vi "MIX11.1Eng.vi"() -> ()   [LabVIEW 2017]
uses:
  <vilib>/Utility/NIReport.llb/NI_report.lvclass
  <vilib>/Utility/NIReport.llb/Excel/NI_Excel.lvclass
  Instance           1 13Saved   MIX10 .vi
  Instance           5 13Saved   MIX10 .vi
  <vilib>/Utility/file.llb/Write To Spreadsheet File (string).vi
  <vilib>/Utility/file.llb/Read From Spreadsheet File (string).vi
  Instance           6 13Saved   MIX10 .vi
  <vilib>/Utility/NIReport.llb/Append Report Text (str wrap).vi
  <vilib>/Utility/NIReport.llb/Append Text Table to Report (wrap).vi
  Instance           4 13Saved   MIX10 .vi
  Instance           2 13Saved   MIX10 .vi
panel:
  in  "SP_Spurious":cluster{"Rx_output_data":path, "SAVE":bool}={"Rx_output_data"=path "L:/cartridge/assembly/SN03/03-23/111227_DSB/SP_810.00_120_111227_CCA03-23_DSBFB.csv", "SAVE"=TRUE}
  in  "report":refnum<class "NI_report.lvclass">=refnum
  in  "Offset":dbl
  in  "WCA Pol":u16(ring) items=["------------"=444, "WCA P0 S1"=0, "WCA P0 S2"=2, "WCA P1 S1"=1, "WCA P1 S2"=3]
  in  "VMax":dbl=5.0
  in  "Vmin":dbl
  out "VP Class":cluster{"”z—ñ":dbl[], "”z—ñ 2":dbl[]}={"”z—ñ"=[-1.0620880126953125, -1.0097503662109375, -0.9580230712890625, -0.9108734130859375, -0.8547210693359375, -0.803070068359375, -0.7555389404296875, -0.71075439453125, -0.659027099609375, -0.6090545654296875, -0.5593109130859375, -0.5091094970703125, -0.4544830322265625, -0.405120849609375, -0.3562164306640625, -0.3061676025390625, -0.25177001953125, -0.2005767822265625, -0.1529693603515625, -0.0995635986328125, -0.0360870361328125, 0.0032806396484375, 0.0568389892578125, 0.1003265380859375, 0.1499176025390625, 0.201416015625, 0.2490234375, 0.2971649169921875, 0.3517913818359375, 0.3971099853515625, 0.447845458984375, 0.4936981201171875, 0.5454254150390625, 0.59356689453125, 0.643768310546875, 0.6946563720703125, 0.7459259033203125, 0.7933807373046875, 0.8406829833984375, 0.8930206298828125, 0.94207763671875], "”z—ñ 2"=[0.0, 0.0, 0.0, 0.0, 0.0, 0.0, 0.0, 0.0, 0.0, 0.0, 0.0, 0.0, 0.0, 0.0, 0.0, 0.0, 0.0, 0.0, 0.0, 0.0, 0.0, 0.0, 0.0, 0.0, 0.0, 0.0, 0.0, 0.0, 0.0, 0.0, 0.0, 0.0, 0.0, 0.0, 0.0, 0.0, 0.0, 0.0, 0.0, 0.0, 0.0]}
  out "VI Class":cluster{"”z—ñ":dbl[], "”z—ñ 2":dbl[]}={"”z—ñ"=[-1.0620880126953125, -1.0097503662109375, -0.9580230712890625, -0.9108734130859375, -0.8547210693359375, -0.803070068359375, -0.7555389404296875, -0.71075439453125, -0.659027099609375, -0.6090545654296875, -0.5593109130859375, -0.5091094970703125, -0.4544830322265625, -0.405120849609375, -0.3562164306640625, -0.3061676025390625, -0.25177001953125, -0.2005767822265625, -0.1529693603515625, -0.0995635986328125, -0.0360870361328125, 0.0032806396484375, 0.0568389892578125, 0.1003265380859375, 0.1499176025390625, 0.201416015625, 0.2490234375, 0.2971649169921875, 0.3517913818359375, 0.3971099853515625, 0.447845458984375, 0.4936981201171875, 0.5454254150390625, 0.59356689453125, 0.643768310546875, 0.6946563720703125, 0.7459259033203125, 0.7933807373046875, 0.8406829833984375, 0.8930206298828125, 0.94207763671875], "”z—ñ 2"=[-8.428955078125, -7.815551757812501, -7.476806640625, -7.16552734375, -6.5887451171875, -6.0546875, -5.7098388671875, -5.682373046875, -5.18798828125, -4.4708251953125, -4.45556640625, -4.150390625, -3.375244140625, -3.167724609375, -2.40478515625, -2.4810791015625, -1.9561767578124998, -1.5899658203125, -1.0498046875, -0.4425048828125, -0.3448486328125, -0.0732421875, 0.1373291015625, 0.5889892578125, 1.1199951171875, 1.2298583984375, 1.715087890625, 1.9439697265625, 2.5054931640625, 2.9205322265625, 3.4698486328125, 3.50341796875, 3.96728515625, 4.2327880859375, 4.656982421875, 4.7698974609375, 5.230712890625, 5.7342529296875, 5.9234619140625, 6.439208984375, 6.9610595703125]}
  out "XY graph":cluster{dbl[], dbl[]}[](graph)=[{[0.9882354736328125], [1.4178466983139515]}, {[0.9882354736328125], [0.0]}, {[-1.0620880126953125, -1.0097503662109375, -0.9580230712890625, -0.9108734130859375, -0.8547210693359375, -0.803070068359375, -0.7555389404296875, -0.71075439453125, -0.659027099609375, -0.6090545654296875, -0.5593109130859375, -0.5091094970703125, -0.4544830322265625, -0.405120849609375, -0.3562164306640625, -0.3061676025390625, -0.25177001953125, -0.2005767822265625, -0.1529693603515625, -0.0995635986328125, -0.0360870361328125, 0.0032806396484375, 0.0568389892578125, 0.1003265380859375, 0.1499176025390625, 0.201416015625, 0.2490234375, 0.2971649169921875, 0.3517913818359375, 0.3971099853515625, 0.447845458984375, 0.4936981201171875, 0.5454254150390625, 0.59356689453125, 0.643768310546875, 0.6946563720703125, 0.7459259033203125, 0.7933807373046875, 0.8406829833984375, 0.8930206298828125, 0.94207763671875], [-8.428955078125, -7.815551757812501, -7.476806640625, -7.16552734375, -6.5887451171875, -6.0546875, -5.7098388671875, -5.682373046875, -5.18798828125, -4.4708251953125, -4.45556640625, -4.150390625, -3.375244140625, -3.167724609375, -2.40478515625, -2.4810791015625, -1.9561767578124998, -1.5899658203125, -1.0498046875, -0.4425048828125, -0.3448486328125, -0.0732421875, 0.1373291015625, 0.5889892578125, 1.1199951171875, 1.2298583984375, 1.715087890625, 1.9439697265625, 2.5054931640625, 2.9205322265625, 3.4698486328125, 3.50341796875, 3.96728515625, 4.2327880859375, 4.656982421875, 4.7698974609375, 5.230712890625, 5.7342529296875, 5.9234619140625, 6.439208984375, 6.9610595703125]}, {[-1.0620880126953125, -1.0097503662109375, -0.9580230712890625, -0.9108734130859375, -0.8547210693359375, -0.803070068359375, -0.7555389404296875, -0.71075439453125, -0.659027099609375, -0.6090545654296875, -0.5593109130859375, -0.5091094970703125, -0.4544830322265625, -0.405120849609375, -0.3562164306640625, -0.3061676025390625, -0.25177001953125, -0.2005767822265625, -0.1529693603515625, -0.0995635986328125, -0.0360870361328125, 0.0032806396484375, 0.0568389892578125, 0.1003265380859375, 0.1499176025390625, 0.201416015625, 0.2490234375, 0.2971649169921875, 0.3517913818359375, 0.3971099853515625, 0.447845458984375, 0.4936981201171875, 0.5454254150390625, 0.59356689453125, 0.643768310546875, 0.6946563720703125, 0.7459259033203125, 0.7933807373046875, 0.8406829833984375, 0.8930206298828125, 0.94207763671875], [0.0, 0.0, 0.0, 0.0, 0.0, 0.0, 0.0, 0.0, 0.0, 0.0, 0.0, 0.0, 0.0, 0.0, 0.0, 0.0, 0.0, 0.0, 0.0, 0.0, 0.0, 0.0, 0.0, 0.0, 0.0, 0.0, 0.0, 0.0, 0.0, 0.0, 0.0, 0.0, 0.0, 0.0, 0.0, 0.0, 0.0, 0.0, 0.0, 0.0, 0.0]}]
  in  "Controller":T1(tab)=enum."revision"
  in  "CAN reset":bool
  out "Connected":bool
  in  "DISConnect":bool
  in  "Connect":bool
  in  "Bias_LO_equip":T2={"Node address"=19, "CAN Interface"="CAN0", "Cartridge band"=8, "Slave Node in"={"Address"=19, "Serial Number"=[16, 121, 69, 76, 1, 8, 0, -31]}, "ObjHandle out"=26, "POL"=0, "sb"=1, "GPIB_SM (SIS S,V)"="24", "GPIB_DMM (SIS I)"="22", "GPIB_SM (MAG I) "="25", "GPIB_SG(LO)"="19", "GPIB_PW (PAMP) "="6", "GPIB_TMP1(8ch)"="12", "GPIB_TMP2(2ch)"="13", "WCA_avg"=10, "Rsen"=10.0, "BiasModule"=1, "LOModule "=2, "WCA_LO_FREQ_SET"={"YTO Low freq. [GHz]"=14.65, "YTO High freq. [GHz]"=17.5, "Kvco"=1, "Lock Pol."=0, "SET LO FREQ"=88.77778, "Multiplier"=6.0, "YTO (HEX)"=210, "YTO ( FREQ)"=14.796153, "NULL PLL INTEGRATOR"=TRUE}, "Res for"=0} {"Res for" items=["none", "series res", "parallel res"]; "WCA_LO_FREQ_SET"."YTO ( FREQ)" min=25 max=150 step=0.0001 format="%.3f"; "WCA_LO_FREQ_SET"."Multiplier" min=3 max=6 step=3; "WCA_LO_FREQ_SET"."SET LO FREQ" min=25 max=150 step=0.0001 format="%.3f"; "WCA_LO_FREQ_SET"."Lock Pol." items=["Lower", "Upper"]; "WCA_LO_FREQ_SET"."Kvco" items=["7.5MHz/V", "15MHz/V"]; "WCA_LO_FREQ_SET"."YTO High freq. [GHz]" format="%.3f"; "WCA_LO_FREQ_SET"."YTO Low freq. [GHz]" format="%.3f"; "BiasModule" items=["B10Lab Bias"=0, "WCA BiasModule"=1, "none"=99, "SM-4W"=2]; "Slave Node in"."Serial Number" format="%.0x"; "Slave Node in"."Address" format="%.0x"; "Cartridge band" max=10 step=1; "Node address" format="%.0x"}
  in  "Control":T3={"GPIB_ATT"="28", "6501Dev#"=1, "GPIB_SpecA"="18", "GPIB_PM"="13", "GPIB_DSA"="11", "GPIB_DMM (TPD)"="23", "MPI COM"="COM5", "motor setting"=[{"Axis"=0, "ID"=0, "HIspeed"=200.0, "LOspeed"=100.0, "ACCEL(ms)"=100.0, "Sratio"=50.0, "free run\n"=FALSE, "motor"="DSB HOT/COLD"}, {"Axis"=1, "ID"=0, "HIspeed"=4.0, "LOspeed"=4.0, "ACCEL(ms)"=100.0, "Sratio"=50.0, "free run\n"=TRUE, "motor"="SubMM Att"}, {"Axis"=0, "ID"=0, "HIspeed"=200.0, "LOspeed"=100.0, "ACCEL(ms)"=100.0, "Sratio"=50.0, "free run\n"=FALSE, "motor"="MPI Port1"}, {"Axis"=1, "ID"=0, "HIspeed"=200.0, "LOspeed"=100.0, "ACCEL(ms)"=100.0, "Sratio"=50.0, "free run\n"=FALSE, "motor"="MPI Port2"}, {"Axis"=1, "ID"=0, "HIspeed"=200.0, "LOspeed"=100.0, "ACCEL(ms)"=100.0, "Sratio"=50.0, "free run\n"=TRUE, "motor"="gainComp"}], "DATA path"=path "C:/", "mixer param file "=path "C:/", "comment"="150115_balanced_WCA_2", "Carteidge SN"="balanced150115", "Th"=297.0, "Tc"=77.0, "Set_SIS_volt"=1.0483870967741935, "Offset"=0.0, "control"=0, "FreqLO"=799.0, "Set_Mag_Cur"=0.0, "MPI offset(mm)"=23.203, "HOT/COLD"=0} {"HOT/COLD" items=["DSB", "SBR (Cart.)"]; "control" items=["CLOSE LOOP", "OPEN LOOP", "Not Control"]}
  in  "Additional Cartridge band":u32=10 max=10 step=1
  in  "add":bool
  in  "CLNA_SET":T4 {"SET POL0 LNA1 STAGE3 DRAIN C" min=0 max=20 step=0.01 format="%.2f"; "SET POL0 LNA1 STAGE3 DRAIN V" min=0 max=3 step=0.01 format="%.2f"; "SET POL0 LNA1 STAGE2 DRAIN C" min=0 max=20 step=0.01 format="%.2f"; "SET POL0 LNA1 STAGE2 DRAIN V" min=0 max=3 step=0.01 format="%.2f"; "SET POL0 LNA1 STAGE1 DRAIN C" min=0 max=20 step=0.01 format="%.2f"; "SET POL0 LNA1 STAGE1 DRAIN V" min=0 max=3 step=0.01 format="%.2f"; "CLNA State" items=["Disabled", "Enabled"]}
  out "CLNA_monitor":T5={"Pol0 LNA1 S1 Drain V [V]"=0.0017700195, "Pol0 LNA1 S1 Drain C [mA]"=0.0033569336, "Pol0 LNA1 S1 Gate V [V]"=-0.3663025, "Pol0 LNA1 S2 Drain V [V]"=0.0020446777, "Pol0 LNA1 S2 Drain C [mA]"=0.0010681152, "Pol0 LNA1 S2 Gate V [V]"=4.9404297, "Pol0 LNA1 S3 Drain V [V]"=0.0019989014, "Pol0 LNA1 S3 Drain C [mA]"=0.024871826, "Pol0 LNA1 S3 Gate V [V]"=4.940445, "Pol0 LNA1 State"=enum."Disabled"} {"Pol0 LNA1 S3 Gate V [V]" format="%.2f"; "Pol0 LNA1 S3 Drain C [mA]" format="%.2f"; "Pol0 LNA1 S3 Drain V [V]" format="%.2f"; "Pol0 LNA1 S2 Gate V [V]" format="%.2f"; "Pol0 LNA1 S2 Drain C [mA]" format="%.2f"; "Pol0 LNA1 S2 Drain V [V]" format="%.2f"; "Pol0 LNA1 S1 Gate V [V]" format="%.2f"; "Pol0 LNA1 S1 Drain C [mA]" format="%.2f"; "Pol0 LNA1 S1 Drain V [V]" format="%.2f"}
  in  "CLNA Monitor":bool=TRUE
  in  "Set CLNA":bool
  in  "Temp Monitor":bool=TRUE
  out "T3":dbl=-1.0
  out "T2":dbl=296.31982421875
  out "T1":dbl=-1.0
  in  "CLNAsweep":T6={"VDmin"=1.0, "VDmax"=2.0, "VDstep"=0.1, "IDmin"=8.0, "IDmax"=20.0, "IDstep"=1.0, "wait (mS)"=500.0, "P.M.aveg"=10, "HOT/COLD "=0, "SIS hotV "=8.0, "SIS coldV"=5.0, "file_name"="", "frq(GHz)"=8.0} {"HOT/COLD" items=["Liq Ni Motor", "SISBias"]}
  in  "CLNA Sweep":bool
  in  "Do shapiro":bool
  in  "Heater@ON@":bool
  in  "Do Demag":bool
  in  "Ic measurement":bool
  in  "demag":T7={"Start(mA)"=100.0, "Time(ms)"=200.0, "step"=1.0}
  in  "Joseph_curr":T8={"start(mA)"=8.5, "stop(mA)"=10.0, "step(mA)"=0.1, "file_name"="", "file path"=path "", "save?"=FALSE, "SIS Bias range Vsis"={"start"=-0.1, "stop"=0.1, "step"=0.02}}
  in  "Magnet Current Set":dbl(slide) scale=10.0..30.0
  in  "Mag Monitor":bool=TRUE
  out "Mag V":dbl=0.8539886474609375
  out "Mag C":dbl=26.22833251953125
  in  "shapiro":T9={"start(mA)"=8.5, "stop(mA)"=10.0, "step(mA)"=0.05, "start(mV)"=1.2, "stop(mV)"=2.4, "step(mV)"=0.05, "file_name"="", "path"=path "", "save?"=FALSE}
  in  "SIS_Deflux_heater":T10={"ON start time (ms)"=3000.0, "ON duration time (ms)"=10000.0, "Measurement end time"=60000.0, "SIS Volt (mV)"=0.5, "GPIB_PW (SISHeater) "="3", "SAVE"=TRUE, "file_name"="", "path"=path "Z:/band10/Labview_ALMA/MIX95/test"}
  in  "SISparam":bool
  in  "Zero Int":bool
  in  "Set LO PAMP":bool
  in  "WCA_LO monitor":bool=TRUE
  in  "LO_misc":T11={"LO FRQ(GHz)"=799.0, "LO multi "=9.0, "LocK?"=FALSE, "LO REF multi"=3.0, "wait (ms)"=100.0, "SG Pow Min (dBm)"=0.0, "SG Pow Max (dBm)"=20.0, "SG Pow Step (dBm)"=0.2, "SGPow OPT? "=TRUE, "SG set frq"=0.0, "SG set pow"=0.0}
  in  "Set LO freq":bool
  out "GET_PA":T12={"PA_A_DRAIN_V"=0.009918213, "PA_A_DRAIN_C"=2.4871826, "PA_A_GATE_V"=0.0016784668, "PA_B_DRAIN_V"=0.0077819824, "PA_B_DRAIN_C"=2.8533936, "PA_B_GATE_V"=0.004272461, "PA_3V_SUPPLY_V"=2.992859, "PA_5V_MON"=5.2355957}
  out "GET_PLL":T13={"PLL_ASSY_T"=29.312134, "PLL_REF_TOT_P"=-0.02670288, "PLL_IF_TOT_P"=-0.036315918, "PLL_CORR_V"=-3.8926976, "PLL_LOCK_V"=0.05389127, "PLL_5V_SUPPLY_V"=25.061035, "Temp_TF"=TRUE, "PLL Ref Pwr_TF"=FALSE, "IF Pwr_TF"=FALSE, "PLL Corr_TF"=FALSE, "PLL Lock V_TF"=FALSE, "PLL Nominal_TF"=FALSE}
  in  "PA V":cluster{"VD":dbl, "VG ":dbl, "String":string}[](array[cluster])=[{"VD"=0.0, "VG "=-0.4, "String"="WCA P0"}, {"VD"=0.0, "VG "=0.0, "String"="WCA P1"}, {"VD"=0.0, "VG "=0.0, "String"="B10 PAMP"}] {"VG" min=-1.0 max=4.0; "VD" min=0.0 max=2.5}
  in  "_LO_P_OPT":T14={"Range Array"=[{"Start"=0.0, "Stop"=3.5, "Step"=0.1, "By"="NEL VG"}, {"Start"=30.0, "Stop"=75.0, "Step"=1.0, "By"="Motor"}, {"Start"=0.5, "Stop"=2.0, "Step"=0.05, "By"="WCA VD"}], "Optimize"=0, "file_name"="LP_914.0_Tmin_100519.csv", "Save?"=FALSE, "measure"=2, "current(uA)"=40.0, "wait(ms)"=0, "IFfrq(GHz)"=8.0, "aveg"=10, "SISparam option"=0} {"SISparam option" items=["Volt and Current", "Volt only"]; "measure" items=["Pmax (only HOT)", "Tmin (HOT/COLD)", "C current"]; "Optimize" items=["Sweep", "‰©‹à•ªŠ„"]; "Range Array"."Step" format="%.2f"; "Range Array"."Stop" format="%.2f"; "Range Array"."Start" format="%.2f"}
  in  "LOP optimize":bool
  in  "_LO_sweep":T15={"scales"=200.0, "start (GHz)"=780.0, "stop (GHz)"=960.0, "step (GHz) "=0.1, "Wait(ms)"=10.0, "file_name"="", "path"=path "", "measure"=0, "WCA Pol"=0} {"WCA Pol" items=["------------"=444, "WCA P0 S1"=0, "WCA P0 S2"=2, "WCA P1 S1"=1, "WCA P1 S2"=3]; "measure" items=["SIS Current", "DMM34401A"]}
  in  "LO_SWEEP":bool
  in  "IFBOX":T16={" Output"=2, "YIG Fc(GHz)"=8.0, " Filter"=3, "Input"=2} {"Input" items=["1:Pol 0"=1, "2:Pol 1"=2, "3:dummy"=3, "4:NoiseSource"=4]; "Filter" items=["1:YIG"=1, "2:direct"=2, "3:4-12BPF"=3, "4:direct 4-12BPF"=4]; "Output" items=["1:Speana"=1, "2:PowerMeter"=2, "3:dummy"=3, "4:TPD"=4]}
  in  "I-V sweep":bool
  in  "i-v parameter":T17={"start(mV)"=0.0, "stop(mV)"=3.0, "step(mV)"=0.05, "file_name"="", "IF OFF/ON"=FALSE, "SAVE OFF/ON"=FALSE, "frq(GHz)"=8.0, "avg"=1, "number of Sweep  "=0, "VminfromSS"=0.15, "mode "=0, "V@opt"=2} {"mode" items=["voltage sweep", "every time HOT/COLD"]; "number of Sweep" items=["only once", "Hot/Cold_auto", "Hot/Cold manual"]}
  out "HOT":bool
  in  "HOT/COLD":bool=TRUE
  in  "IFBOXSet":bool
  in  "CrossTalk_mkpk":T18={"save"=TRUE, "file_name"="", "IF start"=4.0, "IF stop"=12.0, "IF step"=1.0}
  in  "CrossTalk":bool
  in  "GainComp":bool
  in  "GC_LockinAmp":T19={"GPIB"="28", "wait(s)"=10.0, "measure(s) "=30.0, "save"=FALSE, "time constant"=6, "file_name"=""} {"time constant" items=["100mS"=5, "300mS"=6, "1S"=7, "3S"=8, "10S"=9]}
  in  "allan":T20={"DMM Setting A"={"interval"=1.0, "sample number"=5000, "Voltage Range"=enum."1 V", "Factor"=1.0, "unit"=0, "Power supply freq. (Hz)"=50.0}, "Path"=path "c:/Data", "File name"="", "DMM"=0, "DSA_mes"={"GPIB_DSA"="11", "Startfrq(Hz)"=0.0, "Stopfrq(Hz)"=800.0, "Range(Vpk)"=1.0, "average"=4}, " temperature?"=TRUE, "time interval"=10.0} {"DMM" items=["DMM34410A", "34401A", "3458", "DSA35670A"]; "DMM Setting A"."unit" items=["Sec", "PLC"]; "DMM Setting A"."sample number" min=1 max=1000000 step=1}
  in  "Start allan":bool
  in  "LO harmonic":T21={"save"=TRUE, "file_name"="", "LO start"=890.0, "LO stop"=938.0, "LO step"=8.0, "IF"=5.0, "8th 10th"=TRUE}
  in  "LO Harmonic":bool
  in  "spectrum_data":T22={"total data num(1-3)"=2, "file_name"="", "SAVE OFF/ON"=FALSE, "ATT1"=0.0, "ATT2"=2.0, "SNAdatafile ATT1"=path "C:/Documents and Settings/band10/デスクトップ/Labview_ALMA/MIX99/101210_ATT/ATT0db.prn", "SNAdatafile ATT2"=path "C:/Documents and Settings/band10/デスクトップ/Labview_ALMA/MIX99/101210_ATT/ATT2db.prn", "ATTcal"=FALSE, "SP_set"={"start(GHz)"=3.5, "stop(GHz) "=12.5, "BW(MHz)"=8.0, "VBW(Hz)"=30.0, "ref(dBm)"=-50.0, "log(dB)"=1.0, "AVEG"=1, "AVEG ON/OFF"=FALSE, "Auto Align ON/OFF"=FALSE, "GPIB"="18", "point"=1126}, "HOT/COLD"=1} {"HOT/COLD" items=["Manual", "Motor auto", "SIS V", "P0/P1", "single data"]}
  in  "SPmeasuremnt":bool
  in  "Noise_YIG_tune_filter_control":T23={"Start(GHz)"=4.0, "Stop(GHz)"=12.0, "Step(GHz) "=0.1, "wait (S)"=0.0, "Hot/Cold Switch"=1, "file_name"="", "P.M.aveg"=10, "save"=TRUE} {"Hot/Cold Switch" items=["Liq Ni Motor", "NoiseSource Pow", "NoiseSource SP4T SW"]}
  in  "YIG measurement":bool
  in  "RF":bool
  in  "Move MPI toSSB":bool
  in  "IF frequency to SSB":dbl=4.0 format="%#.5g"
  in  "SBR":bool
  out "MPI present location":string="22.99999\r\n"
  in  "MPI pos":dbl=23.0 format="%#.5g"
  in  "MPI-I":bool
  in  "MPI_I":T24={"wait(ms)"=300, "Start"=22.5, "Stop"=23.5, "Step"=0.005, "save"=TRUE, "file_name"=""} {"Step" format="%#.6f"; "Stop" format="%.2f"; "Start" format="%.2f"}
  in  "Move MPI":bool
  in  "SBR_Set":T25={"file_name"="", "HOT/COLD AUTO"=TRUE, "MPI SSB Set"=TRUE, "Waiting time at AUTO(S)"=0.1, "P/V         V/P"=TRUE, "save"=TRUE, "start(GHz)"=4.0, "stop(GHz) "=12.0, "Step(GHz) "=0.5, "P.M.aveg"=10, "PM        SP"=FALSE, "SP_set"={"start(GHz)"=3.5, "stop(GHz) "=12.5, "BW(MHz)"=8.0, "VBW(Hz)"=30.0, "ref(dBm)"=-45.0, "log(dB)"=1.0, "AVEG"=1, "AVEG ON/OFF"=FALSE, "Auto Align ON/OFF"=FALSE, "GPIB"="18", "point"=801}}
  in  "RF":T26={"RF(GHz)"=900.0, "mm_multi(4or6)"=6.0, "SGPOUT(dBm)"=16.0, "SGGPIB"="29", "PAMP GPIB"="6", "VD (V)"=1.0, "VG (V)"=0.0, "multi (V)"=8.0} {"multi (V)" min=0.0 max=15.0 step=0.5; "VG (V)" min=0.0 max=4.0 step=0.1; "VD (V)" min=0.0 max=1.85 step=0.01}
  out "file name":string="mix11_baranced_setmix.txt"
  in  "MOSL":i32
  out "log_refnum":refnum<file>
  in  "Script path":path=path "C:/Labview_ALMA/MIX11/Mixスクリプト"
  in  "?":enum32{"run", "save"}(tab)
  in  "load script":bool
  in  "run script":bool
  in  "save":bool
  in  "program":cluster{"Cord":u16, "Option":string}[](array[cluster])=[{"Cord"=1, "Option"="auto measurement By WCA LO 2Pol"}, {"Cord"=16, "Option"=""}, {"Cord"=130, "Option"="0"}, {"Cord"=15, "Option"="モータ位置確認"}, {"Cord"=1, "Option"="LOあり"}, {"Cord"=17, "Option"="ファイル名に付加するコメント入力,%COM%"}, {"Cord"=13, "Option"="-9999"}, {"Cord"=21, "Option"=""}, {"Cord"=284, "Option"=""}, {"Cord"=25, "Option"=""}, {"Cord"=302, "Option"=""}, {"Cord"=25, "Option"=""}, {"Cord"=302, "Option"=""}, {"Cord"=25, "Option"=""}, {"Cord"=1, "Option"=""}, {"Cord"=2, "Option"="794,938,8"}, {"Cord"=31, "Option"="_setmix_LO_IV_SP_mes_baranced_s1.txt,dummy"}, {"Cord"=3, "Option"=""}, {"Cord"=1, "Option"="LOをフリーランに"}, {"Cord"=121, "Option"="799,0"}, {"Cord"=1, "Option"="P0 LO　LOなしIV測定"}, {"Cord"=112, "Option"="0,2.1"}, {"Cord"=103, "Option"="1"}, {"Cord"=125, "Option"="0.8,0"}, {"Cord"=103, "Option"="0"}, {"Cord"=215, "Option"="780,960,0.1,0"}, {"Cord"=1, "Option"=""}, {"Cord"=103, "Option"="1"}, {"Cord"=125, "Option"="0,0"}, {"Cord"=103, "Option"="0"}, {"Cord"=221, "Option"="1,8,1,0,-10,10,0.1,aNOLO"}, {"Cord"=221, "Option"="1,8,1,0,0,5,0.01,aNOLOs"}, {"Cord"=103, "Option"="1"}, {"Cord"=221, "Option"="1,8,1,0,-10,10,0.1,aNOLO"}, {"Cord"=221, "Option"="1,8,1,0,0,5,0.01,aNOLOs"}, {"Cord"=114, "Option"="0"}, {"Cord"=103, "Option"="0"}, {"Cord"=114, "Option"="0"}, {"Cord"=221, "Option"="1,8,1,0,0,5,0.01,aNOLO_MAGs"}, {"Cord"=103, "Option"="1"}, {"Cord"=221, "Option"="1,8,1,0,0,5,0.01,aNOLO_MAGs"}, {"Cord"=103, "Option"="1"}, {"Cord"=31, "Option"="_cart_dsb_QL_post.txt,dummy"}, {"Cord"=22, "Option"=""}, {"Cord"=4, "Option"=""}] {"Cord" items=["//"=1, "LOOP"=2, "NEXT"=3, "END"=4, "set loop num"=5, "jump"=6, "-"=10001, "wait"=11, "beep"=12, "comment"=13, "cartSN"=14, "Pause"=15, "Selecr Dir"=16, "Text Input"=17, "--"=10008, "Open Log"=21, "Close Log"=22, "Write Log"=25, "comment form Log"=27, "filename to Log"=28, "CALL"=31, "-----"=10002, "equip"=102, "Pol"=103, "LO_para"=105, "-------"=10004, "SIS V"=112, "SIS offset"=113, "IMAG"=114, "CLNA"=115, "----"=10003, "LOFREQ"=121, "dummyLO"=122, "LOPAMP"=125, "LO GUNN set"=127, "--------"=10005, "Morotr Reset"=130, "Move Mortor"=135, "---------"=10006, "IFBOX"=140, "IFOBOX SW"=145, "IFBOX BPF"=147, "IFBOX ATT"=148, "----------"=10007, "LOP opt"=210, "LO Sweep"=215, "I-V"=220, "I-V(NOLO)"=221, "I-V Trx"=225, "I-V Trx2"=226, "SP"=230, "YIG"=240, "SBR"=250, "Allan"=260, "GainComp"=270, "Cross talk"=275, "Harmonics"=278, "Read-PM_Temp"=281, "Read-WCA_Temp"=282, "Bias_Helth_check"=283, "MIX10 params"=284, "shapiro"=290, "demag"=292, "defluxHTR"=293, "JC"=294, "-----------"=10009, "ReadMixParam"=301, "ReadCLNAParam"=302, "ReadLOParam"=303, "SetMixParam"=311, "SetCLNAParam"=312, "SetLOParam"=313, "SetMixParam_V"=314, "select mixerParam"=320, "--------------"=10010, "excel open "=401, "excel save"=402, "excel close"=403, "open sheet"=404, "set cell "=405, "set 2D data"=406, "excel window"=407, "make file name"=410, "File Time Stamp"=411, "read 2D data"=412, "choice 2D"=414, "Calc IF output"=450, "SPsprious"=451, "make 3D graph"=460]}
  in  "MOS":T27(array[cluster])=[{"run number"=44, "number of lines"=45, "option"="", "Lupu's numerical value"=938.0, "Lupe Stop"=938.0, "Lupe Step"=8.0, "Line number"=15}, {"run number"=14, "number of lines"=15, "option"="", "Lupu's numerical value"=938.0, "Lupe Stop"=938.0, "Lupe Step"=8.0, "Line number"=15}, {"run number"=23, "number of lines"=24, "option"="", "Lupu's numerical value"=794.0, "Lupe Stop"=938.0, "Lupe Step"=8.0, "Line number"=15}, {"run number"=0, "number of lines"=0, "option"="", "Lupu's numerical value"=946.0, "Lupe Stop"=946.0, "Lupe Step"=8.0, "Line number"=10}, {"run number"=0, "number of lines"=0, "option"="", "Lupu's numerical value"=946.0, "Lupe Stop"=946.0, "Lupe Step"=8.0, "Line number"=10}, {"run number"=0, "number of lines"=0, "option"="", "Lupu's numerical value"=946.0, "Lupe Stop"=946.0, "Lupe Step"=8.0, "Line number"=10}]
  in  "Buffer":string="SP__matrix_data10_121_150115_balanced_WCA_2m.csv.plt.png" caption="バッファ"
  out "revision":string="2018 8/8 Translate Japanese to English\n\n2017 Mix11 English Record support\n\n2013 6/13 LOHarmonics to script\n\n2013 5/25 GC file completed after measurement\n\n2012 8/15 JC ªÈ£Í£á£çªÎ«Õ?«¤«ëÙ£ªË£Ì£Ïñ²÷î?\n2012 8/15 £Ê£ÃªÈ£É£í£á£çªÎ«Õ?«¤«ëÙ£ªË£Ì£Ïñ²÷î?ªòìýªìªÊª¤\n\n\n2012?7/10 £É£Ö??£Õ£Ô£Ï£³ªÎª·ªçªÔªíï³?ªòàâïÒÊ¦?ªË«Ç«Õ«©«ë«ÈªÏ0.2ªËª·ªÆªªª­£Ö£ç£á£ðªÎî¸ª¤ªâªÎªÏ0.15ªËª¹ªë¡£\n£Ì£Ï£Ï£Ð£ÔªÎ?ÑÑÝÂùÜªÀªÈ?ðà?Ê¥ª·ªÊª¤ãÁªËÙýð¹ª¢ªê¡¢£Ã£Ã?07?11ö´ïÒãÁ?ª·ªÐªéª¯ª¹ª¤?ª×ªÇ£Ó£É£Ó£Â£é£á£ó«»«Ã«Èª¹ªë¡£\n£Ç£Ã«×«í«°«é?ªÇö´ïÒüÞ?3üÞì¤ß¾ªÇ?ªáªëÝ»ÝÂªÎ÷÷?ªòªÁªçªÃªÈ?ª¨ªë\n\n\n2012 3/14 IV-auto3ªÇª·ªãªÔªíï³?£°£®£²£í£Öì¤ß¾£½£¾£°£®£±£µ£í£Öì¤ß¾ªË?ÌÚ\n£¨ñ²÷î?ªÎÍÔª¤ªÈª³ªíªÇó¬ª¬ÓÞª­ª¹ª®ªë£©\n\n2012 3/2  WCAPOLªÞªïªêáóïá£¨£Ä£Ó£Â«â?«ÉªÀª±ªËª·ª¿£©\n\n\n2012 2/10 ?«Ò??Ö§?£Ï£îûù\n\n2012 1/26 «¹«¯«ê«×«È?£Ì£Ï£Ð£á£ò£á£íªË£Ð£Ï£ÌªòõÚÊ¥\n???????£Ð£Ï£Ìªò?ÌÚª·ª¿ªÈª­ªË£Ã£ï£î£ô£ò£ï£ìªÎ£Ó£å£ô£Ó£É£Ó£Ö£Ï£Ì£ÔÔõªËÚãç±?\n\n2012 1/18  SBRÍªß©?ÊÛæ¶SBRªòõÚÊ¥\n\n2012 1/9 «¹«¯«ê«×«È?Text Inputáóïá¡¢ôøÑ¢ö·ª¬ù±é©ªË\n???????????Cartridge SNõÚÊ¥\n\n2012 1/8 «¹«¯«ê«×«È?FileTimeStampõÚÊ¥\n\n2012 1/7  «¹«¯«ê«×«È?SP spriousõÚÊ¥\n\n2012?1/7  Calc IF?outªÎ«¯«é«¹?ªÇNS£ßENRªÎ«Ç«£«ì«¯«È«êªò\nInputCable¡¢NS_AMPªÎ«Ç«£«ì«¯«È«êªËª¹ªëªèª¦ªË?ÌÚ£¨ú°à°«Ñ?«³«ó¡¢IFBOXª¬?ªïªÃª¿ãÁªËNS_ENRªÀª±àÔ?ª·ªÊªªª¹£©\n        \n\n2011 11/20 LO Harmonic  õÚÊ¥?CrossTalkªÇSIS«Ð«¤«¢«¹ªò£µ£íVªË\n\n2011 11/14 «¹«¯«ê«×«ÈPolÞÅéÄãÁªËWCAPolªâÌÚãæª¹ªëªèª¦ªËª·ª¿\n\n2011 11/05 CLNA«Ð«¤«¢«¹«¹«¤?«×¡¢ª¤ªÃª¿ªó£°V£°MAªËª¹ªë\n??????«¹«¯«ê«×«ÈExcel?Set?CellªÏ£°£¬£°ª¬A1?£¨ì¤îñíÂà÷ª·ª¿«¹«¯«ê«×«ÈªÏìéËÁªºªÄá´ªÊª¯ª¹ªë£©\n\n2011 11/04 Labview2011 ver «ì??«ÈíÂà÷«Ä?«ëÞÅéÄ\n\n2011 10/29  «¹«¯«ê«×«È?SetcellªËPolõÚÊ¥?Make3DªÎ«Õ?«¤«ëÙ£áóïá\n\n2011 10/25?«¹«¯«ê«×«È?Mix10ParamsªË«¹«¯«ê«×«È«Õ?«¤«ëÙ£õÚÊ¥ \n\n2011 10/14 «¹«¯«ê«×«ÈPolSetªÎªÈª­ôøÑ¢ö·ª«ªéSetMagÔõªò?ÌÚ\n????PM?TEMP?PolªË«¹«Ú?«¹ð¶ËÛ\n????LOParamsªò?PAA?PABªÎ?ªÓª«ªéP0?P1ªÎªÊªéªÓªË¡¢ª½ªÎý­ªÎWCA«Ñ«é«á??ªÏPAA?PABªÎ?ªÓ\n\n2011 10/02 «¹«¯«ê«×«ÈSetcell áóïá?make3Ddataªâáóïá£¨«Ç??«Ç«£«ì«¯«È«êªË?ßÀªòÜÁðí£©\n\n2011 9/28?«¹«¯«ê«×«ÈSP?ÌÚ?VBWªâàâïÒÊ¦?ªË\n \n2011 9/26 SP single dataªÉªê¡¢«¹«¯«ê«×«ÈªËpoint comment2õÚÊ¥\n \n\n2011 9/9 2pol ö´ïÒéÄªË«¹«¯«ê«×«ÈìéÝ»áóïá\n\n2011 9/8 control ªÎDB«Ñ«¹ªòmixer param ªË?ÌÚ\n\n2011 9/7 «¹«¯«ê«×«ÈMake£³DgraphíÂà÷\n\n2011 8/31 SIS setªÎªÈª­ªËPAVÛÕÖªªòÌÚãæ?SISï³??OffsetªâÌÚãæ\n\n2011 8/26 \n¡ÜLO PAMP?ªÈ ?£Ã£Ì£Î??ªÏ£×£Ã?ªÎãÁ£Ð£°£¬£Ð£±ªÈªâªËàâïÒ\n¡ÜBias_LO_equip LOModuleªËÊ¦?£Ì£Ï?£Ô£Ôªâùßªáªëª³ªÈªËª·ª¿ªÎªÇ¡¢\n£Ì£Ï?£Ï£Ð£Ô?Ìõªòáóïá \n¡Ü£Ã?£Î«ê«»«Ã«È?õÚÊ¥ \n\n2011 8/3 «¹«¯«ê«×«ÈªÇ«Õ«é«Ã«¯«¹?Ìõ\n????CAN«Î?«ÉªËMIX10paramsì£?ÌÚ\n\n2011 7/28  «¹«¯«ê«×«ÈªË«·«ã«Ô«í?Ìõ?«Õ?«¤«ëÙ£ªòLogªËßöª¯«³?«ó«ÉõÚÊ¥\n2011 7/27  «·«ã«Ô«í?Ìõáóïá¡¢í»ÔÑûù\n\n2011 7/6 «¨«¯«»«ë?Ìõáóïá\n2011 7/5 ª¤ª¯ªÄª«áóïá\n\n2011 7/1 Calc IF output ?Ö§?õÚÊ¥\n\n2011 6/29 Cross Talk õÚÊ¥\n\n2011 6/21 MPIð¤åÙªòGPIBªÇú¼ªÃªÆª¤ª¿ªé«¨«é?Òý?ªÊªÎªÇRS-232CªÇð¤åÙª¹ªëªèª¦ªËª·ª¿\n\n\n2011 6/18 «¹«¯«ê«×«È?«¨«¯«»«ë?Ìõ\n                                 ìé?jump«³?«ó«ÉõÚÊ¥\n\n2011 6/16  «¹«¯«ê«×«È?fileÙ£ªò«µ«Ö£Ö£éûù\n\n2011 6/12 «¹«¯«ê«×«È?set loop num\n2011 6/12 «¹«¯«ê«×«È?LO Sweep\n\n2011 5/15 «¹«¯«ê«×«ÈLOPOPT?Read LO param??ÌõíÂà÷\n\n2011 5/13 WCA LO??ªÇ«³«ó«È«í?«ëª·ª¿ªÈª³ªíªÎ?×âáóïá\n\n2011 4/28 RoomTemp Helth check \n               SPªâP£°?P1ï·ªêôðª¨ªÇ«Ç??ªòªÈªëªèª¦ªËáóïá\n\n2011?02?15?YIGSave«Õ«©??«Ã«È?ÌÚ\n\n2011/02/6  SetMixerParamõÚÊ¥\n\n\n2011/02/4 GainCompõÚÊ¥ Read MixCLNAParamõÚÊ¥?£¨LOªÏªÞªÀ£©\n \n2011/01/27 «¹«¯«ê«×«È«µ«Ö«×«í«°«é?áóïá\n\n2011/01/20 IFBOXñ²ªêªòáóïá\n\n2011 1/12 Mix10ªË?ÌÚ?«¹«¯«ê«×«È?«µ«Ö«¹«¯«ê«×«È?\n\n12/10 «¹«¯«ê«×«ÈLO«»«Ã«ÈªÎáóïá «â??«ê«»«Ã«È\n\n10/17 «¹«¯«ê«×«ÈªËAllan6£¨?Óø«Ç??ö¢Ôð£©õÚÊ¥?\n\n10/3 SPªËSISVªÇªÎH/CõÚÊ¥\n\n9?7?PLL?GUNNªÄª¤ª«\n\n9/4 YIGõÚÊ¥\n\n8/29 ControlªËHOT/COLDªòõÚÊ¥¡¢SBRö´ïÒãÁªÇªâIVSPDSB?ëåö´ïÒ\n\n8/24 MPIðÚªß?ªß\n\n8/13 WCA LO?Ö§?YTO?ªßö¢ªêáóïá¡¢Lock«ë??«óªÎÌ¸òÁª·£¨IFPªòõÌîêûùª·ªÆª«ªéLock£©\n\n8/12 CANôøÑ¢ûù«¨«é?ãÁªÎ?×âªò?ûù£À««?«È«ê«Ã«¸\n«¤«Ù«ó«È«¹«È«é«¯?«ãªòÓÞøëïÚ×â\n\n\n8/11 LOPOPT ªÎTCTHªòControlª«ªéªË?ÌÚ\n????«¹«¯«ê«×«ÈLOFreqGUNNªÇñ²÷î?ªòControlªË\n\n8/9 «¹«¯«ê«×«ÈªËIVNOLOªòõÚÊ¥¡¢Log«Õ?«¤«ëªËCommentªòªÄª±ªëªèª¦ªË£À?«¯«µö´ïÒÍ§\n\n8/6 «·«ã«Ô«í«¹«Æ«Ã«×«×«í«°«é?¡¢ª¤ªÃª¿ªó0ªË«»«Ã«Èª¹ªëªÈªèª¤Êïª¸£¿£À?«¯«µö´ïÒ\n«·«ã«Ô«í«¹«Æ«Ã«×«×«í«°«é?ÊÛæ¶÷úIF£ðªÎªßö´ïÒªÇ\n\n8/5  8/4áóïáÝÂªÎ«Ð«°áóïá£À?«¯«µö´ïÒ\n?LOSWEEPªÎB10LabãÁªÎ«Õ?«¤«ëÜÁðíáóïá\n\n8/4 IV-TrxªÇö´ïÒý­õÌî¸?ëå?ÓøªËVset\nContorolªËoffseÔõªÎõÚÊ¥IVª«ªéVsetÔõªÎÞûð¶\n\n\n8/2 «Ð«¤«¢«¹«â«¸«å?«ëôøÑ¢ûùªÎ«Ð«°áóïá\n?\n\n\n\n7/31\n?I-V«¹«¤?«×ªÎStartªÇ0.5sÜÁò¥\n?«¹«¯«ê«×«ÈªÇªÎö´ïÒªÇªÏ?ãÆ«Ñ«Í«ëªòÌÚãæª·ªÊª¤£¨«Õ?«¤«ëÙ£?óþ£©\n?«¹«¯«ê«×«È«í«°«Õ?«¤«ë\n?Bias«â«¸«å?«ë?LO«â«¸«å?«ëª¬ªÊª¤íÞùê99ªÇôøÑ¢ûù«â«Ë?ªòú¼ªïªÊª¤\n?SUB«×«í«°«é?ªÇªÏÚ±?óþ¡¢«¹«¯«ê«×«È«Ç«Ð«Ã«°éÄ\n\n\n7/30 \n?«Ò???ð¤åÙªÇ«Õ?«¤«ëÜÁðíõÚÊ¥\n£À««?«È«ê«Ã«¸\n\n7£®27?\n?yig?ãá?ñ²÷î?àâïÒõÚÊ¥¡¹?\n?GetSIS ªÎB10«Ð«¤«¢«¹\n£À?«¯«µö´ïÒÍ§"
  out "Detected CAN Nodes.":string="Program running.\nDo not turn off power to CAN nodes.\n\r\rCAN node with adress x13 found at Node index 00\rS/N: 10 79 45 4C 01 08 00 E1\r----------\r\r\nAMBSI CAN Library V1.1.2\r\nAMBSI Firmware V1.0.1\r\nFEMC Firmware V2.5.0\r\nFPGA V2.1.0\r\n10 F2 B3 58 2 8 0 1B\r\n1 21 C8 4F 14 0 0 E\r\n1 29 B5 5B 15 0 0 B3\r\n1 1F B 5C 15 0 0 87\r\n23 9B DE 4C 1 0 0 44\r\n0 0 0 0 0 0 0 0\r\n"
  in  "Controller 2":T28(tab)=enum."Page 2"
  in  "2D data":string[][](array[string])=[["-3.554E+0", "-314.008E+0", "-3.554E+0", "-314.120E+0", "-19.809E+0", "-21.049E+0", "563.916E+0", "-3.500E+0"], ["-3.510E+0", "-309.573E+0", "-3.510E+0", "-309.393E+0", "-19.811E+0", "-21.039E+0", "570.748E+0", "-3.450E+0"], ["-3.457E+0", "-305.008E+0", "-3.462E+0", "-305.002E+0", "-19.805E+0", "-21.029E+0", "573.442E+0", "-3.400E+0"], ["-3.418E+0", "-300.302E+0", "-3.406E+0", "-300.198E+0", "-19.795E+0", "-21.013E+0", "576.702E+0", "-3.350E+0"], ["-3.351E+0", "-295.950E+0", "-3.357E+0", "-295.618E+0", "-19.800E+0", "-21.011E+0", "581.317E+0", "-3.300E+0"], ["-3.306E+0", "-291.183E+0", "-3.307E+0", "-291.260E+0", "-19.807E+0", "-21.026E+0", "576.053E+0", "-3.250E+0"], ["-3.256E+0", "-286.865E+0", "-3.256E+0", "-286.792E+0", "-19.798E+0", "-21.026E+0", "570.840E+0", "-3.200E+0"], ["-3.197E+0", "-282.147E+0", "-3.212E+0", "-282.135E+0", "-19.812E+0", "-21.018E+0", "584.866E+0", "-3.150E+0"], ["-3.147E+0", "-277.560E+0", "-3.148E+0", "-276.825E+0", "-19.805E+0", "-21.014E+0", "582.408E+0", "-3.100E+0"], ["-3.099E+0", "-273.331E+0", "-3.099E+0", "-273.276E+0", "-19.806E+0", "-21.022E+0", "578.002E+0", "-3.050E+0"], ["-3.055E+0", "-269.608E+0", "-3.055E+0", "-269.714E+0", "-19.803E+0", "-21.006E+0", "586.259E+0", "-3.000E+0"], ["-3.002E+0", "-265.839E+0", "-3.003E+0", "-265.436E+0", "-19.807E+0", "-21.003E+0", "590.949E+0", "-2.950E+0"], ["-2.951E+0", "-261.908E+0", "-2.958E+0", "-261.768E+0", "-19.785E+0", "-20.989E+0", "585.905E+0", "-2.900E+0"], ["-2.895E+0", "-257.721E+0", "-2.905E+0", "-257.855E+0", "-19.786E+0", "-20.966E+0", "601.188E+0", "-2.850E+0"], ["-2.867E+0", "-254.266E+0", "-2.855E+0", "-254.358E+0", "-19.762E+0", "-20.925E+0", "612.705E+0", "-2.800E+0"], ["-2.808E+0", "-251.022E+0", "-2.801E+0", "-250.812E+0", "-19.735E+0", "-20.878E+0", "626.954E+0", "-2.750E+0"], ["-2.757E+0", "-247.894E+0", "-2.758E+0", "-247.897E+0", "-19.737E+0", "-20.882E+0", "625.252E+0", "-2.700E+0"], ["-2.711E+0", "-244.705E+0", "-2.709E+0", "-244.794E+0", "-19.851E+0", "-21.027E+0", "604.353E+0", "-2.650E+0"], ["-2.661E+0", "-240.149E+0", "-2.661E+0", "-240.082E+0", "-19.996E+0", "-21.280E+0", "538.095E+0", "-2.600E+0"], ["-2.613E+0", "-230.112E+0", "-2.616E+0", "-230.020E+0", "-20.061E+0", "-21.387E+0", "515.449E+0", "-2.550E+0"], ["-2.572E+0", "-206.451E+0", "-2.575E+0", "-207.053E+0", "-20.066E+0", "-21.403E+0", "509.446E+0", "-2.500E+0"], ["-2.540E+0", "-165.112E+0", "-2.538E+0", "-166.498E+0", "-20.065E+0", "-21.417E+0", "502.085E+0", "-2.450E+0"], ["-2.504E+0", "-111.349E+0", "-2.492E+0", "-110.480E+0", "-20.099E+0", "-21.398E+0", "529.610E+0", "-2.400E+0"], ["-2.427E+0", "-71.350E+0", "-2.433E+0", "-71.573E+0", "-20.173E+0", "-21.394E+0", "575.302E+0", "-2.350E+0"], ["-2.366E+0", "-59.100E+0", "-2.363E+0", "-59.076E+0", "-20.270E+0", "-21.328E+0", "692.159E+0", "-2.300E+0"], ["-2.313E+0", "-54.916E+0", "-2.306E+0", "-54.791E+0", "-20.304E+0", "-21.099E+0", "979.692E+0", "-2.250E+0"], ["-2.262E+0", "-52.783E+0", "-2.266E+0", "-52.924E+0", "-20.121E+0", "-20.640E+0", "1.602E+3", "-2.200E+0"], ["-2.204E+0", "-51.346E+0", "-2.216E+0", "-51.678E+0", "-19.789E+0", "-20.108E+0", "2.729E+3", "-2.150E+0"], ["-2.159E+0", "-50.983E+0", "-2.160E+0", "-51.157E+0", "-19.492E+0", "-19.694E+0", "4.395E+3", "-2.100E+0"], ["-2.108E+0", "-49.966E+0", "-2.108E+0", "-50.101E+0", "-19.268E+0", "-19.396E+0", "7.101E+3", "-2.050E+0"], ["-2.061E+0", "-49.182E+0", "-2.066E+0", "-49.487E+0", "-19.106E+0", "-19.208E+0", "8.906E+3", "-2.000E+0"], ["-2.004E+0", "-48.468E+0", "-2.001E+0", "-48.553E+0", "-18.970E+0", "-19.059E+0", "10.000E+3", "-1.950E+0"], ["-1.958E+0", "-48.276E+0", "-1.961E+0", "-47.842E+0", "-18.825E+0", "-18.930E+0", "8.683E+3", "-1.900E+0"], ["-1.918E+0", "-47.705E+0", "-1.908E+0", "-47.815E+0", "-18.499E+0", "-18.583E+0", "10.000E+3", "-1.850E+0"], ["-1.853E+0", "-47.379E+0", "-1.861E+0", "-47.388E+0", "-18.176E+0", "-18.121E+0", "0.000E+0", "-1.800E+0"], ["-1.806E+0", "-46.896E+0", "-1.827E+0", "-46.741E+0", "-18.721E+0", "-18.971E+0", "3.522E+3", "-1.750E+0"], ["-1.756E+0", "-46.344E+0", "-1.754E+0", "-46.112E+0", "-18.464E+0", "-18.508E+0", "10.000E+3", "-1.700E+0"], ["-1.705E+0", "-45.749E+0", "-1.705E+0", "-45.651E+0", "-18.152E+0", "-18.113E+0", "0.000E+0", "-1.650E+0"], ["-1.659E+0", "-45.465E+0", "-1.659E+0", "-45.422E+0", "-18.533E+0", "-18.638E+0", "8.712E+3", "-1.600E+0"], ["-1.597E+0", "-44.727E+0", "-1.601E+0", "-44.147E+0", "-18.764E+0", "-18.844E+0", "10.000E+3", "-1.550E+0"], ["-1.551E+0", "-44.458E+0", "-1.559E+0", "-44.321E+0", "-18.835E+0", "-18.904E+0", "10.000E+3", "-1.500E+0"], ["-1.503E+0", "-44.202E+0", "-1.506E+0", "-43.933E+0", "-18.891E+0", "-18.952E+0", "10.000E+3", "-1.450E+0"], ["-1.467E+0", "-43.820E+0", "-1.452E+0", "-43.329E+0", "-18.965E+0", "-19.027E+0", "10.000E+3", "-1.400E+0"], ["-1.407E+0", "-43.127E+0", "-1.406E+0", "-42.612E+0", "-19.096E+0", "-19.160E+0", "10.000E+3", "-1.350E+0"], ["-1.363E+0", "-42.645E+0", "-1.364E+0", "-42.596E+0", "-19.299E+0", "-19.387E+0", "10.000E+3", "-1.300E+0"], ["-1.311E+0", "-41.809E+0", "-1.314E+0", "-41.873E+0", "-19.568E+0", "-19.707E+0", "6.482E+3", "-1.250E+0"], ["-1.258E+0", "-40.463E+0", "-1.265E+0", "-41.077E+0", "-19.882E+0", "-20.115E+0", "3.780E+3", "-1.200E+0"], ["-1.213E+0", "-39.981E+0", "-1.206E+0", "-39.725E+0", "-20.175E+0", "-20.616E+0", "1.917E+3", "-1.150E+0"], ["-1.161E+0", "-38.474E+0", "-1.160E+0", "-38.229E+0", "-20.320E+0", "-21.025E+0", "1.129E+3", "-1.100E+0"], ["-1.110E+0", "-35.971E+0", "-1.108E+0", "-35.672E+0", "-20.305E+0", "-21.236E+0", "810.934E+0", "-1.050E+0"], ["-1.066E+0", "-31.772E+0", "-1.054E+0", "-31.656E+0", "-20.249E+0", "-21.305E+0", "693.471E+0", "-1.000E+0"], ["-1.000E+0", "-25.909E+0", "-1.012E+0", "-27.249E+0", "-20.204E+0", "-21.339E+0", "632.670E+0", "-950.000E-3"], ["-957.565E-3", "-22.900E+0", "-962.677E-3", "-22.787E+0", "-20.190E+0", "-21.328E+0", "630.777E+0", "-900.000E-3"], ["-910.873E-3", "-20.010E+0", "-912.781E-3", "-19.965E+0", "-20.151E+0", "-21.233E+0", "671.863E+0", "-850.000E-3"], ["-855.408E-3", "-18.329E+0", "-863.190E-3", "-18.423E+0", "-19.963E+0", "-20.915E+0", "788.553E+0", "-800.000E-3"], ["-805.893E-3", "-17.474E+0", "-797.577E-3", "-16.693E+0", "-19.631E+0", "-20.449E+0", "948.323E+0", "-750.000E-3"], ["-753.937E-3", "-16.397E+0", "-756.149E-3", "-16.562E+0", "-19.415E+0", "-20.143E+0", "1.088E+3", "-700.000E-3"], ["-706.635E-3", "-15.799E+0", "-709.305E-3", "-16.281E+0", "-19.334E+0", "-20.079E+0", "1.060E+3", "-650.000E-3"], ["-659.866E-3", "-15.152E+0", "-660.858E-3", "-15.347E+0", "-19.358E+0", "-20.133E+0", "1.011E+3", "-600.000E-3"], ["-610.886E-3", "-14.783E+0", "-606.995E-3", "-14.621E+0", "-19.409E+0", "-20.217E+0", "961.275E+0", "-550.000E-3"], ["-559.311E-3", "-13.873E+0", "-565.491E-3", "-14.023E+0", "-19.448E+0", "-20.307E+0", "894.438E+0", "-500.000E-3"], ["-516.586E-3", "-13.635E+0", "-508.804E-3", "-13.446E+0", "-19.491E+0", "-20.383E+0", "854.372E+0", "-450.000E-3"], ["-457.382E-3", "-12.192E+0", "-454.559E-3", "-12.311E+0", "-19.514E+0", "-20.451E+0", "804.276E+0", "-400.000E-3"], ["-404.587E-3", "-11.618E+0", "-400.162E-3", "-11.603E+0", "-19.533E+0", "-20.501E+0", "773.566E+0", "-350.000E-3"], ["-355.682E-3", "-10.532E+0", "-355.225E-3", "-10.071E+0", "-19.546E+0", "-20.543E+0", "744.690E+0", "-300.000E-3"], ["-309.219E-3", "-9.567E+0", "-303.802E-3", "-10.074E+0", "-19.563E+0", "-20.605E+0", "705.578E+0", "-250.000E-3"], ["-252.686E-3", "-8.945E+0", "-252.609E-3", "-8.673E+0", "-19.601E+0", "-20.680E+0", "674.590E+0", "-200.000E-3"], ["-201.111E-3", "-7.727E+0", "-205.078E-3", "-7.590E+0", "-19.650E+0", "-20.780E+0", "636.383E+0", "-150.000E-3"], ["-153.809E-3", "-5.951E+0", "-158.005E-3", "-6.284E+0", "-19.729E+0", "-20.910E+0", "600.845E+0", "-100.000E-3"], ["-96.970E-3", "-4.373E+0", "-107.956E-3", "-4.797E+0", "-19.794E+0", "-21.016E+0", "574.575E+0", "-50.000E-3"], ["-43.640E-3", "-2.356E+0", "-36.545E-3", "-2.161E+0", "-19.832E+0", "-21.101E+0", "546.658E+0", "-4.066E-15"], ["19.760E-3", "-424.194E-3", "4.272E-3", "-170.898E-3", "-19.910E+0", "-21.236E+0", "515.105E+0", "50.000E-3"], ["56.229E-3", "2.649E+0", "54.474E-3", "2.695E+0", "-19.812E+0", "-21.098E+0", "536.785E+0", "100.000E-3"], ["106.125E-3", "4.666E+0", "123.291E-3", "4.520E+0", "-19.773E+0", "-21.060E+0", "536.264E+0", "150.000E-3"], ["154.114E-3", "6.256E+0", "158.386E-3", "6.668E+0", "-19.684E+0", "-20.963E+0", "540.819E+0", "200.000E-3"], ["199.280E-3", "7.840E+0", "201.569E-3", "7.468E+0", "-19.590E+0", "-20.863E+0", "544.456E+0", "250.000E-3"], ["245.590E-3", "8.932E+0", "249.405E-3", "8.960E+0", "-19.488E+0", "-20.757E+0", "546.465E+0", "300.000E-3"], ["295.258E-3", "9.595E+0", "296.326E-3", "10.144E+0", "-19.407E+0", "-20.680E+0", "544.239E+0", "350.000E-3"], ["349.350E-3", "11.029E+0", "351.105E-3", "10.928E+0", "-19.336E+0", "-20.620E+0", "538.110E+0", "400.000E-3"], ["403.442E-3", "11.746E+0", "400.314E-3", "11.606E+0", "-19.273E+0", "-20.574E+0", "528.540E+0", "450.000E-3"], ["446.777E-3", "12.802E+0", "445.328E-3", "12.567E+0", "-19.219E+0", "-20.531E+0", "522.576E+0", "500.000E-3"], ["497.589E-3", "13.077E+0", "495.224E-3", "13.425E+0", "-19.160E+0", "-20.485E+0", "515.927E+0", "550.000E-3"], ["545.731E-3", "14.075E+0", "544.205E-3", "14.014E+0", "-19.080E+0", "-20.430E+0", "503.416E+0", "600.000E-3"], ["593.491E-3", "14.951E+0", "573.807E-3", "14.926E+0", "-19.004E+0", "-20.352E+0", "504.038E+0", "650.000E-3"], ["644.302E-3", "15.656E+0", "652.466E-3", "15.085E+0", "-18.901E+0", "-20.265E+0", "496.035E+0", "700.000E-3"], ["699.844E-3", "16.412E+0", "693.130E-3", "16.574E+0", "-18.810E+0", "-20.195E+0", "485.520E+0", "750.000E-3"], ["739.822E-3", "17.044E+0", "747.986E-3", "16.858E+0", "-18.770E+0", "-20.174E+0", "476.807E+0", "800.000E-3"], ["797.119E-3", "17.181E+0", "796.890E-3", "17.456E+0", "-18.869E+0", "-20.315E+0", "457.431E+0", "850.000E-3"], ["850.372E-3", "18.149E+0", "840.073E-3", "18.036E+0", "-19.174E+0", "-20.666E+0", "437.987E+0", "900.000E-3"], ["890.884E-3", "19.199E+0", "890.503E-3", "19.342E+0", "-19.551E+0", "-21.109E+0", "412.046E+0", "950.000E-3"], ["945.358E-3", "21.292E+0", "936.966E-3", "21.060E+0", "-19.788E+0", "-21.344E+0", "412.568E+0", "1.000E+0"], ["989.532E-3", "24.512E+0", "991.974E-3", "24.652E+0", "-19.840E+0", "-21.429E+0", "400.686E+0", "1.050E+0"], ["1.041E+0", "28.998E+0", "1.039E+0", "29.016E+0", "-19.828E+0", "-21.425E+0", "397.458E+0", "1.100E+0"], ["1.091E+0", "33.380E+0", "1.095E+0", "32.864E+0", "-19.765E+0", "-21.431E+0", "373.807E+0", "1.150E+0"], ["1.142E+0", "37.363E+0", "1.146E+0", "36.755E+0", "-19.566E+0", "-21.406E+0", "321.819E+0", "1.200E+0"], ["1.178E+0", "39.682E+0", "1.187E+0", "39.258E+0", "-19.194E+0", "-21.241E+0", "271.895E+0", "1.250E+0"], ["1.236E+0", "41.003E+0", "1.239E+0", "40.692E+0", "-18.648E+0", "-20.930E+0", "225.826E+0", "1.300E+0"], ["1.291E+0", "41.791E+0", "1.287E+0", "41.760E+0", "-18.108E+0", "-20.525E+0", "203.774E+0", "1.350E+0"], ["1.340E+0", "42.896E+0", "1.341E+0", "42.557E+0", "-17.651E+0", "-20.145E+0", "192.364E+0", "1.400E+0"], ["1.387E+0", "44.077E+0", "1.390E+0", "43.390E+0", "-17.325E+0", "-19.847E+0", "188.158E+0", "1.450E+0"], ["1.455E+0", "44.028E+0", "1.438E+0", "43.607E+0", "-17.083E+0", "-19.644E+0", "182.710E+0", "1.500E+0"], ["1.494E+0", "44.110E+0", "1.496E+0", "44.211E+0", "-16.947E+0", "-19.525E+0", "180.484E+0", "1.550E+0"], ["1.549E+0", "45.062E+0", "1.537E+0", "45.053E+0", "-16.858E+0", "-19.452E+0", "178.239E+0", "1.600E+0"], ["1.601E+0", "45.724E+0", "1.597E+0", "45.175E+0", "-16.787E+0", "-19.406E+0", "174.975E+0", "1.650E+0"], ["1.643E+0", "46.613E+0", "1.646E+0", "45.679E+0", "-16.696E+0", "-19.342E+0", "171.488E+0", "1.700E+0"], ["1.697E+0", "46.085E+0", "1.691E+0", "45.761E+0", "-16.480E+0", "-19.111E+0", "173.444E+0", "1.750E+0"], ["1.738E+0", "46.381E+0", "1.740E+0", "46.494E+0", "-16.314E+0", "-18.687E+0", "210.713E+0", "1.800E+0"], ["1.787E+0", "46.957E+0", "1.786E+0", "46.164E+0", "-16.829E+0", "-19.267E+0", "200.475E+0", "1.850E+0"], ["1.841E+0", "47.687E+0", "1.836E+0", "47.552E+0", "-16.797E+0", "-19.219E+0", "202.934E+0", "1.900E+0"], ["1.896E+0", "47.678E+0", "1.889E+0", "48.123E+0", "-16.370E+0", "-18.795E+0", "202.560E+0", "1.950E+0"], ["1.943E+0", "48.849E+0", "1.939E+0", "48.254E+0", "-16.613E+0", "-19.271E+0", "169.919E+0", "2.000E+0"], ["1.987E+0", "49.103E+0", "1.988E+0", "48.993E+0", "-16.848E+0", "-19.511E+0", "169.283E+0", "2.050E+0"], ["2.040E+0", "49.640E+0", "2.053E+0", "49.222E+0", "-17.000E+0", "-19.645E+0", "171.505E+0", "2.100E+0"], ["2.092E+0", "50.201E+0", "2.090E+0", "49.765E+0", "-17.181E+0", "-19.807E+0", "174.060E+0", "2.150E+0"], ["2.144E+0", "50.583E+0", "2.141E+0", "50.494E+0", "-17.410E+0", "-20.004E+0", "178.325E+0", "2.200E+0"], ["2.189E+0", "51.788E+0", "2.189E+0", "51.523E+0", "-17.775E+0", "-20.300E+0", "187.701E+0", "2.250E+0"], ["2.237E+0", "52.512E+0", "2.239E+0", "51.724E+0", "-18.280E+0", "-20.693E+0", "204.427E+0", "2.300E+0"], ["2.293E+0", "54.300E+0", "2.306E+0", "53.561E+0", "-18.990E+0", "-21.162E+0", "246.057E+0", "2.350E+0"], ["2.344E+0", "56.546E+0", "2.342E+0", "56.546E+0", "-19.505E+0", "-21.408E+0", "305.499E+0", "2.400E+0"], ["2.388E+0", "62.613E+0", "2.384E+0", "62.000E+0", "-19.812E+0", "-21.462E+0", "379.194E+0", "2.450E+0"], ["2.428E+0", "76.163E+0", "2.426E+0", "75.449E+0", "-19.947E+0", "-21.446E+0", "435.331E+0", "2.500E+0"], ["2.476E+0", "107.446E+0", "2.472E+0", "107.626E+0", "-20.004E+0", "-21.425E+0", "468.802E+0", "2.550E+0"], ["2.512E+0", "153.696E+0", "2.516E+0", "154.590E+0", "-20.018E+0", "-21.423E+0", "476.300E+0", "2.600E+0"], ["2.563E+0", "207.529E+0", "2.552E+0", "206.989E+0", "-20.018E+0", "-21.423E+0", "476.685E+0", "2.650E+0"], ["2.624E+0", "233.282E+0", "2.632E+0", "233.401E+0", "-19.991E+0", "-21.381E+0", "483.200E+0", "2.700E+0"], ["2.687E+0", "242.419E+0", "2.688E+0", "242.673E+0", "-19.856E+0", "-21.238E+0", "487.333E+0", "2.750E+0"], ["2.739E+0", "246.121E+0", "2.735E+0", "246.765E+0", "-19.660E+0", "-21.000E+0", "508.248E+0", "2.800E+0"], ["2.790E+0", "249.734E+0", "2.805E+0", "249.255E+0", "-19.575E+0", "-20.900E+0", "515.606E+0", "2.850E+0"], ["2.835E+0", "253.070E+0", "2.836E+0", "252.512E+0", "-19.587E+0", "-20.912E+0", "515.546E+0", "2.900E+0"], ["2.876E+0", "256.454E+0", "2.898E+0", "256.696E+0", "-19.627E+0", "-20.946E+0", "518.967E+0", "2.950E+0"], ["2.930E+0", "260.153E+0", "2.940E+0", "260.052E+0", "-19.663E+0", "-20.992E+0", "513.630E+0", "3.000E+0"], ["2.998E+0", "264.050E+0", "2.993E+0", "263.867E+0", "-19.677E+0", "-21.021E+0", "505.770E+0", "3.050E+0"], ["3.042E+0", "268.317E+0", "3.046E+0", "267.770E+0", "-19.693E+0", "-21.033E+0", "508.205E+0", "3.100E+0"], ["3.102E+0", "273.386E+0", "3.104E+0", "272.488E+0", "-19.707E+0", "-21.042E+0", "510.451E+0", "3.150E+0"], ["3.140E+0", "277.008E+0", "3.146E+0", "276.770E+0", "-19.721E+0", "-21.034E+0", "522.488E+0", "3.200E+0"], ["3.199E+0", "280.923E+0", "3.192E+0", "280.750E+0", "-19.737E+0", "-21.048E+0", "522.780E+0", "3.250E+0"], ["3.246E+0", "285.114E+0", "3.246E+0", "285.309E+0", "-19.728E+0", "-21.052E+0", "516.688E+0", "3.300E+0"], ["3.296E+0", "289.407E+0", "3.294E+0", "289.282E+0", "-19.734E+0", "-21.037E+0", "527.844E+0", "3.350E+0"], ["3.353E+0", "293.417E+0", "3.341E+0", "293.414E+0", "-19.743E+0", "-21.046E+0", "527.643E+0", "3.400E+0"], ["3.382E+0", "297.748E+0", "3.386E+0", "297.763E+0", "-19.735E+0", "-21.030E+0", "531.782E+0", "3.450E+0"], ["3.440E+0", "302.432E+0", "3.439E+0", "302.261E+0", "-19.740E+0", "-21.037E+0", "531.314E+0", "3.500E+0"]]
  in  "Calc_IFout":T29={"Th"=297.0, "Tc"=83.26, "BW (MHz)"=40.0, "NS_output_data"=path "C:/data/cartridge/SN80/CCA80-06/140205_DSB_IFBOX2/YIG_799.00_120_140205_CCA80-06_IFBOX2aNS.csv", "Rx_output_data"=path "C:/data/cartridge/SN80/CCA80-06/140205_DSB_IFBOX2/YIG_938.00_120_140205_CCA80-06_IFBOX2m.csv", "NS_ENR"=path "C:/Labview_ALMA/MIX10(win8.1)/140205_IFBOX_TY/NS_ENR_44421726.csv", "SAVE"=TRUE, "IFB_NS_AMP(filename)"="NS_amp.prn", "IFB_INPUT_CBL(filename) "="P0_inputcable.prn"}
  in  "CLNA_SET dummy":T4 {"SET POL0 LNA1 STAGE3 DRAIN C" min=0 max=20 step=0.01 format="%.2f"; "SET POL0 LNA1 STAGE3 DRAIN V" min=0 max=3 step=0.01 format="%.2f"; "SET POL0 LNA1 STAGE2 DRAIN C" min=0 max=20 step=0.01 format="%.2f"; "SET POL0 LNA1 STAGE2 DRAIN V" min=0 max=3 step=0.01 format="%.2f"; "SET POL0 LNA1 STAGE1 DRAIN C" min=0 max=20 step=0.01 format="%.2f"; "SET POL0 LNA1 STAGE1 DRAIN V" min=0 max=3 step=0.01 format="%.2f"; "CLNA State" items=["Disabled", "Enabled"]}
  in  "initial value":dbl[][](array[numeric])=[[1.0483870967741935, 0.0, 0.0], [2.1, 0.0, 0.0], [0.3629032258064516, 0.0, 12.91970802919708], [0.0, 0.0, 0.0], [0.0, 0.0, 0.0]]
  out "error out":errorcluster caption="Error output"
  in  "control IP":string
  out "Their Response":string caption="response"
  in  "send":string
  in  "Nitsuki_TDP_Command":bool
  in  "mk3d":T30={"Start(GHz)"=794.0, "Stop(GHz) "=938.0, "Step(GHz) "=8.0, "path"=path "L:/cartridge/assembly/SN03/03-13/110628_GUNNDSBFULL_P1", "first file name"="", "Acquisition column Z"=1, "Text line skip"=0, "Ring Z"=3, "Ring X"=0, "Acquisition column X"=0} {"Ring X" items=["IF(GHz)", "V(mV)"]; "Ring Z" items=["Trx(K)", "I (mA)", "P_PM (dBm)", "P_SP(dBm)", "SBR (dB)", "POUT(dBm/100MHz)", "P-P(dB)"]}
  in  "End of the equipment\nLOCAL":bool=TRUE
  out "IFpow(dBm)":dbl format="%.3f"
  out "Current (uA)":dbl=1.4178466983139515 format="%.2f"
  out "Volt(mV)":dbl=0.9882354736328125 format="%.3f"
  in  "SIScontrol":u16(ring) items=["CLOSE LOOP", "OPEN LOOP", "Not Control"]
  in  "STOP program":bool=TRUE
  in  "SISSetVolt":dbl(slide) min=0.0 max=20.0 scale=0.0..5.0
  # "https://ssl.pstatic.net/static/maps2/blank.gif"
  # "LO freq. [GHz]"
  # "YTO LOW\n/High Freq."
  # "ZERO Intgrtr"
  # "Node Address"
  # "Serial Number"
  # "Vd [V]"
  # "Id [mA]"
  # "Stage 1"
  # "Stage 2"
  # "Stage 3"
  # "CLNA State."
  # "Vd [V]"
  # "Id [mA]"
  # "Vg [V]"
  # "Stage 1"
  # "Stage 2"
  # "Stage 3"
  # "Magnet current"
  # "Magnet current"
  # "SIS Bias range"
  # "-3V/5V Supply"
  # "Vd [V]"
  # "Id [mA]"
  # "Vg [V]"
  # "PA A"
  # "PA B"
  # "NS_ENR same directory as"
  # "Vd [V]"
  # "Id [mA]"
  # "Stage 1"
  # "Stage 2"
  # "Stage 3"
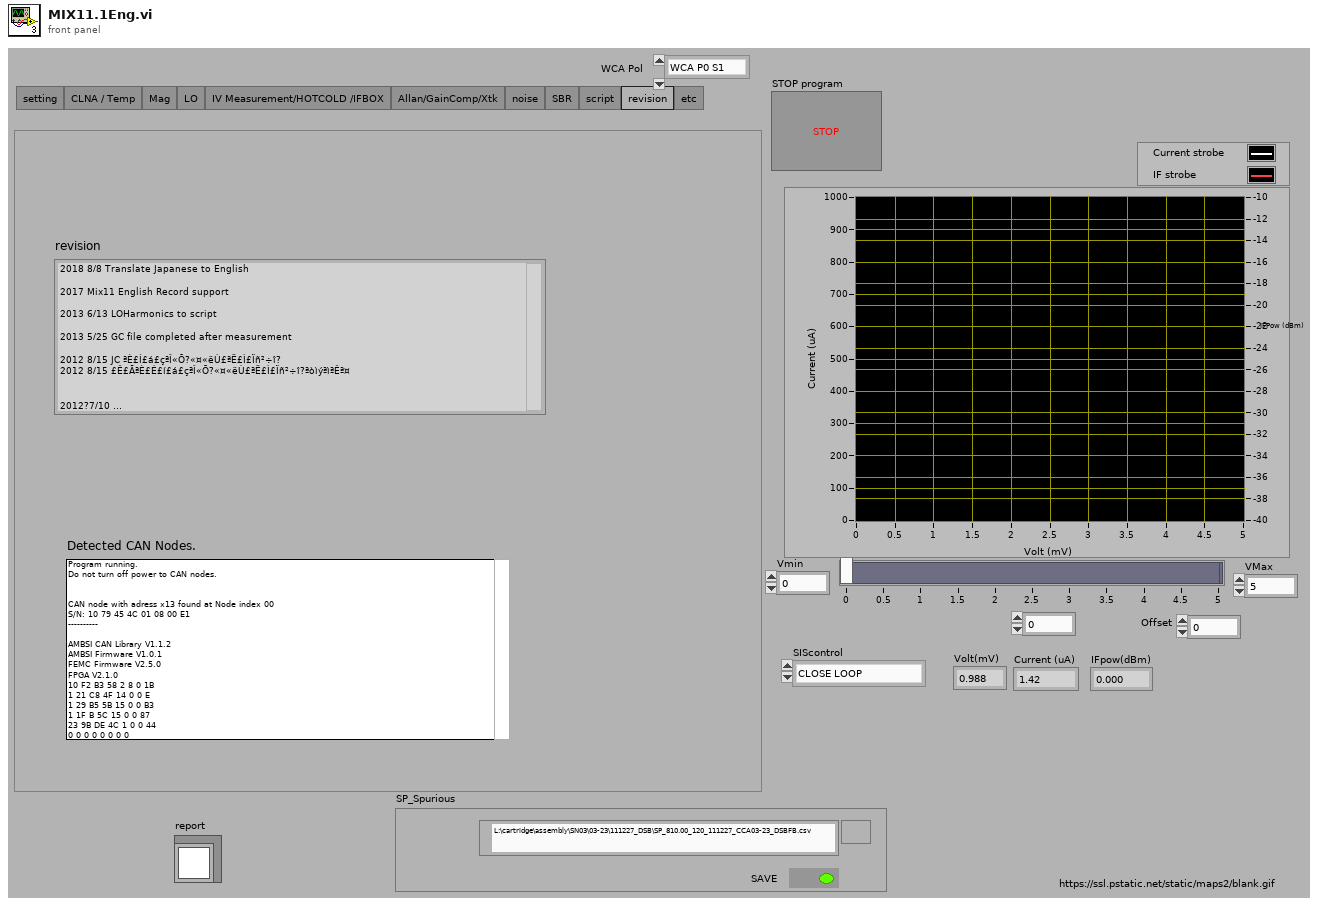
[diagram p1: front panel]
types:
  T1 = enum32{"setting", "CLNA / Temp", "Mag", "LO", "IV Measurement/HOTCOLD /IFBOX", "Allan/GainComp/Xtk", "noise", "SBR", "script", "revision", "etc"}
  T2 = cluster{"Node address":u16, "CAN Interface":string, "Cartridge band":u32, "Slave Node in":cluster{"Address":i16, "Serial Number":i8[]}, "ObjHandle out":u32, "POL":u32, "sb":u32, "GPIB_SM (SIS S,V)":string, "GPIB_DMM (SIS I)":string, "GPIB_SM (MAG I) ":string, "GPIB_SG(LO)":string, "GPIB_PW (PAMP) ":string, "GPIB_TMP1(8ch)":string, "GPIB_TMP2(2ch)":string, "WCA_avg":i32, "Rsen":dbl, "BiasModule":u16, "LOModule ":u16, "WCA_LO_FREQ_SET":cluster{"YTO Low freq. [GHz]":sgl, "YTO High freq. [GHz]":sgl, "Kvco":u16, "Lock Pol.":u16, "SET LO FREQ":sgl, "Multiplier":sgl, "YTO (HEX)":u16, "YTO ( FREQ)":sgl, "NULL PLL INTEGRATOR":bool}, "Res for":u16}
  T3 = cluster{"GPIB_ATT":string, "6501Dev#":i16, "GPIB_SpecA":string, "GPIB_PM":string, "GPIB_DSA":string, "GPIB_DMM (TPD)":string, "MPI COM":refnum<visa-resource-name>, "motor setting":cluster{"Axis":i16, "ID":i16, "HIspeed":dbl, "LOspeed":dbl, "ACCEL(ms)":dbl, "Sratio":dbl, "free run\n":bool, "motor":string}[], "DATA path":path, "mixer param file ":path, "comment":string, "Carteidge SN":string, "Th":dbl, "Tc":dbl, "Set_SIS_volt":dbl, "Offset":dbl, "control":u16, "FreqLO":dbl, "Set_Mag_Cur":dbl, "MPI offset(mm)":dbl, "HOT/COLD":u16}
  T4 = cluster{"CLNA State":u8, "SET POL0 LNA1 STAGE1 DRAIN V":sgl, "SET POL0 LNA1 STAGE1 DRAIN C":sgl, "SET POL0 LNA1 STAGE2 DRAIN V":sgl, "SET POL0 LNA1 STAGE2 DRAIN C":sgl, "SET POL0 LNA1 STAGE3 DRAIN V":sgl, "SET POL0 LNA1 STAGE3 DRAIN C":sgl}
  T5 = cluster{"Pol0 LNA1 S1 Drain V [V]":sgl, "Pol0 LNA1 S1 Drain C [mA]":sgl, "Pol0 LNA1 S1 Gate V [V]":sgl, "Pol0 LNA1 S2 Drain V [V]":sgl, "Pol0 LNA1 S2 Drain C [mA]":sgl, "Pol0 LNA1 S2 Gate V [V]":sgl, "Pol0 LNA1 S3 Drain V [V]":sgl, "Pol0 LNA1 S3 Drain C [mA]":sgl, "Pol0 LNA1 S3 Gate V [V]":sgl, "Pol0 LNA1 State":enum16{"Disabled", "Enabled"}}
  T6 = cluster{"VDmin":dbl, "VDmax":dbl, "VDstep":dbl, "IDmin":dbl, "IDmax":dbl, "IDstep":dbl, "wait (mS)":dbl, "P.M.aveg":i32, "HOT/COLD ":u16, "SIS hotV ":dbl, "SIS coldV":dbl, "file_name":string, "frq(GHz)":dbl}
  T7 = cluster{"Start(mA)":dbl, "Time(ms)":dbl, "step":dbl}
  T8 = cluster{"start(mA)":dbl, "stop(mA)":dbl, "step(mA)":dbl, "file_name":string, "file path":path, "save?":bool, "SIS Bias range Vsis":cluster{"start":dbl, "stop":dbl, "step":dbl}}
  T9 = cluster{"start(mA)":dbl, "stop(mA)":dbl, "step(mA)":dbl, "start(mV)":dbl, "stop(mV)":dbl, "step(mV)":dbl, "file_name":string, "path":path, "save?":bool}
  T10 = cluster{"ON start time (ms)":dbl, "ON duration time (ms)":dbl, "Measurement end time":dbl, "SIS Volt (mV)":dbl, "GPIB_PW (SISHeater) ":string, "SAVE":bool, "file_name":string, "path":path}
  T11 = cluster{"LO FRQ(GHz)":dbl, "LO multi ":dbl, "LocK?":bool, "LO REF multi":dbl, "wait (ms)":dbl, "SG Pow Min (dBm)":dbl, "SG Pow Max (dBm)":dbl, "SG Pow Step (dBm)":dbl, "SGPow OPT? ":bool, "SG set frq":dbl, "SG set pow":dbl}
  T12 = cluster{"PA_A_DRAIN_V":sgl, "PA_A_DRAIN_C":sgl, "PA_A_GATE_V":sgl, "PA_B_DRAIN_V":sgl, "PA_B_DRAIN_C":sgl, "PA_B_GATE_V":sgl, "PA_3V_SUPPLY_V":sgl, "PA_5V_MON":sgl}
  T13 = cluster{"PLL_ASSY_T":sgl, "PLL_REF_TOT_P":sgl, "PLL_IF_TOT_P":sgl, "PLL_CORR_V":sgl, "PLL_LOCK_V":sgl, "PLL_5V_SUPPLY_V":sgl, "Temp_TF":bool, "PLL Ref Pwr_TF":bool, "IF Pwr_TF":bool, "PLL Corr_TF":bool, "PLL Lock V_TF":bool, "PLL Nominal_TF":bool}
  T14 = cluster{"Range Array":cluster{"Start":dbl, "Stop":dbl, "Step":dbl, "By":string}[], "Optimize":u16, "file_name":string, "Save?":bool, "measure":u16, "current(uA)":dbl, "wait(ms)":i32, "IFfrq(GHz)":dbl, "aveg":i32, "SISparam option":u16}
  T15 = cluster{"scales":dbl, "start (GHz)":dbl, "stop (GHz)":dbl, "step (GHz) ":dbl, "Wait(ms)":dbl, "file_name":string, "path":path, "measure":u16, "WCA Pol":u16}
  T16 = cluster{" Output":u16, "YIG Fc(GHz)":dbl, " Filter":u16, "Input":u16}
  T17 = cluster{"start(mV)":dbl, "stop(mV)":dbl, "step(mV)":dbl, "file_name":string, "IF OFF/ON":bool, "SAVE OFF/ON":bool, "frq(GHz)":dbl, "avg":i32, "number of Sweep  ":u16, "VminfromSS":dbl, "mode ":u16, "V@opt":u16}
  T18 = cluster{"save":bool, "file_name":string, "IF start":dbl, "IF stop":dbl, "IF step":dbl}
  T19 = cluster{"GPIB":string, "wait(s)":dbl, "measure(s) ":dbl, "save":bool, "time constant":u16, "file_name":string}
  T20 = cluster{"DMM Setting A":cluster{"interval":dbl, "sample number":i32, "Voltage Range":enum16{"100 mV", "1 V", "10 V", "100 V", "1000 V", "Auto", "Minimum", "Maximum"}, "Factor":dbl, "unit":u16, "Power supply freq. (Hz)":dbl}, "Path":path, "File name":string, "DMM":u16, "DSA_mes":cluster{"GPIB_DSA":string, "Startfrq(Hz)":dbl, "Stopfrq(Hz)":dbl, "Range(Vpk)":dbl, "average":i16}, " temperature?":bool, "time interval":dbl}
  T21 = cluster{"save":bool, "file_name":string, "LO start":dbl, "LO stop":dbl, "LO step":dbl, "IF":dbl, "8th 10th":bool}
  T22 = cluster{"total data num(1-3)":i16, "file_name":string, "SAVE OFF/ON":bool, "ATT1":dbl, "ATT2":dbl, "SNAdatafile ATT1":path, "SNAdatafile ATT2":path, "ATTcal":bool, "SP_set":cluster{"start(GHz)":dbl, "stop(GHz) ":dbl, "BW(MHz)":dbl, "VBW(Hz)":dbl, "ref(dBm)":dbl, "log(dB)":dbl, "AVEG":i16, "AVEG ON/OFF":bool, "Auto Align ON/OFF":bool, "GPIB":string, "point":i16}, "HOT/COLD":u16}
  T23 = cluster{"Start(GHz)":dbl, "Stop(GHz)":dbl, "Step(GHz) ":dbl, "wait (S)":dbl, "Hot/Cold Switch":u16, "file_name":string, "P.M.aveg":i32, "save":bool}
  T24 = cluster{"wait(ms)":i32, "Start":dbl, "Stop":dbl, "Step":dbl, "save":bool, "file_name":string}
  T25 = cluster{"file_name":string, "HOT/COLD AUTO":bool, "MPI SSB Set":bool, "Waiting time at AUTO(S)":dbl, "P/V         V/P":bool, "save":bool, "start(GHz)":dbl, "stop(GHz) ":dbl, "Step(GHz) ":dbl, "P.M.aveg":i32, "PM        SP":bool, "SP_set":cluster{"start(GHz)":dbl, "stop(GHz) ":dbl, "BW(MHz)":dbl, "VBW(Hz)":dbl, "ref(dBm)":dbl, "log(dB)":dbl, "AVEG":i16, "AVEG ON/OFF":bool, "Auto Align ON/OFF":bool, "GPIB":string, "point":i16}}
  T26 = cluster{"RF(GHz)":dbl, "mm_multi(4or6)":dbl, "SGPOUT(dBm)":dbl, "SGGPIB":string, "PAMP GPIB":string, "VD (V)":dbl, "VG (V)":dbl, "multi (V)":dbl}
  T27 = cluster{"run number":i32, "number of lines":i32, "option":string, "Lupu's numerical value":dbl, "Lupe Stop":dbl, "Lupe Step":dbl, "Line number":i32}[]
  T28 = enum32{"Page 1", "Page 2", "Page 3", "Nitsuki_TPD", "Page 4"}
  T29 = cluster{"Th":dbl, "Tc":dbl, "BW (MHz)":dbl, "NS_output_data":path, "Rx_output_data":path, "NS_ENR":path, "SAVE":bool, "IFB_NS_AMP(filename)":string, "IFB_INPUT_CBL(filename) ":string}
  T30 = cluster{"Start(GHz)":dbl, "Stop(GHz) ":dbl, "Step(GHz) ":dbl, "path":path, "first file name":string, "Acquisition column Z":i32, "Text line skip":i32, "Ring Z":u16, "Ring X":u16, "Acquisition column X":i32}
  T31 = enum16{"Standard Report", "HTML", "Word", "Excel"}
  T32 = cluster{"position (Excel)":cluster{"row":i32, "column":i32}, "name (Excel)":string, "bookmark (Word)":string}
  T33 = cluster{"Axis":i16, "ID":i16, "HIspeed":dbl, "LOspeed":dbl, "ACCEL(ms)":dbl, "Sratio":dbl, "free run\n":bool, "motor":string}[]
  T34 = cluster{"Axis":i16, "ID":i16, "HIspeed":dbl, "LOspeed":dbl, "ACCEL(ms)":dbl, "Sratio":dbl, "free run\n":bool, "motor":string}
  T35 = cluster{"Node address":u16, "CAN Interface":string, "Cartridge band":u32, "Slave Node in":cluster{"Address":i16, "Serial Number":i8[]}, "ObjHandle out":u32, "POL":u32, "sb":u32, "GPIB_SM (SIS S,V)":string, "GPIB_DMM (SIS I)":string, "GPIB_SM (MAG I) ":string, "GPIB_SG(LO)":string, "GPIB_PW (PAMP) ":string, "GPIB_TMP1(8ch)":string, "GPIB_TMP2(2ch)  ":string, "WCA_avg":i32, "Rsen":dbl, "BiasModule":u16, "LOModule ":u16, "WCA_LO_FREQ_SET":cluster{"YTO Low freq. [GHz]":sgl, "YTO High freq. [GHz]":sgl, "Kvco":u16, "Lock Pol.":u16, "SET LO FREQ":sgl, "Multiplier":sgl, "YTO (HEX)":u16, "YTO ( FREQ)":sgl, "NULL PLL INTEGRATOR":bool}, "Res for":u16}
  T36 = cluster{"GPIB_ATT":string, "6501Dev#":i16, "GPIB_SP":string, "GPIB_PM":string, "GPIB_DSA":string, "GPIB_DMM (TPD)":string, "GPIB_MPI":string, "mortorÝè":cluster{"Axis":i16, "ID":i16, "HIspeed":dbl, "LOspeed":dbl, "ACCEL(ms)":dbl, "Sratio":dbl, "フリーラン\n":bool, "•¶Žš—ñ":string}[], "DATAパス":path, "DBパス ":path, "comment":string, "ColdCarts":string, "Th":dbl, "Tc":dbl, "Set_SIS_volt":dbl, "Offset":dbl, "control":u16, "FreqLO":dbl, "Set_Mag_Cur":dbl, "MPI offset(mm)":dbl, "HOT/COLD":u16}
  T37 = cluster{"run number":i32, "number of lines":i32, "option":string, "Lupu's numerical value":dbl, "Lupe Stop":dbl, "Lupe Step":dbl, "Line number":i32}
  T38 = cluster{"Node address":u16, "CAN Interface":string, "Cartridge band":u32, "Slave Node in":cluster{"Address":i16, "Serial Number":i8[]}, "ObjHandle out":u32, "POL":u32, "sb":u32, "GPIB_SM (SIS S,V)":string, "GPIB_DMM (SIS I)":string, "GPIB_SM (MAG I) ":string, "GPIB_SG(LO)":string, "GPIB_PW (PAMP) ":string, "GPIB_TMP1(8ch)":string, "GPIB_TMP2(2ch)  ":string, "WCA_avg":i32, "Rsen":dbl, "BiasModule":u16, "LOModule ":u16, "WCA_LO_FREQ_SET":cluster{"YTO Low freq. [GHz]":sgl, "YTO High freq. [GHz]":sgl, "Kvco":u16, "Lock Pol.":u16, "SET LO FREQ":sgl, "Multiplier":sgl, "YTO (HEX)":u16, "YTO coarse( FREQ)":sgl, "NULL PLL INTEGRATOR":bool}, "Res for":u16}
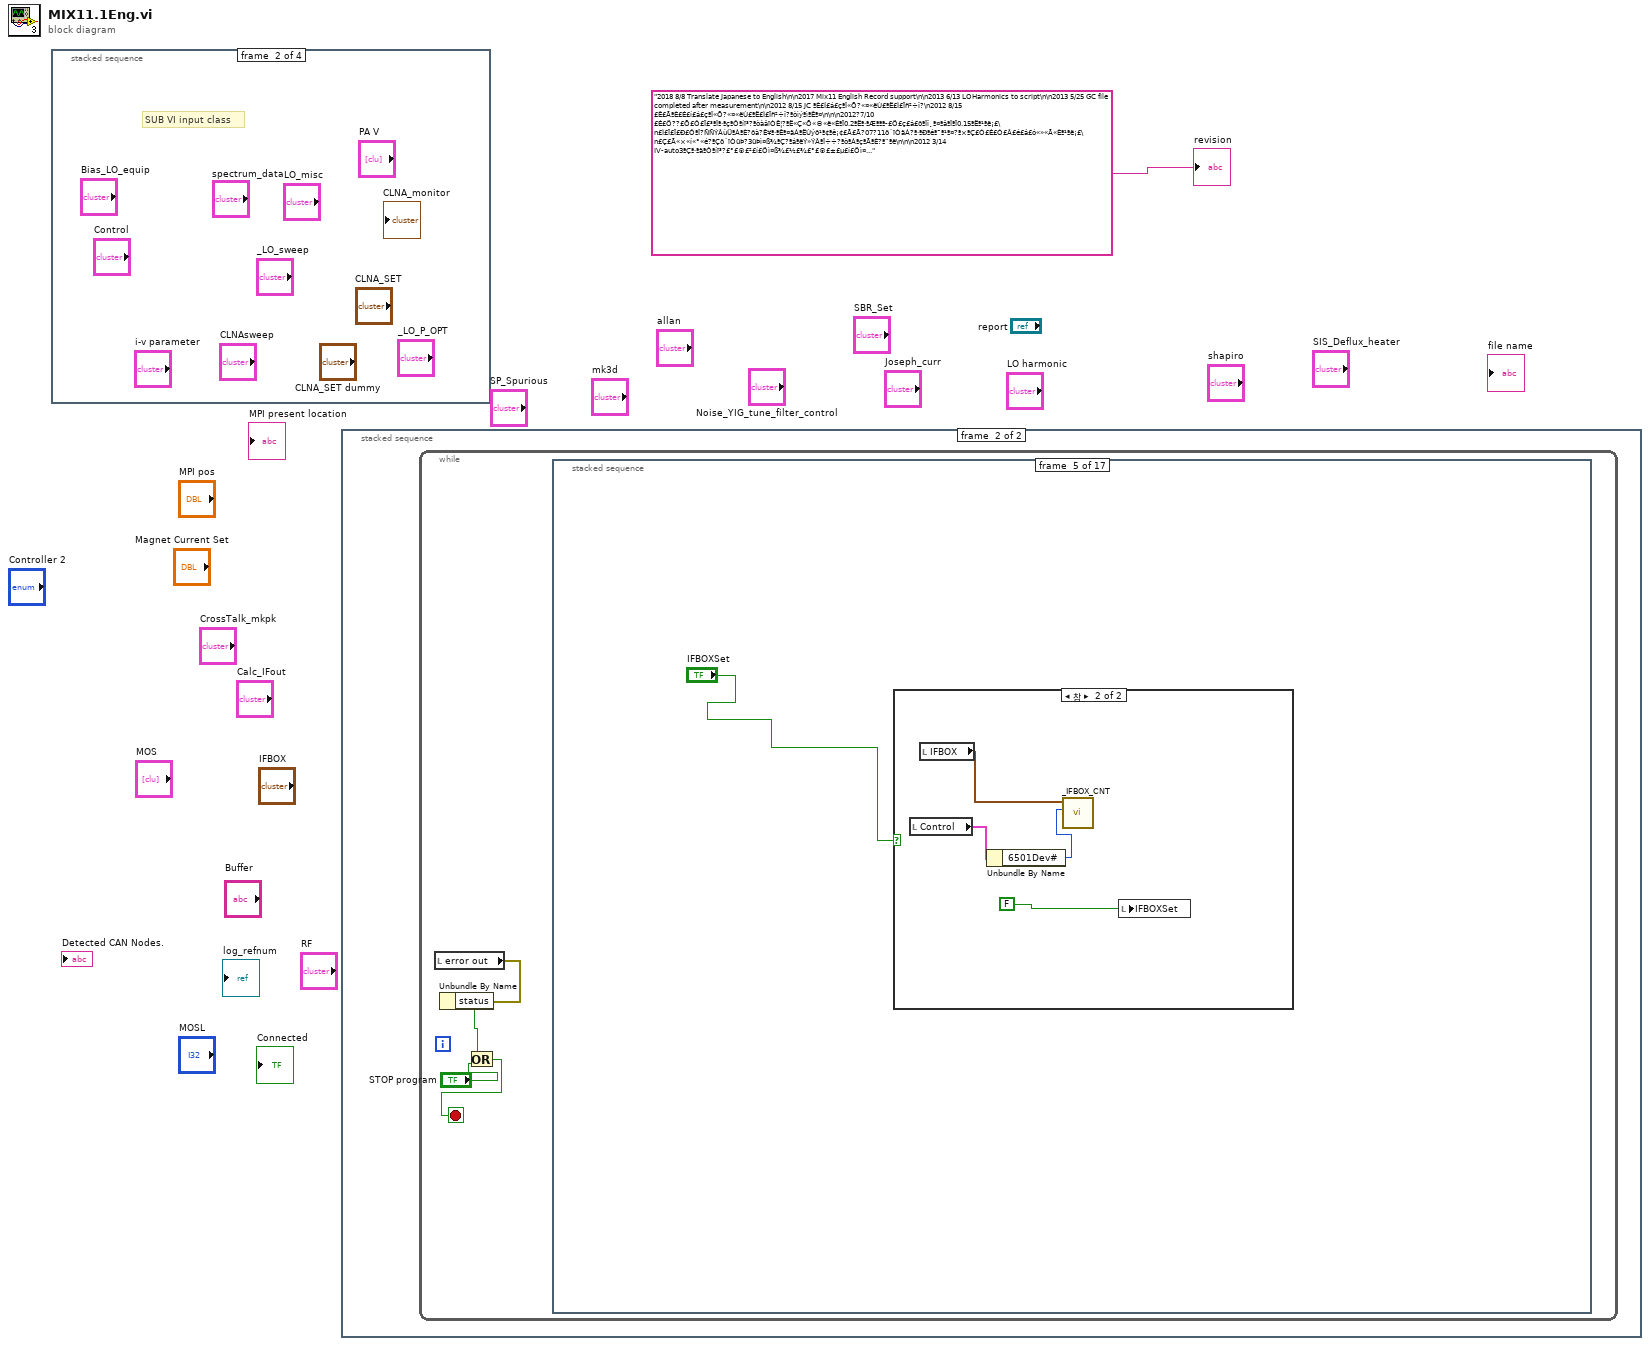
[diagram p0: block diagram]
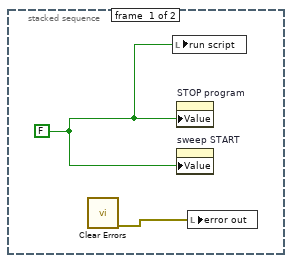
[diagram p2: hidden frame]
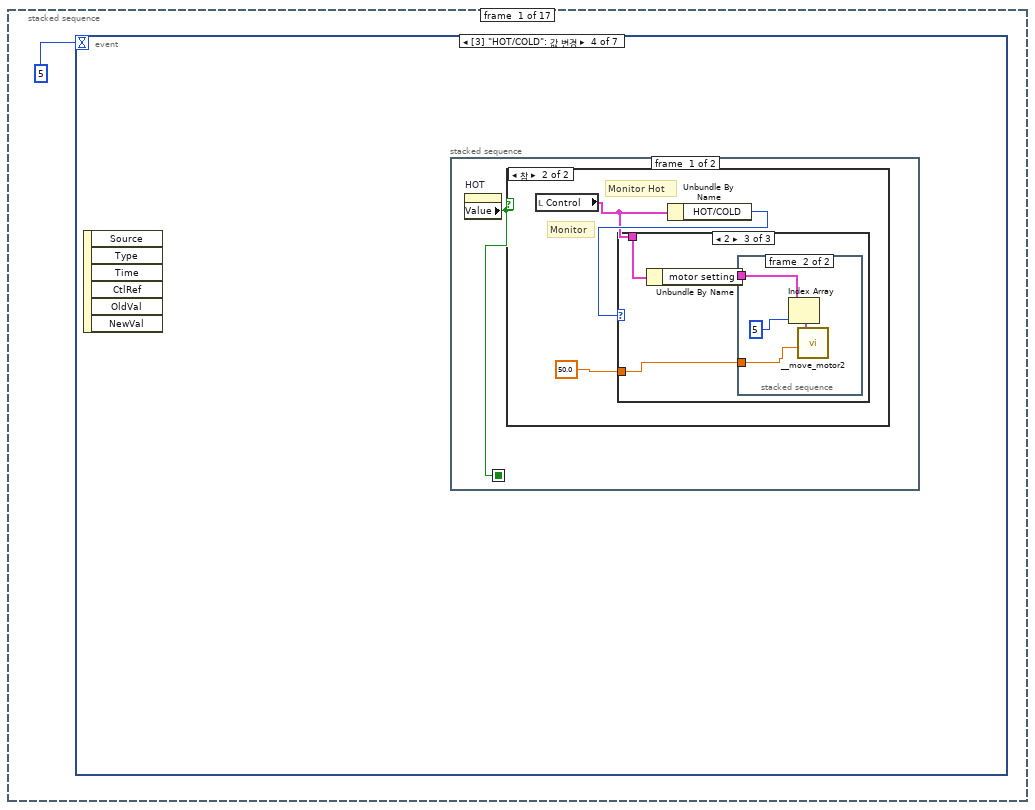
[diagram p3: hidden frame]
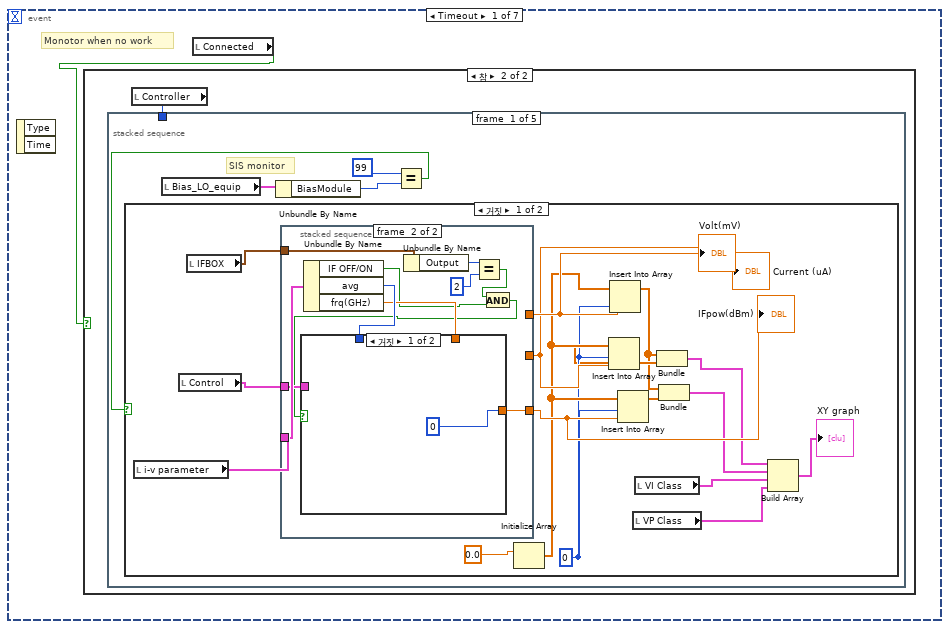
[diagram p4: hidden frame]
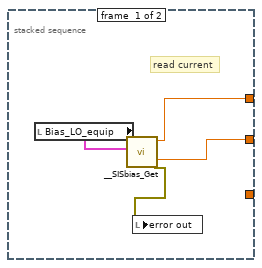
[diagram p6: hidden frame]
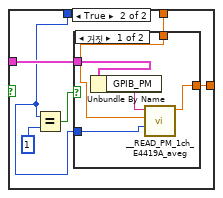
[diagram p7: hidden frame]
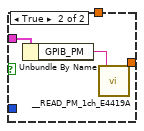
[diagram p8: hidden frame]
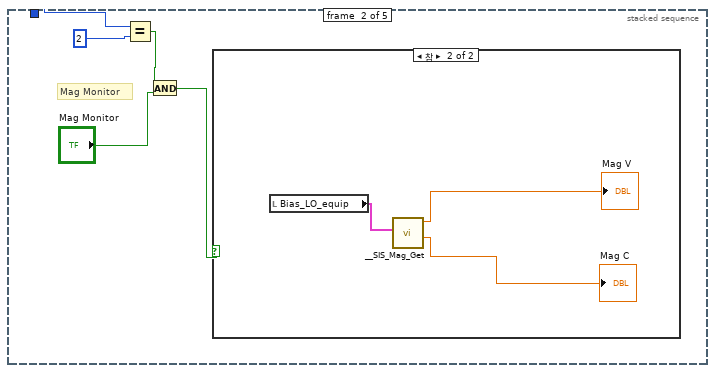
[diagram p10: hidden frame]
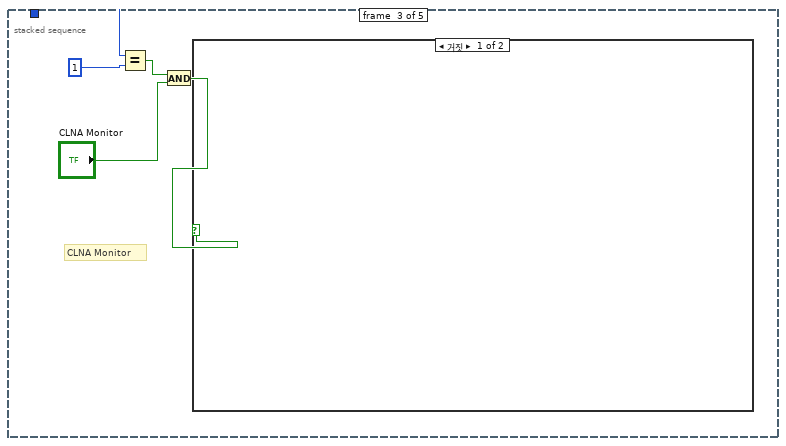
[diagram p12: hidden frame]
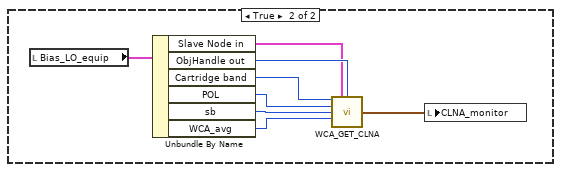
[diagram p13: hidden frame]
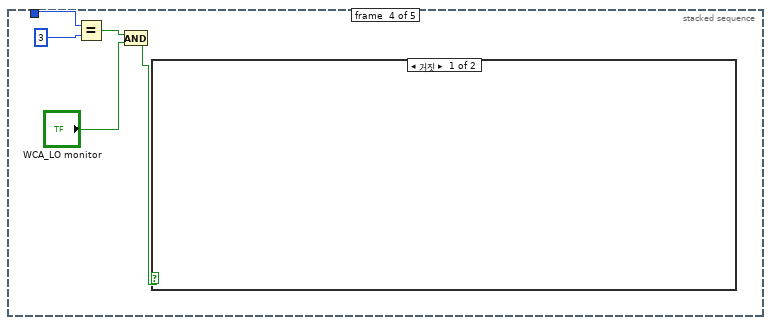
[diagram p14: hidden frame]
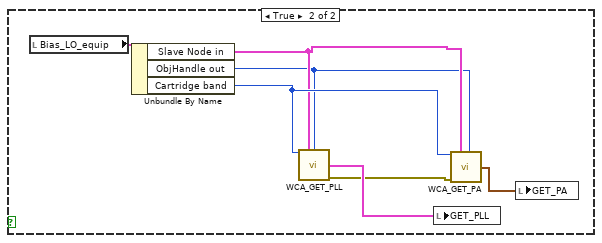
[diagram p15: hidden frame]
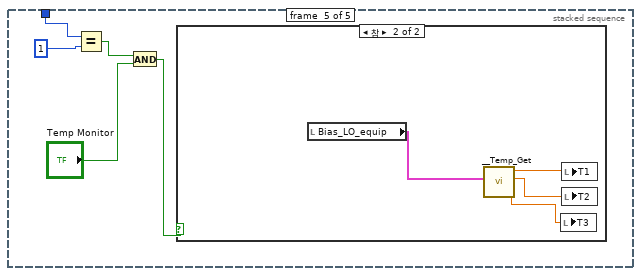
[diagram p16: hidden frame]
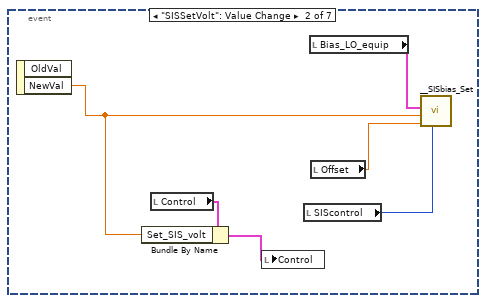
[diagram p18: hidden frame]
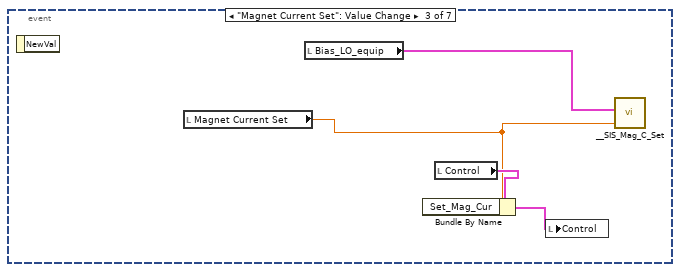
[diagram p19: hidden frame]
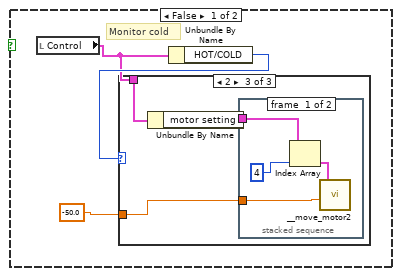
[diagram p20: hidden frame]
diagram:
  n1 = stacked-sequence {
    frame #0 {
    }
    frame #1 {
      # "SUB VI input class"
    }
    frame #2 {
      # "Monitor"
    }
    frame #3 {
      # "Script"
    }
  }
  n2 = stacked-sequence {
    frame #0 {
      w2 = FALSE
      n3 = call <vilib>:"Clear Errors.vi"() -> ("error out"=w3:errorcluster)  [unwired: 6 in, 1 out]
      n4 = local write "run script"(w2) -> ()
      n5 = property on="STOP program" class="Bool (엄격한)"("Value"=w2) -> ()  [unwired: 2 in, 2 out]
      n6 = property on="sweep START" class="Bool (엄격한)"("Value"=w2) -> ()  [unwired: 2 in, 2 out]
      n7 = local write "error out"(w3) -> ()
    }
    frame #1 {
      n8 = while {
        stop <- w4 stop-if-true
        n9 = local read "error out"() -> (w7:errorcluster)
        n10 = Unbundle By Name(w7) -> ("status"=w5:bool)
        n11 = Or(x=w5, y="STOP program") -> (x .or. y?=w4:bool)
        n12 = stacked-sequence {
          frame #0 {
            n13 = event shown="[3] \"HOT/COLD\": 값 변경" {
              selector: _ -> [_ _ _ _ _ _ _]
              dyn-events: _ -> [_ _ _ _ _ _ _]
              timeout: 5 -> [_ _ _ _ _ _ _]
              event Timeout {
                # "Monotor when no work"
                n14 = event-data() -> ()  [unwired: 1 in, 2 out]
                n15 = local read "Connected"() -> (w9:bool)
                n16 = case shown="참" w9 {
                  frame False {
                  }
                  frame True {
                    n17 = local read "Controller"() -> (w10:T1)
                    n18 = stacked-sequence {
                      tunnel: w10 -> [_ w65 w73 w86 w97]
                      frame #0 {
                        # "SIS monitor"
                        n19 = local read "Bias_LO_equip"() -> (w14:T2)
                        n20 = Unbundle By Name(w14) -> ("BiasModule"=w13:u16)
                        n21 = Equal?(x=99, y=w13) -> (x = y?=w11:bool)
                        n22 = case shown="거짓" w11 {
                          frame False {
                            w25 = 0
                            n23 = local read "i-v parameter"() -> (w28:T17)
                            n24 = local read "Control"() -> (w16:T3)
                            n25 = local read "IFBOX"() -> (w15:T16)
                            n26 = stacked-sequence {
                              tunnel: [w33 _] -> w30
                              tunnel: [_ w46] -> w29
                              tunnel: w28 -> [_ w43]
                              tunnel: [w34 _] -> w31
                              tunnel: w16 -> [_ w42]
                              tunnel: w15 -> [_ w41]
                              frame #0 {
                                # "read current"
                                n27 = local read "Bias_LO_equip"() -> (w35:T2)
                                n28 = call "__SISbias_Get.vi"("Bias_LO_equip"=w35) -> ("error out"=w32:errorcluster, "Get_I(uA)"=w33:dbl, "Get_V(mV)"=w34:dbl)  [unwired: 8 in]
                                n29 = local write "error out"(w32) -> ()
                              }
                              frame #1 {
                                n30 = Unbundle By Name(w43) -> ("IF OFF/ON"=w37:bool, "avg"=w45:i32, "frq(GHz)"=w44:dbl)
                                n31 = Unbundle By Name(w41) -> ("Output"=w40:u16)
                                n32 = Equal?(x=w40, y=2) -> (x = y?=w38:bool)
                                n33 = And(x=w38, y=w37) -> (x .and. y?=w36:bool)
                                n34 = case shown="거짓" w36 {
                                tunnel: [0 w53] -> w46
                                tunnel: w45 -> [_ w48]
                                tunnel: w44 -> [_ w50]
                                tunnel: w42 -> [_ w49]
                                frame False {
                                }
                                frame True {
                                n35 = Equal?(x=w48, y=1) -> (x = y?=w51:bool)
                                n36 = case shown="거짓" w51 {
                                tunnel: [w58 w61] -> w53
                                tunnel: w50 -> [w56 _]
                                tunnel: w48 -> [w55 _]
                                tunnel: w49 -> [w54 w60]
                                frame False {
                                n37 = Unbundle By Name(w54) -> ("GPIB_PM"=w57:string)
                                n38 = call "__READ_PM_1ch_E4419A_aveg.VI"("aveg"=w55, "frq(GHz)"=w56, "GPIB"=w57) -> ("chA"=w58:dbl)  [unwired: 4 in]
                                }
                                frame True {
                                n39 = Unbundle By Name(w60) -> ("GPIB_PM"=w59:string)
                                n40 = call "__READ_PM_1ch_E4419A.VI"("GPIB"=w59) -> ("chA"=w61:dbl)  [unwired: 6 in]
                                }
                                }
                                }
                                }
                              }
                            }
                            "Volt(mV)" <- w31
                            "Current (uA)" <- w30
                            "IFpow(dBm)" <- w29
                            n41 = Initialize Array(0.0) -> (w27:dbl[])  [unwired: 1 in]
                            n42 = Insert Into Array(array=w27, index=w25, new element=w30) -> (w24:dbl[])
                            n43 = Insert Into Array(array=w27, index=w25, new element=w31) -> (w23:dbl[])
                            n44 = Insert Into Array(array=w27, index=w25, new element=w29) -> (w22:dbl[])
                            n45 = local read "VP Class"() -> (w18:cluster{"”z—ñ":dbl[], "”z—ñ 2":dbl[]})
                            n46 = local read "VI Class"() -> (w19:cluster{"”z—ñ":dbl[], "”z—ñ 2":dbl[]})
                            n47 = Bundle(w23, w24) -> (w21:cluster{dbl[], dbl[]})  [unwired: 1 in]
                            n48 = Bundle(w23, w22) -> (w20:cluster{dbl[], dbl[]})  [unwired: 1 in]
                            n49 = Build Array(w21, w20, w19, w18) -> (→"XY graph":cluster{"”z—ñ":dbl[], "”z—ñ 2":dbl[]}[])
                          }
                          frame True {
                          }
                        }
                      }
                      frame #1 {
                        # "Mag Monitor"
                        n50 = Equal?(x=w65, y=2) -> (x = y?=w63:bool)
                        n51 = And(x=w63, y="Mag Monitor") -> (x .and. y?=w64:bool)
                        n52 = case shown="참" w64 {
                          frame False {
                          }
                          frame True {
                            n53 = local read "Bias_LO_equip"() -> (w69:T2)
                            n54 = call "__SIS_Mag_Get.vi"("Bias_LO_equip"=w69) -> ("Get_Mag_I"=→"Mag C":dbl, "Get_Mag_V"=→"Mag V":dbl)  [unwired: 9 in]
                          }
                        }
                      }
                      frame #2 {
                        # "CLNA Monitor"
                        n55 = Equal?(x=w73, y=1) -> (x = y?=w72:bool)
                        n56 = And(x=w72, y="CLNA Monitor") -> (x .and. y?=w70:bool)
                        n57 = case shown="거짓" w70 {
                          frame False {
                          }
                          frame True {
                            n58 = local read "Bias_LO_equip"() -> (w82:T2)
                            n59 = Unbundle By Name(w82) -> ("Slave Node in"=w77:cluster{"Address":i16, "Serial Number":i8[]}, "ObjHandle out"=w81:u32, "Cartridge band"=w80:u32, "POL"=w75:u32, "sb"=w79:u32, "WCA_avg"=w78:i32)
                            n60 = call "WCA_GET_CLNA.vi"("Cartridge Band"=w80, "Slave Node in"=w77, "ObjHandle in"=w81, "POL"=w75, "sb"=w79, "avg"=w78) -> ("CLNA_monitor"=w76:T5)  [unwired: 7 in, 2 out]
                            n61 = local write "CLNA_monitor"(w76) -> ()
                          }
                        }
                      }
                      frame #3 {
                        n62 = Equal?(x=w86, y=3) -> (x = y?=w85:bool)
                        n63 = And(x=w85, y="WCA_LO monitor") -> (x .and. y?=w83:bool)
                        n64 = case shown="거짓" w83 {
                          frame False {
                          }
                          frame True {
                            n65 = local read "Bias_LO_equip"() -> (w93:T2)
                            n66 = Unbundle By Name(w93) -> ("Slave Node in"=w90:cluster{"Address":i16, "Serial Number":i8[]}, "ObjHandle out"=w89:u32, "Cartridge band"=w91:u32)
                            n67 = call "WCA_GET_PLL.vi"("Cartridge Band"=w91, "Slave Node in"=w90, "ObjHandle in"=w89) -> ("GET_PLL"=w94:T13, "error out"=w92:errorcluster)  [unwired: 10 in, 1 out]
                            n68 = local write "GET_PLL"(w94) -> ()
                            n69 = call "WCA_GET_PA.vi"("Cartridge Band"=w91, "Slave Node in"=w90, "ObjHandle in"=w89, "error in (no error)"=w92) -> ("GET_PA"=w88:T12)  [unwired: 9 in, 2 out]
                            n70 = local write "GET_PA"(w88) -> ()
                          }
                        }
                      }
                      frame #4 {
                        n71 = Equal?(x=w97, y=1) -> (x = y?=w98:bool)
                        n72 = And(x=w98, y="Temp Monitor") -> (x .and. y?=w95:bool)
                        n73 = case shown="참" w95 {
                          frame False {
                          }
                          frame True {
                            n74 = local read "Bias_LO_equip"() -> (w103:T2)
                            n75 = call "__Temp_Get.vi"("Bias_LO_equip"=w103) -> ("MixTemp"=w100:dbl, "90/20K_temp"=w101:dbl, "4K_Temp"=w102:dbl)  [unwired: 8 in]
                            n76 = local write "T3"(w100) -> ()
                            n77 = local write "T1"(w102) -> ()
                            n78 = local write "T2"(w101) -> ()
                          }
                        }
                      }
                    }
                  }
                }
              }
              event "SISSetVolt": Value Change {
                n79 = event-data() -> ("NewVal"=w105:dbl)  [unwired: 1 in, 1 out]
                n80 = local read "Control"() -> (w106:T3)
                n81 = Bundle By Name(cluster=w106, "Set_SIS_volt"=w105) -> (w104:T3)
                n82 = local write "Control"(w104) -> ()
                n83 = local read "SIScontrol"() -> (w107:u16)
                n84 = local read "Bias_LO_equip"() -> (w109:T2)
                n85 = local read "Offset"() -> (w108:dbl)
                n86 = call "__SISbias_Set.vi"("SIS@Mode"=w107, "Offset"=w108, "Set_V"=w105, "Bias_LO_equip"=w109) -> ()  [unwired: 7 in, 1 out]
              }
              event "Magnet Current Set": Value Change {
                n87 = event-data() -> ()  [unwired: 1 in, 1 out]
                n88 = local read "Magnet Current Set"() -> (w110:dbl)
                n89 = local read "Bias_LO_equip"() -> (w113:T2)
                n90 = local read "Control"() -> (w112:T3)
                n91 = Bundle By Name(cluster=w112, "Set_Mag_Cur"=w110) -> (w111:T3)
                n92 = local write "Control"(w111) -> ()
                n93 = call "__SIS_Mag_C_Set.vi"("Set_Mag_C"=w110, "Bias_LO_equip"=w113) -> ()  [unwired: 10 in]
              }
              event "HOT/COLD": Value Change {
                n94 = event-data() -> ()  [unwired: 1 in, 6 out]
                n95 = stacked-sequence {
                  seq-local: [w114 _] -> [_ w176]
                  frame #0 {
                    n96 = property on="HOT" class="Bool (엄격한)"() -> ("Value"=w114:bool)  [unwired: 2 in, 2 out]
                    n97 = case shown="참" w114 {
                      frame False {
                        # "Monitor cold"
                        n98 = local read "Control"() -> (w115:T3)
                        n99 = Unbundle By Name(w115) -> ("HOT/COLD"=w116:u16)
                        n100 = case shown="2" w116 {
                          tunnel: w115 -> [w121 w125 w136]
                          tunnel: -50.0 -> [w118 w123 w134]
                          frame 0, Default {
                            n101 = Unbundle By Name(w121) -> ("motor setting"=w120:T33)
                            n102 = Index Array(array=w120, index=0) -> (element=w119:T34)
                            n103 = call "__move_motor2.vi"("Moving distance"=w118, "motor setup"=w119) -> ()  [unwired: 2 in, 2 out]
                          }
                          frame 1 {
                            n104 = Unbundle By Name(w125) -> ("motor setting"=w124:T33)
                            n105 = stacked-sequence {
                              tunnel: w124 -> [w128 w132]
                              tunnel: w123 -> [w126 w130]
                              frame #0 {
                                n106 = Index Array(array=w128, index=2) -> (element=w127:T34)
                                n107 = call "__move_motor2.vi"("Moving distance"=w126, "motor setup"=w127) -> ()  [unwired: 2 in, 2 out]
                              }
                              frame #1 {
                                n108 = Index Array(array=w132, index=3) -> (element=w131:T34)
                                n109 = call "__move_motor2.vi"("Moving distance"=w130, "motor setup"=w131) -> ()  [unwired: 2 in, 2 out]
                              }
                            }
                          }
                          frame 2 {
                            n110 = Unbundle By Name(w136) -> ("motor setting"=w135:T33)
                            n111 = stacked-sequence {
                              tunnel: w135 -> [w139 w143]
                              tunnel: w134 -> [w137 w141]
                              frame #0 {
                                n112 = Index Array(array=w139, index=4) -> (element=w138:T34)
                                n113 = call "__move_motor2.vi"("Moving distance"=w137, "motor setup"=w138) -> ()  [unwired: 2 in, 2 out]
                              }
                              frame #1 {
                                n114 = Index Array(array=w143, index=5) -> (element=w142:T34)
                                n115 = call "__move_motor2.vi"("Moving distance"=w141, "motor setup"=w142) -> ()  [unwired: 2 in, 2 out]
                              }
                            }
                          }
                        }
                      }
                      frame True {
                        # "Monitor Hot"
                        # "Monitor"
                        n116 = local read "Control"() -> (w145:T3)
                        n117 = Unbundle By Name(w145) -> ("HOT/COLD"=w146:u16)
                        n118 = case shown="2" w146 {
                          tunnel: w145 -> [w151 w155 w166]
                          tunnel: 50.0 -> [w148 w153 w164]
                          frame 0, Default {
                            n119 = Unbundle By Name(w151) -> ("motor setting"=w150:T33)
                            n120 = Index Array(array=w150, index=0) -> (element=w149:T34)
                            n121 = call "__move_motor2.vi"("Moving distance"=w148, "motor setup"=w149) -> ()  [unwired: 2 in, 2 out]
                          }
                          frame 1 {
                            n122 = Unbundle By Name(w155) -> ("motor setting"=w154:T33)
                            n123 = stacked-sequence {
                              tunnel: w154 -> [w158 w162]
                              tunnel: w153 -> [w156 w160]
                              frame #0 {
                                n124 = Index Array(array=w158, index=2) -> (element=w157:T34)
                                n125 = call "__move_motor2.vi"("Moving distance"=w156, "motor setup"=w157) -> ()  [unwired: 2 in, 2 out]
                              }
                              frame #1 {
                                n126 = Index Array(array=w162, index=3) -> (element=w161:T34)
                                n127 = call "__move_motor2.vi"("Moving distance"=w160, "motor setup"=w161) -> ()  [unwired: 2 in, 2 out]
                              }
                            }
                          }
                          frame 2 {
                            n128 = Unbundle By Name(w166) -> ("motor setting"=w165:T33)
                            n129 = stacked-sequence {
                              tunnel: w165 -> [w169 w173]
                              tunnel: w164 -> [w167 w171]
                              frame #0 {
                                n130 = Index Array(array=w169, index=4) -> (element=w168:T34)
                                n131 = call "__move_motor2.vi"("Moving distance"=w167, "motor setup"=w168) -> ()  [unwired: 2 in, 2 out]
                              }
                              frame #1 {
                                n132 = Index Array(array=w173, index=5) -> (element=w172:T34)
                                n133 = call "__move_motor2.vi"("Moving distance"=w171, "motor setup"=w172) -> ()  [unwired: 2 in, 2 out]
                              }
                            }
                          }
                        }
                      }
                    }
                  }
                  frame #1 {
                    n134 = Not(x=w176) -> (.not. x?=w175:bool)
                    n135 = property on="HOT" class="Bool (엄격한)"("Val(Sgnl)"=w175) -> ()  [unwired: 2 in, 2 out]
                  }
                }
              }
              event "Zero Int": Value Change {
                n136 = event-data() -> ()  [unwired: 1 in, 6 out]
                n137 = local read "Bias_LO_equip"() -> (w182:T2)
                n138 = local read "Zero Int"() -> (w178:bool)
                n139 = Unbundle By Name(w182) -> ("ObjHandle out"=w181:u32, "Slave Node in"=w180:cluster{"Address":i16, "Serial Number":i8[]}, "Cartridge band"=w179:u32)
                n140 = case shown="참" w178 {
                  tunnel: [0 1] -> w177
                  frame False {
                  }
                  frame True {
                  }
                }
                n141 = call "WCA_SET_NULL_PLL_INTEGRATOR.vi"("Cartridge Band"=w179, "Slave Node in"=w180, "ObjHandle in"=w181, "SET_NULL_PLL_INTEGRATOR"=w177) -> ()  [unwired: 10 in, 2 out]
              }
              event "Vmin", "VMax": Value Change {
                n142 = event-data() -> ()  [unwired: 1 in, 6 out]
                n143 = property on="SISSetVolt" class="Slide (엄격한)"("Scale.Minimum"="Vmin", "Scale.Maximum"="VMax") -> ()  [unwired: 2 in, 2 out]
                n144 = property on="XY graph" class="XYGraph (엄격한)"("XScale.Minimum"="Vmin", "XScale.Maximum"="VMax") -> ()  [unwired: 2 in, 2 out]
              }
              event "WCA Pol": Value Change {
                n145 = event-data() -> ("OldVal"=w190:u16, "NewVal"=w189:u16)  [unwired: 1 in, 4 out]
                n146 = local read "Bias_LO_equip"() -> (w188:T2)
                n147 = Unbundle By Name(w188) -> ("BiasModule"=w187:u16)
                n148 = case shown="1" w187 {
                  tunnel: w190 -> [_ w192]
                  tunnel: w189 -> [_ w191]
                  frame 0, Default {
                  }
                  frame 1 {
                    n149 = stacked-sequence {
                      tunnel: w192 -> [w194 _ _]
                      tunnel: w191 -> [_ w204 w221]
                      frame #0 {
                        n150 = local read "SISSetVolt"() -> (w201:dbl)
                        n151 = local read "Magnet Current Set"() -> (w197:dbl)
                        n152 = local read "initial value"() -> (w203:dbl[][])
                        n153 = local read "Offset"() -> (w200:dbl)
                        n154 = Replace Array Subset(array=w203, new element=w201, index (row)=w194, index (col)=0) -> (w196:dbl[][])
                        n155 = Replace Array Subset(array=w196, new element=w200, index (row)=w194, index (col)=1) -> (w195:dbl[][])
                        n156 = Replace Array Subset(array=w195, new element=w197, index (row)=w194, index (col)=2) -> (w193:dbl[][])
                        n157 = local write "initial value"(w193) -> ()
                      }
                      frame #1 {
                        n158 = local read "Bias_LO_equip"() -> (w208:T2)
                        n159 = case shown="0, 1" w204 {
                          tunnel: [1 1 2] -> w206
                          frame Default {
                          }
                          frame 0, 1 {
                          }
                          frame 2, 3 {
                          }
                        }
                        n160 = case shown="1, 3" w204 {
                          tunnel: [1 0 1] -> w205
                          frame Default {
                          }
                          frame 0, 2 {
                          }
                          frame 1, 3 {
                          }
                        }
                        n161 = Bundle By Name(cluster=w208, "POL"=w205, "sb"=w206) -> (w207:T2)
                        n162 = local write "Bias_LO_equip"(w207) -> ()
                      }
                      frame #2 {
                        n163 = local read "initial value"() -> (w222:dbl[][])
                        n164 = Index Array(array=w222, index (row)=w221, index (col)=0) -> (element=w218:dbl)
                        n165 = Index Array(array=w222, index (row)=w221, index (col)=2) -> (element=w216:dbl)
                        n166 = Index Array(array=w222, index (row)=w221, index (col)=1) -> (element=w217:dbl)
                        n167 = local write "SISSetVolt"(w218) -> ()
                        n168 = local write "Offset"(w217) -> ()
                        n169 = local write "Magnet Current Set"(w216) -> ()
                        n170 = local read "Control"() -> (w219:T3)
                        n171 = Bundle By Name(cluster=w219, "Set_SIS_volt"=w218, "Offset"=w217, "Set_Mag_Cur"=w216) -> (w215:T3)
                        n172 = local write "Control"(w215) -> ()
                      }
                    }
                  }
                }
              }
            }
          }
          frame #1 {
            n173 = case shown="참" "Set CLNA" {
              frame False {
              }
              frame True {
                n174 = local read "Bias_LO_equip"() -> (w238:T2)
                n175 = Unbundle By Name(w238) -> ("Slave Node in"=w233:cluster{"Address":i16, "Serial Number":i8[]}, "ObjHandle out"=w237:u32, "Cartridge band"=w236:u32, "sb"=w235:u32, "POL"=w232:u32)
                n176 = local write "Set CLNA"(FALSE) -> ()
                n177 = local read "CLNA_SET"() -> (w231:T4)
                n178 = call "WCA_SET_CLNA.vi"("Cartridge Band"=w236, "Slave Node in"=w233, "ObjHandle in"=w237, "POL"=w232, "sb"=w235, "CLNA_SET"=w231) -> ()  [unwired: 8 in, 2 out]
              }
            }
            n179 = case shown="참" "CLNA Sweep" {
              frame False {
              }
              frame True {
                n180 = local read "Bias_LO_equip"() -> (w229:T2)
                n181 = local read "CLNAsweep"() -> (w228:T6)
                n182 = local read "Control"() -> (w230:T3)
                n183 = call "_WCA_CLNA_Sweep.vi"("CLNAsweep"=w228, "Control"=w230, "Bias_LO_equip"=w229) -> ()  [unwired: 9 in]
                n184 = local write "CLNA Sweep"(FALSE) -> ()
              }
            }
          }
          frame #2 {
            n185 = case shown="참" "I-V sweep" {
              frame False {
              }
              frame True {
                n186 = stacked-sequence {
                  frame #0 {
                    n187 = local read "SISSetVolt"() -> (w243:dbl)
                    n188 = local read "SIScontrol"() -> (w245:u16)
                    n189 = local read "Offset"() -> (w246:dbl)
                    n190 = local read "i-v parameter"() -> (w242:T17)
                    n191 = local read "Control"() -> (w241:T3)
                    n192 = Bundle By Name(cluster=w241, "control"=w245, "Offset"=w246, "Set_SIS_volt"=w243) -> (w240:T3)
                    n193 = local read "Bias_LO_equip"() -> (w249:T2)
                    n194 = Unbundle By Name(w242) -> ("number of Sweep"=w244:u16)
                    n195 = local write "i-v parameter"(w242) -> ()
                    n196 = local write "Control"(w240) -> ()
                    n197 = case shown="1, 2" w244 {
                      tunnel: w249 -> [w253 w257]
                      tunnel: [w255 w260] -> w248
                      tunnel: [w254 w259] -> w247
                      tunnel: w242 -> [w252 w258]
                      tunnel: w240 -> [w251 w256]
                      frame 1, 2 {
                        n198 = call "_iv_AUTO3.vi"("i-v class"=w252, "Control"=w251, "Bias_LO_equip"=w253) -> ("Set_SIS_volt"=w250:dbl, "XY graph 3"=w254:cluster{dbl[], dbl[]}, "XY graph 2"=w255:cluster{dbl[], dbl[]})  [unwired: 1 in, 1 out]
                        n199 = local write "SISSetVolt"(w250) -> ()
                      }
                      frame 0, Default {
                        n200 = call "_get_iv_sweep3.vi"("I-V class"=w258, "Control"=w256, "Bias_LO_equip"=w257) -> ("VP class"=w259:cluster{"array":dbl[], "array2":dbl[]}, "VI class"=w260:cluster{"array":dbl[], "array2":dbl[]})  [unwired: 2 in, 1 out]
                      }
                    }
                    "VI Class" <- w248
                    "VP Class" <- w247
                  }
                  frame #1 {
                    n201 = local read "Bias_LO_equip"() -> (w262:T2)
                    n202 = local read "SISSetVolt"() -> (w264:dbl)
                    n203 = local read "Offset"() -> (w263:dbl)
                    n204 = call "__SISbias_Set.vi"("Offset"=w263, "Set_V"=w264, "Bias_LO_equip"=w262) -> ()  [unwired: 8 in, 1 out]
                    n205 = local write "I-V sweep"(FALSE) -> ()
                  }
                }
              }
            }
          }
          frame #3 {
            n206 = case shown="참" "LOP optimize" {
              frame False {
              }
              frame True {
                n207 = local read "SISSetVolt"() -> (w271:dbl)
                n208 = local read "_LO_P_OPT"() -> (w269:T14)
                n209 = local read "Control"() -> (w272:T3)
                n210 = local read "Bias_LO_equip"() -> (w267:T2)
                n211 = Unbundle By Name(w267) -> ("LOModule"=w266:u16)
                n212 = Bundle By Name(cluster=w272, "Set_SIS_volt"=w271) -> (w270:T3)
                n213 = call "_LO_P_OPT2.vi"("_LO_P_OPT"=w269, "Control"=w270, "Bias_LO_equip"=w267) -> ("Œ‹‰Ê"=w268:string)  [unwired: 4 in]
                n214 = case shown="0, 2, 5..7" w266 {
                  selector: w266 -> [w277 _]
                  tunnel: w268 -> [w283 _]
                  tunnel: w267 -> [w280 _]
                  frame 0, 2, 5..7 {
                    n215 = Unbundle By Name(w280) -> ("POL"=w281:u32)
                    n216 = Scan From String(format string="LOPt,%f,%f,%s", input string=w283) -> (output 2=w276:dbl)  [unwired: 7 in, 3 out]
                    n217 = local read "PA V"() -> (w278:cluster{"VD":dbl, "VG ":dbl, "String":string}[])
                    n218 = case shown="2" w277 {
                      tunnel: w281 -> [_ w291]
                      tunnel: [w287 w291] -> w279
                      tunnel: w278 -> [w288 w292]
                      tunnel: w276 -> [w285 w290]
                      tunnel: [w284 w289] -> w275
                      frame 0, 5..7, Default {
                        w287 = 2
                        n219 = Index Array(array=w288, index=w287) -> (element=w286:cluster{"VD":dbl, "VG ":dbl, "String":string})
                        n220 = Bundle By Name(cluster=w286, "VG"=w285) -> (w284:cluster{"VD":dbl, "VG ":dbl, "String":string})
                      }
                      frame 2 {
                        n221 = Index Array(array=w292, index=w291) -> (element=w293:cluster{"VD":dbl, "VG ":dbl, "String":string})
                        n222 = Bundle By Name(cluster=w293, "VD"=w290) -> (w289:cluster{"VD":dbl, "VG ":dbl, "String":string})
                      }
                    }
                    n223 = Replace Array Subset(array=w278, new element=w275, index=w279) -> (w274:cluster{"VD":dbl, "VG ":dbl, "String":string}[])
                    n224 = local write "PA V"(w274) -> ()
                  }
                  frame 1, Default {
                  }
                }
                n225 = local write "Control"(w270) -> ()
                n226 = local write "LOP optimize"(FALSE) -> ()
              }
            }
          }
          frame #4 {
            n227 = case shown="참" "IFBOXSet" {
              frame False {
              }
              frame True {
                n228 = local read "Control"() -> (w296:T3)
                n229 = local read "IFBOX"() -> (w298:T16)
                n230 = Unbundle By Name(w296) -> ("6501Dev#"=w295:i16)
                n231 = call "_IFBOX_CNT.vi"("6501Dev#"=w295, "IFBOX"=w298) -> ()  [unwired: 6 in]
                n232 = local write "IFBOXSet"(FALSE) -> ()
              }
            }
          }
          frame #5 {
            n233 = case shown="참" "Start allan" {
              frame False {
              }
              frame True {
                n234 = local read "allan"() -> (w319:T20)
                n235 = call "_allan_Variance_Ver6.vi"("allanÝèA"=w319) -> ()  [unwired: 7 in]
                n236 = local write "Start allan"(FALSE) -> ()
              }
            }
            n237 = case shown="참" "GainComp" {
              frame False {
              }
              frame True {
                n238 = local read "GC_LockinAmp"() -> (w316:T19)
                n239 = local read "Bias_LO_equip"() -> (w318:T2)
                n240 = local read "Control"() -> (w317:T3)
                n241 = call "_GainComp_LockInAmp_2.vi"("GC_LockinAmp"=w316, "Control"=w317, "Bias_LO_equip"=w318) -> ()  [unwired: 8 in, 1 out]
                n242 = local write "GainComp"(FALSE) -> ()
              }
            }
            n243 = case shown="참" "CrossTalk" {
              frame False {
              }
              frame True {
                n244 = local read "Bias_LO_equip"() -> (w314:T2)
                n245 = local read "Control"() -> (w312:T3)
                n246 = local read "PA V"() -> (w309:cluster{"VD":dbl, "VG ":dbl, "String":string}[])
                n247 = local read "CrossTalk_mkpk"() -> (w311:T18)
                n248 = local read "_LO_P_OPT"() -> (w310:T14)
                n249 = call "_crosstalk_mkpk.vi"("Bias_LO_equip"=w314, "Control"=w312, "CrossTalk_mkpk"=w311, "PAV”z—ñ"=w309, "_LO_P_OPT"=w310) -> ()  [unwired: 5 in, 1 out]
                n250 = local write "CrossTalk"(FALSE) -> ()
              }
            }
            n251 = case shown="참" "LO Harmonic" {
              frame False {
              }
              frame True {
                n252 = local read "Bias_LO_equip"() -> (w307:T2)
                n253 = local read "PA V"() -> (w304:cluster{"VD":dbl, "VG ":dbl, "String":string}[])
                n254 = local read "Control"() -> (w306:T3)
                n255 = local read "LO harmonic"() -> (w305:T21)
                n256 = local read "_LO_P_OPT"() -> (w303:T14)
                n257 = local write "LO Harmonic"(FALSE) -> ()
                n258 = call "_LOharmonic.vi"("Bias_LO_equip"=w307, "Control"=w306, "LOhharmonic"=w305, "PAV”z—ñ"=w304, "_LO_P_OPT"=w303) -> ()  [unwired: 5 in, 1 out]
              }
            }
          }
          frame #6 {
            n259 = case shown="참" "Set LO freq" {
              frame False {
              }
              frame True {
                n260 = local read "Bias_LO_equip"() -> (w325:T2)
                n261 = local read "LO_misc"() -> (w323:T11)
                n262 = call "_Set_LO_frq_B10_WCA.vi"("Bias_LO_equip"=w325, "LO_misc"=w323) -> ("Bias_LO_equip 2"=w324:T35, "LO_misc 2"=w326:T11)  [unwired: 15 in, 1 out]
                n263 = local write "Bias_LO_equip"(w324) -> ()
                n264 = local write "LO_misc"(w326) -> ()
                n265 = Unbundle By Name(w326) -> ("LO FRQ(GHz)"=w328:dbl)
                n266 = local read "Control"() -> (w327:T3)
                n267 = local write "Set LO freq"(FALSE) -> ()
                n268 = Bundle By Name(cluster=w327, "FreqLO"=w328) -> (w329:T3)
                n269 = local write "Control"(w329) -> ()
              }
            }
          }
          frame #7 {
            n270 = case shown="참" "SISparam" {
              frame False {
              }
              frame True {
                n271 = local read "_LO_P_OPT"() -> (w333:T14)
                n272 = local read "Bias_LO_equip"() -> (w339:T2)
                n273 = local read "Control"() -> (w338:T3)
                n274 = local write "SISparam"(FALSE) -> ()
                n275 = call "_set_mixer_params.vi"("_LO_P_OPT"=w333, "Control"=w338, "Bias_LO_equip"=w339) -> ("•¶Žš—ñ"=w336:string, "Control 2"=w334:T36, "Bias_LO_equip 2"=w335:T35)  [unwired: 6 in]
                n276 = Unbundle By Name(w333) -> ("SISparam option"=w332:u16)
                n277 = local write "Buffer"(w336) -> ()
                n278 = local write "Bias_LO_equip"(w335) -> ()
                n279 = local write "Control"(w334) -> ()
                n280 = case shown="1, 기본" w332 {
                  tunnel: w336 -> [_ w349]
                  tunnel: w335 -> [_ w347]
                  tunnel: w334 -> [_ w342]
                  frame 1, Default {
                  }
                  frame 0 {
                    n281 = Unbundle By Name(w347) -> ("LOModule"=w346:u16, "POL"=w345:u32)
                    n282 = Scan From String(format string="LOPt,%f,%f,%s", input string=w349) -> (output 2=w343:dbl)  [unwired: 7 in, 3 out]
                    n283 = Unbundle By Name(w342) -> ("Set_SIS_volt"=w341:dbl, "Offset"=w340:dbl)
                    n284 = local read "PA V"() -> (w344:cluster{"VD":dbl, "VG ":dbl, "String":string}[])
                    n285 = case shown="2" w346 {
                      tunnel: w345 -> [w352 _ _]
                      tunnel: w344 -> [w354 w359 _]
                      tunnel: w343 -> [w350 w360 _]
                      frame 2 {
                        n286 = Index Array(array=w354, index=w352) -> (element=w355:cluster{"VD":dbl, "VG ":dbl, "String":string})
                        n287 = Bundle By Name(cluster=w355, "VD"=w350) -> (w353:cluster{"VD":dbl, "VG ":dbl, "String":string})
                        n288 = Replace Array Subset(array=w354, new element=w353, index=w352) -> (w351:cluster{"VD":dbl, "VG ":dbl, "String":string}[])
                        n289 = local write "PA V"(w351) -> ()
                      }
                      frame 5..7 {
                        w356 = 2
                        n290 = Index Array(array=w359, index=w356) -> (element=w361:cluster{"VD":dbl, "VG ":dbl, "String":string})
                        n291 = Bundle By Name(cluster=w361, "VG"=w360) -> (w358:cluster{"VD":dbl, "VG ":dbl, "String":string})
                        n292 = Replace Array Subset(array=w359, new element=w358, index=w356) -> (w357:cluster{"VD":dbl, "VG ":dbl, "String":string}[])
                        n293 = local write "PA V"(w357) -> ()
                      }
                      frame 8, Default {
                      }
                    }
                    n294 = local write "SISSetVolt"(w341) -> ()
                    n295 = local write "Offset"(w340) -> ()
                  }
                }
              }
            }
            n296 = case shown="참" "Set LO PAMP" {
              frame False {
              }
              frame True {
                n297 = local read "Bias_LO_equip"() -> (w364:T2)
                n298 = local read "PA V"() -> (w363:cluster{"VD":dbl, "VG ":dbl, "String":string}[])
                n299 = local write "Set LO PAMP"(FALSE) -> ()
                n300 = call "_LO_PAMP_set.vi"("PAV”z—ñ"=w363, "Bias_LO_equip"=w364) -> ()  [unwired: 10 in]
              }
            }
          }
          frame #8 {
            n301 = case shown="참" "SPmeasuremnt" {
              frame False {
              }
              frame True {
                n302 = local read "spectrum_data"() -> (w368:T22)
                n303 = local read "Bias_LO_equip"() -> (w366:T2)
                n304 = local read "Control"() -> (w367:T3)
                n305 = call "_sp3.vi"("sp_data"=w368, "Control"=w367, "Bias_LO_equip"=w366) -> ()  [unwired: 5 in]
                n306 = local write "SPmeasuremnt"(FALSE) -> ()
              }
            }
          }
          frame #9 {
            n307 = case shown="참" "LO_SWEEP" {
              frame False {
              }
              frame True {
                n308 = local read "Bias_LO_equip"() -> (w374:T2)
                n309 = local read "_LO_sweep"() -> (w372:T15)
                n310 = local read "LO_misc"() -> (w373:T11)
                n311 = call "_LO_freq_Sweep.vi"("_LO_sweep"=w372, "LO_misc"=w373, "Bias_LO_equip"=w374) -> ()  [unwired: 9 in]
                n312 = local write "LO_SWEEP"(FALSE) -> ()
              }
            }
          }
          frame #10 {
            n313 = case shown="참" "Do Demag" {
              frame False {
              }
              frame True {
                n314 = local read "Bias_LO_equip"() -> (w396:T2)
                n315 = call "_Demagnetization.vi"("demag"="demag", "Bias_LO_equip"=w396) -> ()  [unwired: 10 in]
                n316 = local write "Do Demag"(FALSE) -> ()
                n317 = local write "Magnet Current Set"(0.0) -> ()
              }
            }
            n318 = case shown="참" "Ic measurement" {
              frame False {
              }
              frame True {
                n319 = local read "Joseph_curr"() -> (w397:T8)
                n320 = local read "Bias_LO_equip"() -> (w399:T2)
                n321 = local write "Ic measurement"(FALSE) -> ()
                n322 = call "_Josep_curr_Imag_2.vi"("Joseph_curr"=w397, "Bias_LO_equip"=w399) -> ()  [unwired: 10 in]
              }
            }
            n323 = case shown="참" "Heater@ON@" {
              frame False {
              }
              frame True {
                n324 = local read "SIS_Deflux_heater"() -> (w390:T10)
                n325 = local read "Bias_LO_equip"() -> (w391:T2)
                n326 = local write "Heater@ON@"(FALSE) -> ()
                n327 = call "_SIS_defux_heater.vi"("SIS_Deflux_heater"=w390, "Bias_LO_equip"=w391) -> ()  [unwired: 10 in]
              }
            }
            n328 = case shown="참" "Do shapiro" {
              frame False {
              }
              frame True {
                n329 = local read "demag"() -> (w385:T7)
                n330 = local read "Bias_LO_equip"() -> (w388:T2)
                n331 = local read "shapiro"() -> (w387:T9)
                n332 = local read "Control"() -> (w386:T3)
                n333 = local write "Do shapiro"(FALSE) -> ()
                n334 = call "_shapiro2.vi"("Bias_LO_equip"=w388, "Control"=w386, "shapiro"=w387, "demag"=w385) -> ("min Mag current"=w384:dbl)  [unwired: 6 in]
                n335 = local write "Magnet Current Set"(w384) -> ()
              }
            }
            n336 = case shown="참" "Nitsuki_TDP_Command" {
              frame False {
              }
              frame True {
                n337 = local write "Nitsuki_TDP_Command"(FALSE) -> ()
                n338 = call "_Nitsuki_TPD_control_send.vi"("send"="send", "control IP"="control IP") -> ("Their Response:"=→"Their Response":string)  [unwired: 8 in, 1 out]
              }
            }
          }
          frame #11 {
            n339 = case shown="참" "run script" {
              frame False {
              }
              frame True {
                n340 = stacked-sequence {
                  frame #0 {
                    w401 = 0
                    n341 = local write "MOSL"(w401) -> ()
                    n342 = local read "program"() -> (w407:cluster{"Cord":u16, "Option":string}[])
                    n343 = Array Size(array=w407) -> (size(s)=w403:i32)
                    n344 = local read "MOS"() -> (w406:T27)
                    n345 = Index Array(array=w406, index=w401) -> (element=w404:T37)
                    n346 = Bundle By Name(cluster=w404, "number of lines"=w403) -> (w402:T37)
                    n347 = Replace Array Subset(array=w406, new element=w402, index=w401) -> (w405:T27)
                    n348 = local write "MOS"(w405) -> ()
                  }
                  frame #1 {
                    n349 = while {
                      shift-right: [w409] -> _
                      shift-left: 0 -> [w411]
                      stop <- w410 stop-if-true
                      n350 = stacked-sequence {
                        seq-local: [w419 _ _] -> [_ w425 _]
                        seq-local: [w418 _ _] -> [_ w426 _]
                        seq-local: [_ w423 _] -> [_ _ w1605]
                        seq-local: [_ w422 _] -> [_ _ w1615]
                        tunnel: w411 -> [w412 w424 _]
                        tunnel: [_ _ w1608] -> w410
                        tunnel: [_ _ w1606] -> w409
                        frame #0 {
                          n351 = local read "program"() -> (w420:cluster{"Cord":u16, "Option":string}[])
                          n352 = Index Array(array=w420, index=w412) -> (element=w421:cluster{"Cord":u16, "Option":string})
                          n353 = Unbundle By Name ("名前でバンドル解除")(w421) -> ("Cord"=w419:u16, "Option"=w418:string)
                          n354 = local read "MOSL"() -> (w416:i32)
                          n355 = local read "MOS"() -> (w415:T27)
                          n356 = Index Array(array=w415, index=w416) -> (element=w417:T37)
                          n357 = Bundle By Name(cluster=w417, "run number"=w412) -> (w414:T37)
                          n358 = Replace Array Subset(array=w415, new element=w414, index=w416) -> (w413:T27)
                          n359 = local write "MOS"(w413) -> ()
                        }
                        frame #1 {
                          n360 = case shown="220" w425 {
                            tunnel: w426 -> [_ w440 _ _ w472 w477 w480 w487 w496 w502 _ w531 _ _ _ _ _ w596 w656 w666 w702 w714 w720 w727 w743 w765 _ w794 w813 w825 w838 w851 w863 w880 w888 w905 w924 w953 w983 w1016 w1051 w1077 w1096 w1119 w1154 w1163 w1183 w1196 w1216 _ _ _ w1279 w1297 _ w1320 _ _ _ _ _ _ w1399 w1405 _ w1424 w1448 w1461 _ w1474 _ w1512 w1524 _ _ w1600]
                            tunnel: w424 -> [w429 w438 w448 w462 w470 w475 w483 w490 w499 w505 w519 w543 w554 w558 w567 w576 w593 w598 w661 w670 w707 w718 w724 w731 w747 w770 w783 w798 w817 w829 w842 w855 w867 w884 w892 w909 w928 w957 w987 w1020 w1055 w1081 w1100 w1123 w1158 w1172 w1187 w1209 w1220 w1239 w1253 w1270 w1290 w1301 w1313 w1330 w1336 w1342 w1348 w1361 w1374 w1388 w1403 w1416 w1420 w1427 w1451 w1465 w1468 w1477 w1501 w1515 w1527 w1566 w1585 w1604]
                            tunnel: [w428 w441 w450 w462 w473 w476 w482 w489 w498 w504 w518 w542 w553 w557 w566 w575 w592 w594 w660 w669 w706 w717 w723 w730 w746 w769 w782 w797 w816 w828 w841 w854 w866 w883 w891 w908 w927 w956 w986 w1019 w1054 w1080 w1099 w1122 w1157 w1171 w1186 w1208 w1219 w1238 w1252 w1269 w1289 w1300 w1312 w1329 w1335 w1341 w1347 w1360 w1373 w1387 w1402 w1415 w1419 w1426 w1450 w1464 w1467 w1476 w1500 w1514 w1526 w1565 w1584 w1603] -> w423
                            tunnel: [FALSE _ _ TRUE _ FALSE FALSE FALSE FALSE FALSE FALSE FALSE FALSE FALSE FALSE FALSE FALSE FALSE FALSE FALSE FALSE FALSE FALSE FALSE FALSE FALSE FALSE FALSE FALSE FALSE FALSE FALSE FALSE FALSE FALSE FALSE FALSE FALSE FALSE FALSE FALSE FALSE FALSE FALSE FALSE FALSE FALSE FALSE FALSE FALSE FALSE FALSE FALSE FALSE FALSE FALSE FALSE FALSE FALSE FALSE FALSE FALSE FALSE FALSE FALSE FALSE FALSE FALSE FALSE FALSE FALSE FALSE FALSE FALSE FALSE FALSE] -> w422
                            frame 1, Default {
                              # "スクリプトのコメント処理\n何もしない"
                              n361 = Increment(x=w429) -> (x+1=w428:i32)
                            }
                            frame 2 {
                              # "LOOP"
                              n362 = Increment(x=w438) -> (x+1=w441:i32)
                              n363 = local read "MOSL"() -> (w433:i32)
                              n364 = Scan From String(format string="%f,%f,%f", input string=w440) -> (output 1=w437:dbl, output 2=w436:dbl, output 3=w435:dbl)  [unwired: 5 in, 3 out]
                              n365 = local read "MOS"() -> (w432:T27)
                              n366 = Index Array(array=w432, index=w433) -> (element=w434:T37)
                              n367 = Bundle By Name(cluster=w434, "Line number"=w438, "Lupu's numerical value"=w437, "Lupe Stop"=w436, "Lupe Step"=w435) -> (w431:T37)
                              n368 = Replace Array Subset(array=w432, new element=w431, index=w433) -> (w430:T27)
                              n369 = local write "MOS"(w430) -> ()
                            }
                            frame 3 {
                              # "Next"
                              n370 = local read "MOS"() -> (w442:T27)
                              n371 = local read "MOSL"() -> (w443:i32)
                              n372 = Index Array(array=w442, index=w443) -> (element=w444:T37)
                              n373 = Unbundle By Name(w444) -> ("Lupu's numerical value"=w447:dbl, "Lupe Step"=w446:dbl, "Lupe Stop"=w445:dbl)
                              n374 = Add(x=w447, y=w446) -> (x+y=w449:dbl)
                              n375 = Less Or Equal?(x=w449, y=w445) -> (x <= y?=w451:bool)
                              n376 = case shown="참" w451 {
                                tunnel: [w452 w461] -> w450
                                tunnel: w449 -> [_ w460]
                                tunnel: w448 -> [w453 _]
                                tunnel: w444 -> [_ w457]
                                tunnel: w443 -> [_ w458]
                                tunnel: w442 -> [_ w455]
                                frame False {
                                n377 = Increment(x=w453) -> (x+1=w452:i32)
                                }
                                frame True {
                                n378 = Unbundle By Name(w457) -> ("Line number"=w459:i32)
                                n379 = Bundle By Name(cluster=w457, "Lupu's numerical value"=w460) -> (w456:T37)
                                n380 = Increment(x=w459) -> (x+1=w461:i32)
                                n381 = Replace Array Subset(array=w455, new element=w456, index=w458) -> (w454:T27)
                                n382 = local write "MOS"(w454) -> ()
                                }
                              }
                            }
                            frame 4 {
                              # "END"
                            }
                            frame 5 {
                              # "set LOOP num"
                              n383 = Increment(x=w470) -> (x+1=w473:i32)
                              n384 = local read "MOSL"() -> (w467:i32)
                              n385 = Scan From String(format string="%f", input string=w472) -> (output 1=w469:dbl)  [unwired: 3 in, 3 out]
                              n386 = local read "MOS"() -> (w466:T27)
                              n387 = Index Array(array=w466, index=w467) -> (element=w468:T37)
                              n388 = Bundle By Name(cluster=w468, "Lupu's numerical value"=w469) -> (w465:T37)
                              n389 = Replace Array Subset(array=w466, new element=w465, index=w467) -> (w464:T27)
                              n390 = local write "MOS"(w464) -> ()
                            }
                            frame 6 {
                              # "jump"
                              n391 = Decimal String To Number(string=w477) -> (number=w474:i32)  [unwired: 2 in, 1 out]
                              n392 = Add(x=w475, y=w474) -> (x+y=w476:i32)
                            }
                            frame 11 {
                              # "Wait"
                              n393 = Increment(x=w483) -> (x+1=w482:i32)
                              n394 = Decimal String To Number(string=w480) -> (number=w479:i32)  [unwired: 2 in, 1 out]
                              n395 = Wait (ms)(milliseconds to wait=w479) -> ()  [unwired: 1 out]
                            }
                            frame 13 {
                              # "Comment"
                              n396 = case shown="\"-9999\"" w487 {
                                tunnel: w487 -> [_ w492]
                                tunnel: [w491 w492] -> w484
                                frame "-9999" {
                                n397 = local read "Buffer"() -> (w491:string)
                                }
                                frame "True", Default {
                                }
                              }
                              n398 = Increment(x=w490) -> (x+1=w489:i32)
                              n399 = local read "Control"() -> (w485:T3)
                              n400 = Bundle By Name(cluster=w485, "comment"=w484) -> (w486:T3)
                              n401 = local write "Control"(w486) -> ()
                            }
                            frame 14 {
                              # "Cartrige SN"
                              n402 = case shown="\"-9999\"" w496 {
                                tunnel: w496 -> [_ w501]
                                tunnel: [w500 w501] -> w493
                                frame "-9999" {
                                n403 = local read "Buffer"() -> (w500:string)
                                }
                                frame "True", Default {
                                }
                              }
                              n404 = Increment(x=w499) -> (x+1=w498:i32)
                              n405 = local read "Control"() -> (w494:T3)
                              n406 = Bundle By Name(cluster=w494, "Carteidge SN"=w493) -> (w495:T3)
                              n407 = local write "Control"(w495) -> ()
                            }
                            frame 15 {
                              # "Pause"
                              n408 = Increment(x=w505) -> (x+1=w504:i32)
                              n409 = One Button Dialog(message=w502) -> ()  [unwired: 1 in, 1 out]
                            }
                            frame 16 {
                              # "SelectDir"
                              n410 = local read "Control"() -> (w507:T3)
                              n411 = Unbundle By Name(w507) -> ("DATA path"=w506:path)
                              n412 = Increment(x=w519) -> (x+1=w518:i32)
                              n413 = call "ファイルダイアログ"("start path"=w506, "prompt"="select work dir", "button label"="select this dir") -> ("selected path"=w509:path, "exists"=w514:bool, "cancelled"=w516:bool)  [unwired: 9 in, 1 out]
                              n414 = Not(x=w514) -> (.not. x?=w515:bool)
                              n415 = local read "Control"() -> (w511:T3)
                              n416 = Or(x=w515, y=w516) -> (x .or. y?=w508:bool)
                              n417 = case shown="거짓" w508 {
                                tunnel: w511 -> [w522 w525]
                                tunnel: [w521 w526] -> w510
                                tunnel: w509 -> [w520 _]
                                frame False {
                                n418 = Bundle By Name(cluster=w522, "DATA path"=w520) -> (w521:T3)
                                }
                                frame True {
                                n419 = String To Path(string="c:\\data\\") -> (path=w523:path)
                                n420 = Bundle By Name(cluster=w525, "DATA path"=w523) -> (w526:T3)
                                }
                              }
                              n421 = local write "Control"(w510) -> ()
                            }
                            frame 17 {
                              w533 = string[] [","]  # operators
                              # "Text input"
                              n422 = local read "Bias_LO_equip"() -> (w536:T2)
                              n423 = Scan String For Tokens(7:w533, 8:0, 9:w531) -> (1:w530:string, 2:w534:i32, 3:w529:string)  [unwired: 3 in, 1 out]
                              n424 = local read "Control"() -> (w537:T3)
                              n425 = local read "Buffer"() -> (w538:string)
                              n426 = local read "Script path"() -> (w539:path)
                              n427 = Increment(x=w534) -> (x+1=w528:i32)
                              n428 = Increment(x=w543) -> (x+1=w542:i32)
                              n429 = String Subset(string=w529, offset (0)=w528) -> (substring=w527:string)  [unwired: 1 in]
                              n430 = call "_srcipt_text_replace.vi"("スクリプトパス"=w539, "バッファ"=w538, "Bias_LO_equip"=w536, "Control"=w537, "input"=w527) -> ("output"=w535:string)  [unwired: 6 in]
                              n431 = call "_text_input.vi"("“ü—Í•¶Žš—ñ"=w535, 11:w530) -> ("oÍ¶ñ"=w540:string)  [unwired: 9 in]
                              n432 = local write "Buffer"(w540) -> ()
                            }
                            frame 21 {
                              # "OPEN LOG"
                              n433 = local read "Control"() -> (w550:T3)
                              n434 = Unbundle By Name(w550) -> ("comment"=w546:string, "DATA path"=w549:path)
                              n435 = Increment(x=w554) -> (x+1=w553:i32)
                              n436 = Format Into String(format string="mix_log_%s.txt", w546) -> (resulting string=w545:string)  [unwired: 2 in, 1 out]
                              n437 = Build Path(base path=w549, name or relative path=w545) -> (appended path=w548:path)
                              n438 = Open/Create/Replace File(file path (use dialog)=w548, operation (0:open)=3) -> (refnum out=w544:refnum<file>)  [unwired: 4 in, 2 out]
                              n439 = local write "log_refnum"(w544) -> ()
                            }
                            frame 22 {
                              # "CLOSE LOG"
                              n440 = Increment(x=w558) -> (x+1=w557:i32)
                              n441 = local read "log_refnum"() -> (w555:refnum<file>)
                              n442 = Close File(refnum=w555) -> ()  [unwired: 1 in, 2 out]
                            }
                            frame 25 {
                              # "write LOG"
                              n443 = Increment(x=w567) -> (x+1=w566:i32)
                              n444 = local read "Buffer"() -> (w560:string)
                              n445 = local read "log_refnum"() -> (w562:refnum<file>)
                              n446 = Set File Position(refnum=w562, from (0:start)=1) -> (refnum out=w563:refnum<file>)  [unwired: 2 in, 1 out]
                              n447 = Concatenate Strings(w560, "\r") -> (w559:string)
                              n448 = Write to Text File(file (use dialog)=w563, text=w559) -> ()  [unwired: 2 in, 3 out]
                            }
                            frame 27 {
                              # "comment from log"
                              n449 = local read "Control"() -> (w569:T3)
                              n450 = Unbundle By Name(w569) -> ("DATA path"=w568:path)
                              n451 = call "File Log 5"("start path"=w568, "prompt"="OPEN LOG FILE", "pattern (all files)"="mix_log*.txt") -> ("selected path"=w571:path, "cancelled"=w570:bool)  [unwired: 9 in, 2 out]
                              n452 = Increment(x=w576) -> (x+1=w575:i32)
                              n453 = case shown="거짓" w570 {
                                tunnel: w571 -> [w577 _]
                                frame False {
                                n454 = local read "Control"() -> (w584:T3)
                                n455 = Strip Path(path=w577) -> (stripped path=w583:path, name=w581:string)
                                n456 = Scan String For Tokens(6:string[] [".txt"], 8:8, 9:w581) -> (1:w578:string)  [unwired: 3 in, 3 out]
                                n457 = Bundle By Name(cluster=w584, "comment"=w578, "DATA path"=w583) -> (w582:T3)
                                n458 = local write "Control"(w582) -> ()
                                }
                                frame True {
                                }
                              }
                            }
                            frame 28 {
                              # "write script file name to LOG"
                              n459 = Increment(x=w593) -> (x+1=w592:i32)
                              n460 = local read "file name"() -> (w585:string)
                              n461 = local read "log_refnum"() -> (w588:refnum<file>)
                              n462 = Set File Position(refnum=w588, from (0:start)=1) -> (refnum out=w589:refnum<file>)  [unwired: 2 in, 1 out]
                              n463 = Concatenate Strings(w585, "\r") -> (w586:string)
                              n464 = Write to Text File(file (use dialog)=w589, text=w586) -> ()  [unwired: 2 in, 3 out]
                            }
                            frame 31 {
                              # "CALL"
                              n465 = Increment(x=w598) -> (x+1=w595:i32)
                              n466 = stacked-sequence {
                                tunnel: w595 -> [w612 _ _]
                                tunnel: w596 -> [_ w637 _]
                                tunnel: [_ 0 _] -> w594
                                frame #0 {
                                # "Saving the script"
                                n467 = local read "MOSL"() -> (w599:i32)
                                n468 = local read "program"() -> (w606:cluster{"Cord":u16, "Option":string}[])
                                n469 = local read "MOS"() -> (w608:T27)
                                n470 = Array Size(array=w606) -> (size(s)=w603:i32)
                                n471 = Index Array(array=w608, index=w599) -> (element=w609:T37)
                                n472 = for {
                                N: w603 -> [_]
                                tunnel: w606 -> [w617] mode=indexing
                                tunnel: [w613] -> w604 mode=indexing
                                n473 = Unbundle By Name(w617) -> ("Cord"=w616:u16, "Option"=w614:string)
                                n474 = Number To Decimal String(number=w616) -> (decimal integer string=w615:string)  [unwired: 1 in]
                                n475 = Build Array(w615, w614) -> (w613:string[])
                                }
                                n476 = Bundle By Name(cluster=w609, "run number"=w612) -> (w610:T37)
                                n477 = local read "Script path"() -> (w602:path)
                                n478 = Format Into String(format string="MOS_SUB%d.tmp", w599) -> (resulting string=w600:string)  [unwired: 2 in, 1 out]
                                n479 = Replace Array Subset(array=w608, new element=w610, index=w599) -> (w611:T27)
                                n480 = local write "MOS"(w611) -> ()
                                n481 = Build Path(base path=w602, name or relative path=w600) -> (appended path=w607:path)
                                n482 = call-poly <vilib>:"Write To Spreadsheet File.vi"("delimiter (\\t)"="@@@", "2D data"=w604, "file path (dialog if empty)"=w607) -> ()  [unwired: 5 in, 1 out]
                                }
                                frame #1 {
                                w634 = string[] [","]  # operators
                                # "Sub-script read in"
                                # "sub-script options are in the file"
                                n483 = local read "MOSL"() -> (w620:i32)
                                n484 = local read "Script path"() -> (w630:path)
                                n485 = Scan String For Tokens(7:w634, 8:0, 9:w637) -> (1:w624:string, 2:w635:i32, 3:w636:string)  [unwired: 3 in, 1 out]
                                n486 = Increment(x=w620) -> (x+1=w619:i32)
                                n487 = Build Path(base path=w630, name or relative path=w624) -> (appended path=w625:path)
                                n488 = Increment(x=w635) -> (x+1=w633:i32)
                                n489 = local write "MOSL"(w619) -> ()
                                n490 = call-poly <vilib>:"Read From Spreadsheet File.vi"("delimiter (\\t)"="@@@", "format (%s)"="%s", "file path (dialog if empty)"=w625) -> ("all rows"=w622:string[][])  [unwired: 4 in, 4 out]
                                n491 = String Subset(string=w636, offset (0)=w633) -> (substring=w631:string)  [unwired: 1 in]
                                n492 = local write "Buffer"(w631) -> ()
                                n493 = Array Size(array=w622) -> (size(s)=w628:i32[])
                                n494 = Index Array(array=w628, index=0) -> (element=w623:i32)
                                n495 = for {
                                N: w623 -> [_]
                                tunnel: w622 -> [w641] mode=indexing
                                tunnel: [w638] -> w621 mode=indexing
                                n496 = Index Array(array=w641, index=0) -> (element=w643:string)
                                n497 = Index Array(array=w641, index=1) -> (element=w639:string)
                                n498 = Decimal String To Number(string=w643) -> (number=w640:i32)  [unwired: 2 in, 1 out]
                                n499 = Bundle(w640, "String"=w639) -> (w638:cluster{i32, "String":string})  [unwired: 1 in]
                                }
                                n500 = local write "program"(w621) -> ()
                                }
                                frame #2 {
                                n501 = local read "MOSL"() -> (w646:i32)
                                n502 = local read "program"() -> (w652:cluster{"Cord":u16, "Option":string}[])
                                n503 = Array Size(array=w652) -> (size(s)=w648:i32)
                                n504 = local read "MOS"() -> (w651:T27)
                                n505 = Decrement(x=w646) -> (x-1=w645:i32)
                                n506 = Index Array(array=w651, index=w645) -> (element=w649:T37)
                                n507 = Bundle By Name(cluster=w649, "number of lines"=w648) -> (w647:T37)
                                n508 = Replace Array Subset(array=w651, new element=w647, index=w646) -> (w650:T27)
                                n509 = local write "MOS"(w650) -> ()
                                }
                              }
                            }
                            frame 102 {
                              # "Equip"
                              n510 = Scan From String(format string="%d,%d", input string=w656) -> (output 1=w655:i32, output 2=w654:i32)  [unwired: 4 in, 3 out]
                              n511 = local read "Bias_LO_equip"() -> (w658:T2)
                              n512 = Increment(x=w661) -> (x+1=w660:i32)
                              n513 = Bundle By Name(cluster=w658, "BiasModule"=w655, "LOModule"=w654) -> (w653:T2)
                              n514 = local write "Bias_LO_equip"(w653) -> ()
                            }
                            frame 103 {
                              # "POL"
                              n515 = local read "Bias_LO_equip"() -> (w665:T2)
                              n516 = Scan From String(format string="%d", input string=w666) -> (output 1=w663:i32)  [unwired: 3 in, 3 out]
                              n517 = Unbundle By Name(w665) -> ("POL"=w664:u32)
                              n518 = Equal?(x=w664, y=w663) -> (x = y?=w662:bool)
                              n519 = case shown="거짓" w662 {
                                tunnel: w663 -> [w671 _]
                                frame False {
                                n520 = stacked-sequence {
                                tunnel: w671 -> [w673 w686 w695]
                                frame #0 {
                                n521 = case shown="1" w673 {
                                tunnel: [1 0] -> w672
                                frame 0, Default {
                                }
                                frame 1 {
                                }
                                }
                                n522 = local read "SISSetVolt"() -> (w681:dbl)
                                n523 = local read "Magnet Current Set"() -> (w677:dbl)
                                n524 = local read "initial value"() -> (w683:dbl[][])
                                n525 = local read "Offset"() -> (w680:dbl)
                                n526 = Replace Array Subset(array=w683, new element=w681, index (row)=w672, index (col)=0) -> (w676:dbl[][])
                                n527 = Replace Array Subset(array=w676, new element=w680, index (row)=w672, index (col)=1) -> (w675:dbl[][])
                                n528 = Replace Array Subset(array=w675, new element=w677, index (row)=w672, index (col)=2) -> (w674:dbl[][])
                                n529 = local write "initial value"(w674) -> ()
                                }
                                frame #1 {
                                n530 = local read "Bias_LO_equip"() -> (w687:T2)
                                n531 = local write "WCA Pol"(w686) -> ()
                                n532 = Bundle By Name(cluster=w687, "POL"=w686) -> (w688:T2)
                                n533 = local write "Bias_LO_equip"(w688) -> ()
                                }
                                frame #2 {
                                n534 = local read "initial value"() -> (w696:dbl[][])
                                n535 = Index Array(array=w696, index (row)=w695, index (col)=0) -> (element=w691:dbl)
                                n536 = Index Array(array=w696, index (row)=w695, index (col)=2) -> (element=w689:dbl)
                                n537 = Index Array(array=w696, index (row)=w695, index (col)=1) -> (element=w690:dbl)
                                n538 = local write "SISSetVolt"(w691) -> ()
                                n539 = local write "Offset"(w690) -> ()
                                n540 = local read "Control"() -> (w692:T3)
                                n541 = local write "Magnet Current Set"(w689) -> ()
                                n542 = Bundle By Name(cluster=w692, "Set_SIS_volt"=w691, "Offset"=w690, "Set_Mag_Cur"=w689) -> (w693:T3)
                                n543 = local write "Control"(w693) -> ()
                                }
                                }
                                }
                                frame True {
                                }
                              }
                              n544 = Increment(x=w670) -> (x+1=w669:i32)
                            }
                            frame 105 {
                              # "LO@para"
                              n545 = Scan From String(format string="%f,%f", input string=w702) -> (output 1=w701:dbl, output 2=w700:dbl)  [unwired: 4 in, 3 out]
                              n546 = Increment(x=w707) -> (x+1=w706:i32)
                              n547 = local read "LO_misc"() -> (w704:T11)
                              n548 = Bundle By Name(cluster=w704, "LO REF multi"=w701, "SG set pow"=w700) -> (w699:T11)
                              n549 = local write "LO_misc"(w699) -> ()
                            }
                            frame 112 {
                              # "SIS@V"
                              n550 = Scan From String(format string="%d,%f", input string=w714) -> (output 1=w713:i32, output 2=w709:dbl)  [unwired: 4 in, 3 out]
                              n551 = Increment(x=w718) -> (x+1=w717:i32)
                              n552 = local write "SISSetVolt"(w709) -> ()
                              n553 = local read "Offset"() -> (w708:dbl)
                              n554 = local read "Bias_LO_equip"() -> (w712:T2)
                              n555 = local write "SIScontrol"(w713) -> ()
                              n556 = local read "Control"() -> (w711:T3)
                              n557 = Bundle By Name(cluster=w711, "Set_SIS_volt"=w709, "Offset"=w708) -> (w710:T3)
                              n558 = call "__SISbias_Set.vi"("SIS@Mode"=w713, "Offset"=w708, "Set_V"=w709, "Bias_LO_equip"=w712) -> ()  [unwired: 7 in, 1 out]
                              n559 = local write "Control"(w710) -> ()
                            }
                            frame 113 {
                              # "SIS offset"
                              n560 = Scan From String(format string="%f", input string=w720) -> (output 1=w719:dbl)  [unwired: 3 in, 3 out]
                              n561 = Increment(x=w724) -> (x+1=w723:i32)
                              n562 = local write "Offset"(w719) -> ()
                            }
                            frame 114 {
                              # "IMAG Setup"
                              n563 = Scan From String(format string="%f", input string=w727) -> (output 1=w725:dbl)  [unwired: 3 in, 3 out]
                              n564 = Increment(x=w731) -> (x+1=w730:i32)
                              n565 = local read "Bias_LO_equip"() -> (w726:T2)
                              n566 = local write "Magnet Current Set"(w725) -> ()
                              n567 = call "__SIS_Mag_C_Set.vi"("Set_Mag_C"=w725, "Bias_LO_equip"=w726) -> ()  [unwired: 10 in]
                            }
                            frame 115 {
                              # "CLNA Set 1段のみ"
                              n568 = Scan From String(format string="%f,%f", input string=w743) -> (output 1=w735:dbl, output 2=w734:dbl)  [unwired: 4 in, 3 out]
                              n569 = local read "Bias_LO_equip"() -> (w742:T2)
                              n570 = local read "CLNA_SET dummy"() -> (w736:T4)
                              n571 = Bundle By Name(cluster=w736, "CLNA State"=1, "SET POL0 LNA1 STAGE1 DRAIN V"=w735, "SET POL0 LNA1 STAGE1 DRAIN C"=w734) -> (w733:T4)
                              n572 = Increment(x=w747) -> (x+1=w746:i32)
                              n573 = Unbundle By Name(w742) -> ("Slave Node in"=w737:cluster{"Address":i16, "Serial Number":i8[]}, "ObjHandle out"=w741:u32, "Cartridge band"=w740:u32, "POL"=w739:u32, "sb"=w738:u32)
                              n574 = local write "CLNA_SET dummy"(w733) -> ()
                              n575 = call "WCA_SET_CLNA.vi"("Cartridge Band"=w740, "Slave Node in"=w737, "ObjHandle in"=w741, "POL"=w739, "sb"=w738, "CLNA_SET"=w733) -> ()  [unwired: 8 in, 2 out]
                            }
                            frame 121 {
                              # "LO@Freq"
                              n576 = local read "MOSL"() -> (w750:i32)
                              n577 = local read "MOS"() -> (w749:T27)
                              n578 = Index Array(array=w749, index=w750) -> (element=w748:T37)
                              n579 = Unbundle By Name(w748) -> ("Lupu's numerical value"=w760:dbl)
                              n580 = Scan From String(format string="%f,%d", input string=w765) -> (output 1=w761:dbl, output 2=w764:i32)  [unwired: 4 in, 3 out]
                              n581 = Greater Than 0?(x=w761) -> (x > 0?=w762:bool)
                              n582 = Increment(x=w770) -> (x+1=w769:i32)
                              n583 = Rotate Right With Carry(2:w764, 3:FALSE) -> (1:w763:bool)  [unwired: 1 out]
                              n584 = Select(t=w761, s=w762, f=w760) -> (s? t:f=w751:dbl)
                              n585 = local read "Control"() -> (w754:T3)
                              n586 = local read "LO_misc"() -> (w767:T11)
                              n587 = Bundle By Name(cluster=w767, "LO FRQ(GHz)"=w751, "LocK?"=w763) -> (w757:T11)
                              n588 = local read "Bias_LO_equip"() -> (w752:T2)
                              n589 = Unbundle By Name(w752) -> ("LOModule"=w753:u16)
                              n590 = Bundle By Name(cluster=w754, "FreqLO"=w751) -> (w755:T3)
                              n591 = local write "Control"(w755) -> ()
                              n592 = case shown="0, 5" w753 {
                                tunnel: w752 -> [_ w774]
                                tunnel: w751 -> [_ w773]
                                frame 2, Default {
                                }
                                frame 0, 5 {
                                # "GUNN NELPAMP"
                                n593 = call "_LO_GUNN_SET.vi"("ATT"=1.0, "LO_ATT"=0, "Set@\nGunn Freq"=w773, "Bias_LO_equip"=w774) -> ()  [unwired: 8 in]
                                }
                              }
                              n594 = call "_Set_LO_frq_B10_WCA.vi"("Bias_LO_equip"=w752, "LO_misc"=w757) -> ("Bias_LO_equip 2"=w759:T35, "LO_misc 2"=w758:T11)  [unwired: 15 in, 1 out]
                              n595 = local write "LO_misc"(w757) -> ()
                              n596 = local write "Bias_LO_equip"(w759) -> ()
                              n597 = local write "LO_misc"(w758) -> ()
                            }
                            frame 122 {
                              # "Dummy LO"
                              n598 = local read "MOSL"() -> (w778:i32)
                              n599 = local read "MOS"() -> (w777:T27)
                              n600 = Index Array(array=w777, index=w778) -> (element=w776:T37)
                              n601 = Unbundle By Name(w776) -> ("Lupu's numerical value"=w775:dbl)
                              n602 = Increment(x=w783) -> (x+1=w782:i32)
                              n603 = local read "Control"() -> (w779:T3)
                              n604 = Bundle By Name(cluster=w779, "FreqLO"=w775) -> (w780:T3)
                              n605 = local write "Control"(w780) -> ()
                            }
                            frame 125 {
                              # "LO@PAMP"
                              n606 = local read "Bias_LO_equip"() -> (w791:T2)
                              n607 = Scan From String(format string="%f,%f", input string=w794) -> (output 1=w786:dbl, output 2=w785:dbl)  [unwired: 4 in, 3 out]
                              n608 = Unbundle By Name(w791) -> ("LOModule"=w790:u16, "POL"=w789:u32)
                              n609 = Increment(x=w798) -> (x+1=w797:i32)
                              n610 = case shown="0, 1, 4, 5, 기본" w790 {
                                tunnel: w789 -> [_ w800]
                                tunnel: [2 w800] -> w787
                                frame 0, 1, 4, 5, Default {
                                }
                                frame 2 {
                                }
                              }
                              n611 = local read "PA V"() -> (w792:cluster{"VD":dbl, "VG ":dbl, "String":string}[])
                              n612 = Index Array(array=w792, index=w787) -> (element=w788:cluster{"VD":dbl, "VG ":dbl, "String":string})
                              n613 = Bundle By Name(cluster=w788, "VD"=w786, "VG"=w785) -> (w793:cluster{"VD":dbl, "VG ":dbl, "String":string})
                              n614 = Replace Array Subset(array=w792, new element=w793, index=w787) -> (w784:cluster{"VD":dbl, "VG ":dbl, "String":string}[])
                              n615 = local write "PA V"(w784) -> ()
                              n616 = call "_LO_PAMP_set.vi"("PAV”z—ñ"=w784, "Bias_LO_equip"=w791) -> ()  [unwired: 10 in]
                            }
                            frame 127 {
                              # "LO@GunnSet"
                              n617 = local read "Bias_LO_equip"() -> (w809:T2)
                              n618 = local read "MOSL"() -> (w804:i32)
                              n619 = local read "MOS"() -> (w803:T27)
                              n620 = local read "LO_misc"() -> (w807:T11)
                              n621 = Index Array(array=w803, index=w804) -> (element=w802:T37)
                              n622 = Scan From String(format string="%d,%f", input string=w813) -> (output 1=w812:i32, output 2=w806:dbl)  [unwired: 4 in, 3 out]
                              n623 = Unbundle By Name(w802) -> ("Lupu's numerical value"=w801:dbl)
                              n624 = Bundle By Name(cluster=w807, "LO FRQ(GHz)"=w801) -> (w805:T11)
                              n625 = Increment(x=w817) -> (x+1=w816:i32)
                              n626 = call "_Set_LO_frq_B10_WCA.vi"("Bias_LO_equip"=w809, "LO_misc"=w805) -> ("Bias_LO_equip 2"=w808:T35)  [unwired: 15 in, 2 out]
                              n627 = local read "Control"() -> (w810:T3)
                              n628 = call "_LO_GUNN_SET.vi"("ATT"=w806, "LO_ATT"=w812, "Set@\nGunn Freq"=w801, "Bias_LO_equip"=w808) -> ()  [unwired: 8 in]
                              n629 = Bundle By Name(cluster=w810, "FreqLO"=w801) -> (w811:T3)
                              n630 = local write "Control"(w811) -> ()
                            }
                            frame 130 {
                              # "Mortor Reset"
                              n631 = local read "Control"() -> (w824:T3)
                              n632 = Unbundle By Name(w824) -> ("motor setting"=w823:T33)
                              n633 = Scan From String(format string="%d", input string=w825) -> (output 1=w822:i32)  [unwired: 3 in, 3 out]
                              n634 = Increment(x=w829) -> (x+1=w828:i32)
                              n635 = Index Array(array=w823, index=w822) -> (element=w818:T34)
                              n636 = call "__move_motor2.vi"("Moving distance"=10.0, "motor setup"=w818) -> ("counter"=w819:dbl)  [unwired: 2 in, 1 out]
                              n637 = Not Equal To 0?(x=w819) -> (x != 0?=w820:bool)
                              n638 = case shown="참" w820 {
                                tunnel: w819 -> [_ w832]
                                tunnel: w818 -> [_ w831]
                                frame False {
                                }
                                frame True {
                                n639 = Negate(x=w832) -> (-x=w830:dbl)
                                n640 = call "__move_motor2.vi"("Moving distance"=w830, "motor setup"=w831) -> ()  [unwired: 2 in, 2 out]
                                }
                              }
                            }
                            frame 135 {
                              # "Mortor Reset"
                              n641 = local read "Control"() -> (w837:T3)
                              n642 = Unbundle By Name(w837) -> ("motor setting"=w836:T33)
                              n643 = Scan From String(format string="%d,%f", input string=w838) -> (output 1=w835:i32, output 2=w833:dbl)  [unwired: 4 in, 3 out]
                              n644 = Increment(x=w842) -> (x+1=w841:i32)
                              n645 = Index Array(array=w836, index=w835) -> (element=w834:T34)
                              n646 = call "__move_motor2.vi"("Moving distance"=w833, "motor setup"=w834) -> ()  [unwired: 2 in, 2 out]
                            }
                            frame 140 {
                              # "IFBOX"
                              n647 = local read "Control"() -> (w844:T3)
                              n648 = Scan From String(format string="%d,%d,%d,%f,%d", input string=w851) -> (output 1=w850:i32, output 2=w849:i32, output 3=w848:i32, output 4=w847:dbl)  [unwired: 8 in, 3 out]
                              n649 = Unbundle By Name(w844) -> ("6501Dev#"=w843:i16)
                              n650 = Increment(x=w855) -> (x+1=w854:i32)
                              n651 = local read "IFBOX"() -> (w846:T16)
                              n652 = Bundle By Name(cluster=w846, "Input"=w850, "Output"=w849, "Filter"=w848, "YIG Fc(GHz)"=w847) -> (w845:T16)
                              n653 = call "_IFBOX_CNT.vi"("6501Dev#"=w843, "IFBOX"=w845) -> ()  [unwired: 6 in]
                              n654 = local write "IFBOX"(w845) -> ()
                            }
                            frame 145 {
                              # "IFBOX SW"
                              n655 = Scan From String(format string="%d,%d", input string=w863) -> (output 1=w860:i32, output 2=w858:i32)  [unwired: 4 in, 3 out]
                              n656 = local read "IFBOX"() -> (w859:T16)
                              n657 = Increment(x=w867) -> (x+1=w866:i32)
                              n658 = local read "Control"() -> (w856:T3)
                              n659 = case shown="6, 기본" w860 {
                                tunnel: w859 -> [w870 w873]
                                tunnel: w858 -> [w869 w872]
                                tunnel: [w868 w871] -> w857
                                frame 6, Default {
                                n660 = Bundle By Name(cluster=w870, "Output"=w869) -> (w868:T16)
                                }
                                frame 5 {
                                n661 = Bundle By Name(cluster=w873, "Input"=w872) -> (w871:T16)
                                }
                              }
                              n662 = Unbundle By Name(w856) -> ("6501Dev#"=w861:i16)
                              n663 = call "__SW_8710XB_6501.vi"("Path(1..6)"=w858, "ch(1..6)"=w860, "bit(4or6)"=4, "Dev(1,2..)"=w861) -> ()
                              n664 = local write "IFBOX"(w857) -> ()
                            }
                            frame 147 {
                              # "IFBOX BPF"
                              n665 = Scan From String(format string="%d,%f", input string=w880) -> (output 1=w876:i32, output 2=w875:dbl)  [unwired: 4 in, 3 out]
                              n666 = local read "IFBOX"() -> (w879:T16)
                              n667 = Increment(x=w884) -> (x+1=w883:i32)
                              n668 = local read "Control"() -> (w874:T3)
                              n669 = Bundle By Name(cluster=w879, "YIG Fc(GHz)"=w875) -> (w878:T16)
                              n670 = Unbundle By Name(w874) -> ("6501Dev#"=w877:i16)
                              n671 = call "__IFBOX_BPF_CONT2.vi"("YIG frq(GHz) 2"=w875, "フィルター（1:YIG,2:direct,3:4-12BPF,4:direct4-12BPF）"=w876, "Dev#"=w877) -> ()  [unwired: 1 in]
                              n672 = local write "IFBOX"(w878) -> ()
                            }
                            frame 148 {
                              # "IFBOX ATT"
                              n673 = Scan From String(format string="%d", input string=w888) -> (output 1=w886:i32)  [unwired: 3 in, 3 out]
                              n674 = local read "Control"() -> (w887:T3)
                              n675 = Increment(x=w892) -> (x+1=w891:i32)
                              n676 = Unbundle By Name(w887) -> ("GPIB_ATT"=w885:string)
                              n677 = call "__AttSet_11713A.vi"("ATT(dB)"=w886, "GPIB"=w885) -> ()  [unwired: 2 in]
                            }
                            frame 210 {
                              # "LOPopt"
                              n678 = local read "_LO_P_OPT"() -> (w902:T14)
                              n679 = local read "Bias_LO_equip"() -> (w896:T2)
                              n680 = local read "Control"() -> (w895:T3)
                              n681 = Scan From String(format string="%d,%d", input string=w905) -> (output 1=w901:i32, output 2=w900:i32)  [unwired: 4 in, 3 out]
                              n682 = Increment(x=w909) -> (x+1=w908:i32)
                              n683 = call "__file_name.vi"("Ží—Þ"=0, "Control"=w895, "Bias_LO_equip"=w896) -> ("file_name"=w894:string)  [unwired: 8 in]
                              n684 = local read "Bias_LO_equip"() -> (w903:T2)
                              n685 = local read "Control"() -> (w904:T3)
                              n686 = Bundle By Name(cluster=w902, "Optimize"=w901, "measure"=w900, "file_name"=w894, "Save?"=TRUE) -> (w898:T14)
                              n687 = call "_LO_P_OPT2.vi"("_LO_P_OPT"=w898, "Control"=w904, "Bias_LO_equip"=w903) -> ("Œ‹‰Ê"=w897:string)  [unwired: 4 in]
                              n688 = local write "Buffer"(w897) -> ()
                            }
                            frame 215 {
                              # "LOSweep"
                              n689 = Scan From String(format string="%f,%f,%f,%d", input string=w924) -> (output 1=w918:dbl, output 2=w917:dbl, output 3=w916:dbl, output 4=w910:i32)  [unwired: 6 in, 3 out]
                              n690 = local read "Bias_LO_equip"() -> (w914:T2)
                              n691 = local read "Control"() -> (w913:T3)
                              n692 = local read "Control"() -> (w923:T3)
                              n693 = Increment(x=w928) -> (x+1=w927:i32)
                              n694 = Unbundle By Name(w923) -> ("DATA path"=w915:path)
                              n695 = local read "_LO_sweep"() -> (w920:T15)
                              n696 = call "__file_name.vi"("Ží—Þ"=1, "Control"=w913, "Bias_LO_equip"=w914) -> ("file_name"=w911:string)  [unwired: 8 in]
                              n697 = local read "Bias_LO_equip"() -> (w922:T2)
                              n698 = local read "LO_misc"() -> (w921:T11)
                              n699 = Bundle By Name(cluster=w920, "file_name"=w911, "path"=w915, "start (GHz)"=w918, "stop (GHz)"=w917, "step (GHz)"=w916, "WCA Pol"=w910) -> (w919:T15)
                              n700 = call "_LO_freq_Sweep.vi"("_LO_sweep"=w919, "LO_misc"=w921, "Bias_LO_equip"=w922) -> ()  [unwired: 9 in]
                            }
                            frame 220 {
                              # "I-V"
                              n701 = local read "Bias_LO_equip"() -> (w932:T2)
                              n702 = local read "Control"() -> (w931:T3)
                              n703 = local read "i-v parameter"() -> (w952:T17)
                              n704 = Scan From String(format string="%d,%f,%d,%d,%f,%f,%f", input string=w953) -> (output 1=w949:i32, output 2=w947:dbl, output 3=w946:i32, output 4=w936:i32, output 5=w945:dbl, output 6=w944:dbl, output 7=w943:dbl)  [unwired: 9 in, 3 out]
                              n705 = call "__file_name.vi"("Ží—Þ"=2, "Control"=w931, "Bias_LO_equip"=w932) -> ("file_name"=w929:string)  [unwired: 8 in]
                              n706 = Rotate Right With Carry(2:w949, 3:TRUE) -> (1:w948:bool)  [unwired: 1 out]
                              n707 = Increment(x=w957) -> (x+1=w956:i32)
                              n708 = Bundle By Name(cluster=w952, "IF OFF/ON"=w948, "frq(GHz)"=w947, "avg"=w946, "start(mV)"=w945, "stop(mV)"=w944, "step(mV)"=w943, "file_name"=w929, "SAVE OFF/ON"=TRUE, "number of Sweep"=0) -> (w940:T17)
                              n709 = local read "SISSetVolt"() -> (w934:dbl)
                              n710 = local read "Offset"() -> (w933:dbl)
                              n711 = local read "Bias_LO_equip"() -> (w941:T2)
                              n712 = local read "Control"() -> (w937:T3)
                              n713 = Bundle By Name(cluster=w937, "control"=w936, "Set_SIS_volt"=w934, "Offset"=w933) -> (w935:T3)
                              n714 = call "_get_iv_sweep3.vi"("I-V class"=w940, "Control"=w935, "Bias_LO_equip"=w941) -> ("VP class"=w938:cluster{"array":dbl[], "array2":dbl[]}, "VI class"=w939:cluster{"array":dbl[], "array2":dbl[]})  [unwired: 2 in, 1 out]
                              n715 = local write "VP Class"(w938) -> ()
                              n716 = local write "VI Class"(w939) -> ()
                              n717 = local write "Control"(w935) -> ()
                            }
                            frame 221 {
                              # "LOなしI-V"
                              n718 = local read "Bias_LO_equip"() -> (w962:T2)
                              n719 = local read "Control"() -> (w961:T3)
                              n720 = local read "i-v parameter"() -> (w982:T17)
                              n721 = Scan From String(format string="%d,%f,%d,%d,%f,%f,%f,%s", input string=w983) -> (output 1=w979:i32, output 2=w977:dbl, output 3=w976:i32, output 4=w966:i32, output 5=w975:dbl, output 6=w974:dbl, output 7=w973:dbl, output 8=w958:string)  [unwired: 10 in, 3 out]
                              n722 = call "__file_name.vi"("comment2"=w958, "Ží—Þ"=3, "Control"=w961, "Bias_LO_equip"=w962) -> ("file_name"=w959:string)  [unwired: 7 in]
                              n723 = Rotate Right With Carry(2:w979, 3:TRUE) -> (1:w978:bool)  [unwired: 1 out]
                              n724 = Increment(x=w987) -> (x+1=w986:i32)
                              n725 = Bundle By Name(cluster=w982, "IF OFF/ON"=w978, "frq(GHz)"=w977, "avg"=w976, "start(mV)"=w975, "stop(mV)"=w974, "step(mV)"=w973, "file_name"=w959, "SAVE OFF/ON"=TRUE, "number of Sweep"=0) -> (w970:T17)
                              n726 = local read "SISSetVolt"() -> (w964:dbl)
                              n727 = local read "Offset"() -> (w963:dbl)
                              n728 = local read "Bias_LO_equip"() -> (w971:T2)
                              n729 = local read "Control"() -> (w967:T3)
                              n730 = Bundle By Name(cluster=w967, "control"=w966, "Set_SIS_volt"=w964, "Offset"=w963) -> (w965:T3)
                              n731 = call "_get_iv_sweep3.vi"("I-V class"=w970, "Control"=w965, "Bias_LO_equip"=w971) -> ("VP class"=w968:cluster{"array":dbl[], "array2":dbl[]}, "VI class"=w969:cluster{"array":dbl[], "array2":dbl[]})  [unwired: 2 in, 1 out]
                              n732 = local write "VP Class"(w968) -> ()
                              n733 = local write "VI Class"(w969) -> ()
                              n734 = local write "Control"(w965) -> ()
                            }
                            frame 225 {
                              # "I-V Trx"
                              n735 = local read "i-v parameter"() -> (w1015:T17)
                              n736 = local read "Bias_LO_equip"() -> (w992:T2)
                              n737 = local read "Control"() -> (w991:T3)
                              n738 = Scan From String(format string="%d,%f,%d,%d,%f,%f,%f,%s", input string=w1016) -> (output 1=w1012:i32, output 2=w1010:dbl, output 3=w1009:i32, output 4=w999:i32, output 5=w1008:dbl, output 6=w1007:dbl, output 7=w1006:dbl, output 8=w990:string)  [unwired: 10 in, 3 out]
                              n739 = Rotate Right With Carry(2:w1012, 3:TRUE) -> (1:w1011:bool)  [unwired: 1 out]
                              n740 = Increment(x=w1020) -> (x+1=w1019:i32)
                              n741 = call "__file_name.vi"("comment2"=w990, "Ží—Þ"=4, "Control"=w991, "Bias_LO_equip"=w992) -> ("file_name"=w988:string)  [unwired: 7 in]
                              n742 = Bundle By Name(cluster=w1015, "IF OFF/ON"=w1011, "frq(GHz)"=w1010, "avg"=w1009, "start(mV)"=w1008, "stop(mV)"=w1007, "step(mV)"=w1006, "file_name"=w988, "SAVE OFF/ON"=TRUE, "number of Sweep"=1) -> (w1003:T17)
                              n743 = local read "Volt(mV)"() -> (w995:dbl)
                              n744 = local read "Bias_LO_equip"() -> (w1004:T2)
                              n745 = local read "Offset"() -> (w994:dbl)
                              n746 = local read "Control"() -> (w1000:T3)
                              n747 = Bundle By Name(cluster=w1000, "control"=w999, "Set_SIS_volt"=w995, "Offset"=w994) -> (w998:T3)
                              n748 = call "_iv_AUTO3.vi"("i-v class"=w1003, "Control"=w998, "Bias_LO_equip"=w1004) -> ("Output string"=w993:string, "Set_SIS_volt"=w997:dbl, "XY graph 3"=w1002:cluster{dbl[], dbl[]}, "XY graph 2"=w1001:cluster{dbl[], dbl[]})  [unwired: 1 in]
                              n749 = Bundle By Name(cluster=w998, "Set_SIS_volt"=w997) -> (w996:T3)
                              n750 = local write "VP Class"(w1002) -> ()
                              n751 = local write "VI Class"(w1001) -> ()
                              n752 = local write "Buffer"(w993) -> ()
                              n753 = local write "Control"(w996) -> ()
                            }
                            frame 226 {
                              # "I-V Trx2"
                              n754 = local read "i-v parameter"() -> (w1050:T17)
                              n755 = local read "Bias_LO_equip"() -> (w1024:T2)
                              n756 = local read "Control"() -> (w1028:T3)
                              n757 = Scan From String(format string="%d,%f,%d,%d,%f,%f,%f,%d,%d,%d,%s", input string=w1051) -> (output 1=w1047:i32, output 2=w1045:dbl, output 3=w1044:i32, output 4=w1035:i32, output 5=w1043:dbl, output 6=w1042:dbl, output 7=w1041:dbl, output 8=w1023:i32, output 9=w1022:i32, output 10=w1021:i32, output 11=w1025:string)  [unwired: 13 in, 3 out]
                              n758 = Rotate Right With Carry(2:w1047, 3:TRUE) -> (1:w1046:bool)  [unwired: 1 out]
                              n759 = Increment(x=w1055) -> (x+1=w1054:i32)
                              n760 = call "__file_name.vi"("comment2"=w1025, "Ží—Þ"=4, "Control"=w1028, "Bias_LO_equip"=w1024) -> ("file_name"=w1026:string)  [unwired: 7 in]
                              n761 = Bundle By Name(cluster=w1050, "IF OFF/ON"=w1046, "frq(GHz)"=w1045, "avg"=w1044, "start(mV)"=w1043, "stop(mV)"=w1042, "step(mV)"=w1041, "file_name"=w1026, "SAVE OFF/ON"=TRUE, "number of Sweep"=w1023, "V@opt"=w1022, "mode"=w1021) -> (w1039:T17)
                              n762 = local read "Volt(mV)"() -> (w1031:dbl)
                              n763 = local read "Bias_LO_equip"() -> (w1040:T2)
                              n764 = local read "Offset"() -> (w1030:dbl)
                              n765 = local read "Control"() -> (w1036:T3)
                              n766 = Bundle By Name(cluster=w1036, "control"=w1035, "Set_SIS_volt"=w1031, "Offset"=w1030) -> (w1034:T3)
                              n767 = call "_iv_AUTO3.vi"("i-v class"=w1039, "Control"=w1034, "Bias_LO_equip"=w1040) -> ("Output string"=w1029:string, "Set_SIS_volt"=w1033:dbl, "XY graph 3"=w1038:cluster{dbl[], dbl[]}, "XY graph 2"=w1037:cluster{dbl[], dbl[]})  [unwired: 1 in]
                              n768 = Bundle By Name(cluster=w1034, "Set_SIS_volt"=w1033) -> (w1032:T3)
                              n769 = local write "VP Class"(w1038) -> ()
                              n770 = local write "VI Class"(w1037) -> ()
                              n771 = local write "Buffer"(w1029) -> ()
                              n772 = local write "Control"(w1032) -> ()
                            }
                            frame 230 {
                              # "SP"
                              n773 = local read "spectrum_data"() -> (w1076:T22)
                              n774 = local read "Bias_LO_equip"() -> (w1066:T2)
                              n775 = local read "Control"() -> (w1065:T3)
                              n776 = Scan From String(format string="%f,%f,%f,%f,%d,%f,%f,%d,%d,%s", input string=w1077) -> (output 1=w1073:dbl, output 2=w1072:dbl, output 3=w1071:dbl, output 4=w1061:dbl, output 5=w1060:i32, output 6=w1059:dbl, output 7=w1058:dbl, output 8=w1057:i32, output 9=w1056:i32, output 10=w1062:string)  [unwired: 12 in, 3 out]
                              n777 = Rotate Right With Carry(2:w1057, 3:TRUE) -> (1:w1074:bool)  [unwired: 1 out]
                              n778 = Increment(x=w1081) -> (x+1=w1080:i32)
                              n779 = call "__file_name.vi"("comment2"=w1062, "Ží—Þ"=5, "Control"=w1065, "Bias_LO_equip"=w1066) -> ("file_name"=w1063:string)  [unwired: 7 in]
                              n780 = Bundle By Name(cluster=w1076, "SP_set.start(GHz)"=w1073, "SP_set.stop(GHz)"=w1072, "SP_set.BW(MHz)"=w1071, "SP_set.VBW(Hz)"=w1061, "SP_set.point"=w1060, "SP_set.ref(dBm)"=w1059, "SP_set.log(dB)"=w1058, "ATTcal"=w1074, "HOT/COLD"=w1056, "file_name"=w1063, "SAVE OFF/ON"=TRUE) -> (w1067:T22)
                              n781 = local read "Bias_LO_equip"() -> (w1068:T2)
                              n782 = local read "Control"() -> (w1069:T3)
                              n783 = call "_sp3.vi"("sp_data"=w1067, "Control"=w1069, "Bias_LO_equip"=w1068) -> ()  [unwired: 5 in]
                            }
                            frame 240 {
                              # "YIG"
                              n784 = local read "Noise_YIG_tune_filter_control"() -> (w1095:T23)
                              n785 = local read "Bias_LO_equip"() -> (w1086:T2)
                              n786 = local read "Control"() -> (w1085:T3)
                              n787 = Scan From String(format string="%f,%f,%f,%d,%s", input string=w1096) -> (output 1=w1094:dbl, output 2=w1093:dbl, output 3=w1092:dbl, output 4=w1091:i32, output 5=w1083:string)  [unwired: 7 in, 3 out]
                              n788 = Increment(x=w1100) -> (x+1=w1099:i32)
                              n789 = call "__file_name.vi"("comment2"=w1083, "Ží—Þ"=6, "Control"=w1085, "Bias_LO_equip"=w1086) -> ("file_name"=w1082:string)  [unwired: 7 in]
                              n790 = local read "Control"() -> (w1089:T3)
                              n791 = Bundle By Name(cluster=w1095, "Start(GHz)"=w1094, "Stop(GHz)"=w1093, "Step(GHz)"=w1092, "Hot/Cold Switch"=w1091, "file_name"=w1082, "save"=TRUE) -> (w1088:T23)
                              n792 = local read "Bias_LO_equip"() -> (w1087:T2)
                              n793 = call "_Noise_YIG3.vi"("Noise_YIG"=w1088, "Bias_LO_equip"=w1087, "Control"=w1089) -> ()  [unwired: 5 in]
                            }
                            frame 250 {
                              w1108 = TRUE
                              # "SBR"
                              n794 = local read "SBR_Set"() -> (w1117:T25)
                              n795 = Scan From String(format string="%f,%f,%f,%d,%d,%d", input string=w1119) -> (output 1=w1116:dbl, output 2=w1115:dbl, output 3=w1114:dbl, output 4=w1106:i32, output 5=w1112:i32, output 6=w1109:i32)  [unwired: 8 in, 3 out]
                              n796 = Number To Decimal String(number=w1106) -> (decimal integer string=w1102:string)  [unwired: 1 in]
                              n797 = local read "Bias_LO_equip"() -> (w1105:T2)
                              n798 = local read "Control"() -> (w1104:T3)
                              n799 = Increment(x=w1123) -> (x+1=w1122:i32)
                              n800 = Rotate Right With Carry(2:w1112, 3:w1108) -> (1:w1111:bool)  [unwired: 1 out]
                              n801 = Rotate Right With Carry(2:w1109, 3:w1108) -> (1:w1110:bool)  [unwired: 1 out]
                              n802 = Rotate Right With Carry(2:w1106, 3:w1108) -> (1:w1113:bool)  [unwired: 1 out]
                              n803 = call "__file_name.vi"("comment2"=w1102, "Ží—Þ"=7, "Control"=w1104, "Bias_LO_equip"=w1105) -> ("file_name"=w1101:string)  [unwired: 7 in]
                              n804 = Bundle By Name(cluster=w1117, "start(GHz)"=w1116, "stop(GHz)"=w1115, "Step(GHz)"=w1114, "PM        SP"=w1113, "P/V         V/P"=w1111, "MPI SSB Set"=w1110, "file_name"=w1101, "save"=TRUE) -> (w1107:T25)
                              n805 = stacked-sequence {
                                seq-local: [w1124 _] -> [_ w1135]
                                tunnel: w1107 -> [w1125 _]
                                frame #0 {
                                n806 = local read "Control"() -> (w1127:T3)
                                n807 = Unbundle By Name(w1127) -> ("HOT/COLD"=w1126:u16)
                                n808 = case shown="1" w1126 {
                                tunnel: w1125 -> [w1128 w1130]
                                tunnel: [w1128 w1129] -> w1124
                                frame 0, Default {
                                }
                                frame 1 {
                                n809 = local read "Bias_LO_equip"() -> (w1134:T2)
                                n810 = Unbundle By Name(w1134) -> ("POL"=w1132:u32)
                                n811 = Rotate Right With Carry(2:w1132, 3:TRUE) -> (1:w1131:bool)  [unwired: 1 out]
                                n812 = Bundle By Name(cluster=w1130, "P/V         V/P"=w1131) -> (w1129:T25)
                                }
                                }
                                }
                                frame #1 {
                                n813 = Unbundle By Name(w1135) -> ("PM        SP"=w1137:bool)
                                n814 = local read "Control"() -> (w1136:T3)
                                n815 = case shown="거짓" w1137 {
                                tunnel: w1136 -> [w1139 w1141]
                                tunnel: w1135 -> [w1138 w1140]
                                frame False {
                                n816 = call "_SBR_mes_PM.vi"("SBR_Set"=w1138, "Control"=w1139) -> ()  [unwired: 6 in]
                                }
                                frame True {
                                n817 = call "_SBR_mes_sp.vi"("SBR_Set"=w1140, "Control"=w1141) -> ()  [unwired: 6 in]
                                }
                                }
                                }
                              }
                            }
                            frame 260 {
                              # "Allan"
                              n818 = Scan From String(format string="%f,%d,%f,%s", input string=w1154) -> (output 1=w1150:dbl, output 2=w1149:i32, output 3=w1148:dbl, output 4=w1142:string)  [unwired: 6 in, 3 out]
                              n819 = local read "Bias_LO_equip"() -> (w1146:T2)
                              n820 = local read "Control"() -> (w1145:T3)
                              n821 = local read "allan"() -> (w1153:T20)
                              n822 = local read "Control"() -> (w1152:T3)
                              n823 = Increment(x=w1158) -> (x+1=w1157:i32)
                              n824 = Unbundle By Name(w1152) -> ("DATA path"=w1151:path)
                              n825 = call "__file_name.vi"("comment2"=w1142, "Ží—Þ"=8, "Control"=w1145, "Bias_LO_equip"=w1146) -> ("file_name"=w1143:string)  [unwired: 7 in]
                              n826 = Bundle By Name(cluster=w1153, "DMM Setting A.interval"=w1150, "DMM Setting A.sample number"=w1149, "time interval"=w1148, "Path"=w1151, "File name"=w1143) -> (w1147:T20)
                              n827 = call "_allan_Variance_Ver6.vi"("allanÝèA"=w1147) -> ()  [unwired: 7 in]
                            }
                            frame 270 {
                              # "GainComp"
                              n828 = local read "GC_LockinAmp"() -> (w1169:T19)
                              n829 = local read "Bias_LO_equip"() -> (w1162:T2)
                              n830 = local read "Control"() -> (w1161:T3)
                              n831 = Increment(x=w1172) -> (x+1=w1171:i32)
                              n832 = call "__file_name.vi"("comment2"=w1163, "Ží—Þ"=9, "Control"=w1161, "Bias_LO_equip"=w1162) -> ("file_name"=w1159:string)  [unwired: 7 in]
                              n833 = Bundle By Name(cluster=w1169, "file_name"=w1159, "save"=TRUE) -> (w1165:T19)
                              n834 = local read "Bias_LO_equip"() -> (w1168:T2)
                              n835 = local read "Control"() -> (w1167:T3)
                              n836 = call "_GainComp_LockInAmp_2.vi"("GC_LockinAmp"=w1165, "Control"=w1167, "Bias_LO_equip"=w1168) -> ("oÍ¶ñ"=w1164:string)  [unwired: 8 in]
                              n837 = local write "Buffer"(w1164) -> ()
                            }
                            frame 275 {
                              # "CrossTalk"
                              n838 = local read "CrossTalk_mkpk"() -> (w1178:T18)
                              n839 = local read "Bias_LO_equip"() -> (w1182:T2)
                              n840 = local read "Control"() -> (w1181:T3)
                              n841 = Increment(x=w1187) -> (x+1=w1186:i32)
                              n842 = call "__file_name.vi"("comment2"=w1183, "Ží—Þ"=10, "Control"=w1181, "Bias_LO_equip"=w1182) -> ("file_name"=w1179:string)  [unwired: 7 in]
                              n843 = Bundle By Name(cluster=w1178, "file_name"=w1179, "save"=TRUE) -> (w1175:T18)
                              n844 = local read "Bias_LO_equip"() -> (w1177:T2)
                              n845 = local read "Control"() -> (w1176:T3)
                              n846 = local read "PA V"() -> (w1173:cluster{"VD":dbl, "VG ":dbl, "String":string}[])
                              n847 = local read "_LO_P_OPT"() -> (w1174:T14)
                              n848 = call "_crosstalk_mkpk.vi"("Bias_LO_equip"=w1177, "Control"=w1176, "CrossTalk_mkpk"=w1175, "PAV”z—ñ"=w1173, "_LO_P_OPT"=w1174) -> ()  [unwired: 5 in, 1 out]
                            }
                            frame 278 {
                              # "Harmonics"
                              n849 = local read "Bias_LO_equip"() -> (w1205:T2)
                              n850 = local read "LO harmonic"() -> (w1201:T21)
                              n851 = local read "Control"() -> (w1204:T3)
                              n852 = Scan From String(format string="%f,%f,%d", input string=w1196) -> (output 1=w1193:dbl, output 2=w1192:dbl, output 3=w1194:i32)  [unwired: 5 in, 3 out]
                              n853 = Increment(x=w1209) -> (x+1=w1208:i32)
                              n854 = Rotate Right With Carry(2:w1194, 3:TRUE) -> (1:w1191:bool)  [unwired: 1 out]
                              n855 = case shown="거짓" w1191 {
                                tunnel: ["8th" "10th"] -> w1190
                                frame False {
                                }
                                frame True {
                                }
                              }
                              n856 = call "__file_name.vi"("comment2"=w1190, "Ží—Þ"=11, "Control"=w1204, "Bias_LO_equip"=w1205) -> ("file_name"=w1202:string)  [unwired: 7 in]
                              n857 = Bundle By Name(cluster=w1201, "LO start"=w1193, "LO stop"=w1192, "8th 10th"=w1191, "file_name"=w1202, "save"=TRUE) -> (w1198:T21)
                              n858 = local read "Bias_LO_equip"() -> (w1200:T2)
                              n859 = local read "Control"() -> (w1199:T3)
                              n860 = local read "PA V"() -> (w1189:cluster{"VD":dbl, "VG ":dbl, "String":string}[])
                              n861 = local read "_LO_P_OPT"() -> (w1188:T14)
                              n862 = call "_LOharmonic.vi"("Bias_LO_equip"=w1200, "Control"=w1199, "LOhharmonic"=w1198, "PAV”z—ñ"=w1189, "_LO_P_OPT"=w1188) -> ()  [unwired: 5 in, 1 out]
                            }
                            frame 281 {
                              # "TempPM"
                              n863 = Scan From String(format string="%d", input string=w1216) -> (output 1=w1214:i32)  [unwired: 3 in, 3 out]
                              n864 = local read "Bias_LO_equip"() -> (w1212:T2)
                              n865 = local read "Control"() -> (w1215:T3)
                              n866 = Increment(x=w1220) -> (x+1=w1219:i32)
                              n867 = call "_HC_PM_and_temp.vi"("PMavg"=w1214, "Bias_LO_equip"=w1212, "Control"=w1215) -> ("•¶Žš—ñ"=w1213:string)  [unwired: 8 in]
                              n868 = local write "Buffer"(w1213) -> ()
                            }
                            frame 282 {
                              # "Read WCA temp"
                              n869 = flat-sequence {
                                tunnel: w1235 -> [w1243]
                                tunnel: [w1242] -> w1227
                                tunnel: [w1241] -> w1226
                                tunnel: [w1240] -> w1225
                                tunnel: w1232 -> [w1248]
                                tunnel: [w1247] -> w1224
                                tunnel: [w1246] -> w1223
                                tunnel: [w1245] -> w1222
                                frame #0 {
                                n870 = call "__Temp_Get.vi"("Bias_LO_equip"=w1243) -> ("MixTemp"=w1240:dbl, "90/20K_temp"=w1241:dbl, "4K_Temp"=w1242:dbl)  [unwired: 8 in]
                                }
                                frame #1 {
                                n871 = Wait (ms)(milliseconds to wait=100) -> ()  [unwired: 1 out]
                                }
                                frame #2 {
                                n872 = call "__Temp_Get.vi"("Bias_LO_equip"=w1248) -> ("MixTemp"=w1245:dbl, "90/20K_temp"=w1246:dbl, "4K_Temp"=w1247:dbl)  [unwired: 8 in]
                                }
                              }
                              n873 = local read "Bias_LO_equip"() -> (w1233:T2)
                              n874 = Increment(x=w1239) -> (x+1=w1238:i32)
                              n875 = Bundle By Name(cluster=w1233, "POL"=0) -> (w1235:T2)
                              n876 = Get Date/Time In Seconds() -> (seconds since 1Jan1904=w1229:timestamp)
                              n877 = Bundle By Name(cluster=w1233, "POL"=1) -> (w1232:T2)
                              n878 = Format Date/Time String(time format string (%c)="%Y-%m-%d  %H:%M:%S", seconds (now)=w1229) -> (date/time string=w1230:string)  [unwired: 1 in]
                              n879 = Format Into String(format string="WCA-Temp, %s,%.2f ,%.2f ,%.2f ,%.2f ,%.2f ,%.2f ", w1230, w1227, w1226, w1225, w1224, w1223, w1222) -> (resulting string=w1221:string)  [unwired: 2 in, 1 out]
                              n880 = local write "Buffer"(w1221) -> ()
                            }
                            frame 283 {
                              # "BiasHelthChech"
                              n881 = local read "Bias_LO_equip"() -> (w1249:T2)
                              n882 = Increment(x=w1253) -> (x+1=w1252:i32)
                              n883 = call "_Bias_health_check.vi"("Bias_LO_equip"=w1249) -> ("•¶Žš—ñ"=w1250:string)  [unwired: 10 in]
                              n884 = local write "Buffer"(w1250) -> ()
                            }
                            frame 284 {
                              # "CAN node"
                              n885 = local read "Bias_LO_equip"() -> (w1266:T2)
                              n886 = local read "Control"() -> (w1267:T3)
                              n887 = Unbundle By Name(w1267) -> ("Th"=w1264:dbl, "Tc"=w1263:dbl, "DATA path"=w1262:path, "mixer param file"=w1260:path, "HOT/COLD"=w1259:u16, "MPI offset(mm)"=w1258:dbl)
                              n888 = Unbundle By Name(w1266) -> ("WCA_LO_FREQ_SET.YTO Low freq. [GHz]"=w1257:sgl, "WCA_LO_FREQ_SET.YTO High freq. [GHz]"=w1256:sgl)
                              n889 = local read "Detected CAN Nodes."() -> (w1255:string)
                              n890 = Increment(x=w1270) -> (x+1=w1269:i32)
                              n891 = local read "file name"() -> (w1254:string)
                              n892 = Format Into String(format string="Control\nTh, %f\nTc, %f\nDataパス, %s\nmixparam, %s\nHOT/COLD,%d\nMPIoffset,%f\n\nBias_Lo_equip\nWCA LO YTO Low, %f\nWCA LO YTO High %f\n \nCAN node\n%s\n\nscript file\n%s", w1264, w1263, w1262, w1260, w1259, w1258, w1257, w1256, w1255, w1254) -> (resulting string=w1261:string)  [unwired: 2 in, 1 out]
                              n893 = local write "Buffer"(w1261) -> ()
                            }
                            frame 290 {
                              # "shapiro"
                              n894 = local read "shapiro"() -> (w1283:T9)
                              n895 = local read "Bias_LO_equip"() -> (w1286:T2)
                              n896 = local read "Control"() -> (w1282:T3)
                              n897 = Scan From String(format string="%f,%f,%f", input string=w1279) -> (output 1=w1278:dbl, output 2=w1277:dbl, output 3=w1276:dbl)  [unwired: 5 in, 3 out]
                              n898 = Increment(x=w1290) -> (x+1=w1289:i32)
                              n899 = call "__file_name.vi"("Ží—Þ"=18, "Control"=w1282, "Bias_LO_equip"=w1286) -> ("file_name"=w1284:string)  [unwired: 8 in]
                              n900 = Unbundle By Name(w1282) -> ("DATA path"=w1281:path)
                              n901 = Bundle By Name(cluster=w1283, "path"=w1281, "file_name"=w1284, "save?"=TRUE, "start(mA)"=w1278, "stop(mA)"=w1277, "step(mA)"=w1276) -> (w1275:T9)
                              n902 = local read "Bias_LO_equip"() -> (w1274:T2)
                              n903 = local read "demag"() -> (w1272:T7)
                              n904 = local read "Control"() -> (w1273:T3)
                              n905 = call "_shapiro2.vi"("Bias_LO_equip"=w1274, "Control"=w1273, "shapiro"=w1275, "demag"=w1272) -> ("min Mag current"=w1271:dbl)  [unwired: 6 in]
                              n906 = local write "Magnet Current Set"(w1271) -> ()
                            }
                            frame 292 {
                              # "Demag"
                              n907 = Scan From String(format string="%f,%f,%f", input string=w1297) -> (output 1=w1295:dbl, output 2=w1294:dbl, output 3=w1293:dbl)  [unwired: 5 in, 3 out]
                              n908 = Increment(x=w1301) -> (x+1=w1300:i32)
                              n909 = local read "demag"() -> (w1296:T7)
                              n910 = Bundle By Name(cluster=w1296, "Start(mA)"=w1295, "step"=w1294, "Time(ms)"=w1293) -> (w1292:T7)
                              n911 = local read "Bias_LO_equip"() -> (w1291:T2)
                              n912 = call "_Demagnetization.vi"("demag"=w1292, "Bias_LO_equip"=w1291) -> ()  [unwired: 10 in]
                            }
                            frame 293 {
                              # "DefluxHTR"
                              n913 = local read "Bias_LO_equip"() -> (w1309:T2)
                              n914 = local read "Control"() -> (w1306:T3)
                              n915 = Increment(x=w1313) -> (x+1=w1312:i32)
                              n916 = local read "SIS_Deflux_heater"() -> (w1304:T10)
                              n917 = call "__file_name.vi"("Ží—Þ"=20, "Control"=w1306, "Bias_LO_equip"=w1309) -> ("file_name"=w1307:string)  [unwired: 8 in]
                              n918 = Unbundle By Name(w1306) -> ("DATA path"=w1305:path)
                              n919 = Bundle By Name(cluster=w1304, "path"=w1305, "file_name"=w1307, "SAVE"=TRUE) -> (w1302:T10)
                              n920 = local read "Bias_LO_equip"() -> (w1310:T2)
                              n921 = call "_SIS_defux_heater.vi"("SIS_Deflux_heater"=w1302, "Bias_LO_equip"=w1310) -> ()  [unwired: 10 in]
                            }
                            frame 294 {
                              # "JC"
                              n922 = local read "Joseph_curr"() -> (w1315:T8)
                              n923 = local read "Bias_LO_equip"() -> (w1326:T2)
                              n924 = local read "Control"() -> (w1323:T3)
                              n925 = Scan From String(format string="%f,%f,%f", input string=w1320) -> (output 1=w1319:dbl, output 2=w1318:dbl, output 3=w1317:dbl)  [unwired: 5 in, 3 out]
                              n926 = Increment(x=w1330) -> (x+1=w1329:i32)
                              n927 = call "__file_name.vi"("Ží—Þ"=19, "Control"=w1323, "Bias_LO_equip"=w1326) -> ("file_name"=w1324:string)  [unwired: 8 in]
                              n928 = Unbundle By Name(w1323) -> ("DATA path"=w1322:path)
                              n929 = Bundle By Name(cluster=w1315, "file path"=w1322, "file_name"=w1324, "save?"=TRUE, "start(mA)"=w1319, "stop(mA)"=w1318, "step(mA)"=w1317) -> (w1314:T8)
                              n930 = local read "Bias_LO_equip"() -> (w1316:T2)
                              n931 = call "_Josep_curr_Imag_2.vi"("Joseph_curr"=w1314, "Bias_LO_equip"=w1316) -> ()  [unwired: 10 in]
                            }
                            frame 301 {
                              # "ReadMixerParam"
                              n932 = local read "Bias_LO_equip"() -> (w1332:T2)
                              n933 = local read "Control"() -> (w1333:T3)
                              n934 = Increment(x=w1336) -> (x+1=w1335:i32)
                              n935 = call "_read_mixer_params.vi"("Control"=w1333, "Bias_LO_equip"=w1332) -> ("•¶Žš—ñ"=w1331:string)  [unwired: 9 in]
                              n936 = local write "Buffer"(w1331) -> ()
                            }
                            frame 302 {
                              # "ReadCLNArParam"
                              n937 = local read "Bias_LO_equip"() -> (w1338:T2)
                              n938 = local read "Control"() -> (w1339:T3)
                              n939 = Increment(x=w1342) -> (x+1=w1341:i32)
                              n940 = call "_read_CLNA_params.vi"("Control"=w1339, "Bias_LO_equip"=w1338) -> ("•¶Žš—ñ"=w1337:string)  [unwired: 9 in]
                              n941 = local write "Buffer"(w1337) -> ()
                            }
                            frame 303 {
                              # "Read LO Param"
                              n942 = local read "Bias_LO_equip"() -> (w1344:T2)
                              n943 = local read "Control"() -> (w1345:T3)
                              n944 = Increment(x=w1348) -> (x+1=w1347:i32)
                              n945 = call "_read_LO_params.vi"("Control"=w1345, "Bias_LO_equip"=w1344) -> ("•¶Žš—ñ"=w1343:string)  [unwired: 9 in]
                              n946 = local write "Buffer"(w1343) -> ()
                            }
                            frame 311 {
                              # "SetMixerParam"
                              n947 = local read "Bias_LO_equip"() -> (w1358:T2)
                              n948 = local read "_LO_P_OPT"() -> (w1350:T14)
                              n949 = Bundle By Name(cluster=w1350, "SISparam option"=0) -> (w1349:T14)
                              n950 = local read "Control"() -> (w1357:T3)
                              n951 = Increment(x=w1361) -> (x+1=w1360:i32)
                              n952 = call "_set_mixer_params.vi"("_LO_P_OPT"=w1349, "Control"=w1357, "Bias_LO_equip"=w1358) -> ("•¶Žš—ñ"=w1355:string, "Control 2"=w1354:T36, "Bias_LO_equip 2"=w1356:T35)  [unwired: 6 in]
                              n953 = Unbundle By Name(w1354) -> ("Set_SIS_volt"=w1353:dbl, "Offset"=w1352:dbl)
                              n954 = local write "Bias_LO_equip"(w1356) -> ()
                              n955 = local write "Buffer"(w1355) -> ()
                              n956 = local write "Control"(w1354) -> ()
                              n957 = local write "Offset"(w1352) -> ()
                              n958 = local write "SISSetVolt"(w1353) -> ()
                            }
                            frame 314 {
                              # "SetMixerParam V"
                              n959 = local read "_LO_P_OPT"() -> (w1364:T14)
                              n960 = local read "Bias_LO_equip"() -> (w1371:T2)
                              n961 = local read "Control"() -> (w1370:T3)
                              n962 = Increment(x=w1374) -> (x+1=w1373:i32)
                              n963 = Bundle By Name(cluster=w1364, "SISparam option"=1) -> (w1362:T14)
                              n964 = call "_set_mixer_params.vi"("_LO_P_OPT"=w1362, "Control"=w1370, "Bias_LO_equip"=w1371) -> ("•¶Žš—ñ"=w1368:string, "Control 2"=w1367:T36, "Bias_LO_equip 2"=w1369:T35)  [unwired: 6 in]
                              n965 = Unbundle By Name(w1367) -> ("Set_SIS_volt"=w1366:dbl, "Offset"=w1365:dbl)
                              n966 = local write "Bias_LO_equip"(w1369) -> ()
                              n967 = local write "Buffer"(w1368) -> ()
                              n968 = local write "Control"(w1367) -> ()
                              n969 = local write "Offset"(w1365) -> ()
                              n970 = local write "SISSetVolt"(w1366) -> ()
                            }
                            frame 320 {
                              # "Select mixer param,"
                              n971 = local read "Control"() -> (w1376:T3)
                              n972 = Unbundle By Name(w1376) -> ("mixer param file"=w1375:path)
                              n973 = Increment(x=w1388) -> (x+1=w1387:i32)
                              n974 = call "ファイルダイアログ6"("start path"=w1375, "prompt"="mixer パラメータファイル", "button label"="select this file") -> ("selected path"=w1378:path, "exists"=w1383:bool, "cancelled"=w1385:bool)  [unwired: 9 in, 1 out]
                              n975 = Not(x=w1383) -> (.not. x?=w1384:bool)
                              n976 = local read "Control"() -> (w1380:T3)
                              n977 = Or(x=w1384, y=w1385) -> (x .or. y?=w1377:bool)
                              n978 = case shown="거짓" w1377 {
                                tunnel: w1380 -> [w1391 w1394]
                                tunnel: [w1390 w1395] -> w1379
                                tunnel: w1378 -> [w1389 _]
                                frame False {
                                n979 = Bundle By Name(cluster=w1391, "mixer param file"=w1389) -> (w1390:T3)
                                }
                                frame True {
                                n980 = String To Path(string="c:\\data\\") -> (path=w1392:path)
                                n981 = Bundle By Name(cluster=w1394, "DATA path"=w1392) -> (w1395:T3)
                                }
                              }
                              n982 = local write "Control"(w1379) -> ()
                            }
                            frame 401 {
                              # "Opens the template."
                              # "Open excel"
                              n983 = local read "Script path"() -> (w1400:path)
                              n984 = Build Path(base path=w1400, name or relative path=w1399) -> (appended path=w1397:path)
                              n985 = Increment(x=w1403) -> (x+1=w1402:i32)
                              n986 = call <vilib>:"New Report.vi"("report type"=T31."Excel", "template (empty)"=w1397) -> ("report out"=w1396:refnum<class "NI_report.lvclass">)  [unwired: 12 in, 1 out]
                              n987 = local write "report"(w1396) -> ()
                            }
                            frame 402 {
                              # "excel save"
                              n988 = local read "Bias_LO_equip"() -> (w1406:T2)
                              n989 = local read "Control"() -> (w1413:T3)
                              n990 = local read "Control"() -> (w1407:T3)
                              n991 = Increment(x=w1416) -> (x+1=w1415:i32)
                              n992 = local read "Buffer"() -> (w1408:string)
                              n993 = local read "Script path"() -> (w1409:path)
                              n994 = Unbundle By Name(w1413) -> ("DATA path"=w1412:path)
                              n995 = call "_srcipt_text_replace.vi"("スクリプトパス"=w1409, "バッファ"=w1408, "Bias_LO_equip"=w1406, "Control"=w1407, "input"=w1405) -> ("output"=w1404:string)  [unwired: 6 in]
                              n996 = Build Path(base path=w1412, name or relative path=w1404) -> (appended path=w1410:path)
                              n997 = local read "report"() -> (w1411:refnum<class "NI_report.lvclass">)
                              n998 = call-dynamic "Save Report to File.vi"("report in"=w1411, "report file path"=w1410) -> ()  [unwired: 12 in, 2 out]
                            }
                            frame 403 {
                              # "excel close"
                              n999 = Increment(x=w1420) -> (x+1=w1419:i32)
                              n1000 = local read "report"() -> (w1417:refnum<class "NI_report.lvclass">)
                              n1001 = call-dynamic "Dispose Report.vi"("report in"=w1417) -> ()  [unwired: 14 in, 1 out]
                            }
                            frame 404 {
                              # "open sheet"
                              n1002 = case shown="\"%NUM%\"" w1424 {
                                selector: w1424 -> [w1428 _]
                                tunnel: [w1428 w1429] -> w1423
                                frame Default {
                                }
                                frame "%NUM%" {
                                n1003 = local read "MOSL"() -> (w1434:i32)
                                n1004 = local read "MOS"() -> (w1433:T27)
                                n1005 = Index Array(array=w1433, index=w1434) -> (element=w1432:T37)
                                n1006 = Unbundle By Name(w1432) -> ("Lupu's numerical value"=w1431:dbl)
                                n1007 = Format Into String(format string="%.2f", w1431) -> (resulting string=w1429:string)  [unwired: 2 in, 1 out]
                                }
                              }
                              n1008 = Increment(x=w1427) -> (x+1=w1426:i32)
                              n1009 = local read "report"() -> (w1422:refnum<class "NI_report.lvclass">)
                              n1010 = call <vilib>:"Excel Get Worksheet.vi"("report in"=w1422, "name (\"\")"=w1423) -> ("report out"=w1421:refnum<class "NI_report.lvclass">)  [unwired: 12 in, 1 out]
                              n1011 = local write "report"(w1421) -> ()
                            }
                            frame 405 {
                              # "set cell"
                              n1012 = Scan From String(format string="%d,%d,%s", input string=w1448) -> (output 1=w1445:i32, output 2=w1444:i32, output 3=w1440:string)  [unwired: 5 in, 3 out]
                              n1013 = local read "Bias_LO_equip"() -> (w1435:T2)
                              n1014 = local read "Control"() -> (w1436:T3)
                              n1015 = local read "Buffer"() -> (w1437:string)
                              n1016 = local read "Script path"() -> (w1438:path)
                              n1017 = Increment(x=w1451) -> (x+1=w1450:i32)
                              n1018 = call "_srcipt_text_replace.vi"("スクリプトパス"=w1438, "バッファ"=w1437, "Bias_LO_equip"=w1435, "Control"=w1436, "input"=w1440) -> ("output"=w1439:string)  [unwired: 6 in]
                              n1019 = local read "report"() -> (w1442:refnum<class "NI_report.lvclass">)
                              n1020 = Bundle By Name(cluster=T32 {"position (Excel)"={"row"=0, "column"=0}, "name (Excel)"="", "bookmark (Word)"=""} ("MS Office parameters"), "position (Excel).row"=w1445, "position (Excel).column"=w1444) -> (w1443:T32)
                              n1021 = call-poly <vilib>:"Append Report Text.vi"("report in"=w1442, "MS Office parameters"=w1443, "text"=w1439) -> ("report out"=w1441:refnum<class "NI_report.lvclass">)  [unwired: 9 in, 3 out]
                              n1022 = local write "report"(w1441) -> ()
                            }
                            frame 406 {
                              # "set 2D data"
                              n1023 = local read "2D data"() -> (w1459:string[][])
                              n1024 = Scan From String(format string="%d,%d", input string=w1461) -> (output 1=w1456:i32, output 2=w1455:i32)  [unwired: 4 in, 3 out]
                              n1025 = Increment(x=w1465) -> (x+1=w1464:i32)
                              n1026 = Bundle By Name(cluster=T32 {"position (Excel)"={"row"=0, "column"=0}, "name (Excel)"="", "bookmark (Word)"=""} ("MS Office parameters"), "position (Excel).row"=w1456, "position (Excel).column"=w1455) -> (w1457:T32)
                              n1027 = local read "report"() -> (w1454:refnum<class "NI_report.lvclass">)
                              n1028 = call-poly <vilib>:"Append Table to Report.vi"("report in"=w1454, "column width (1)"=-1.0, "MS Office parameters"=w1457, "text data"=w1459, "show grid lines (YES)"=FALSE) -> ("report out"=w1453:refnum<class "NI_report.lvclass">)  [unwired: 7 in, 3 out]
                              n1029 = local write "report"(w1453) -> ()
                            }
                            frame 407 {
                              # "excel window"
                              n1030 = Increment(x=w1468) -> (x+1=w1467:i32)
                            }
                            frame 410 {
                              # "make file name"
                              n1031 = Scan From String(format string="%d,%s", input string=w1474) -> (output 1=w1471:i32, output 2=w1472:string)  [unwired: 4 in, 3 out]
                              n1032 = Greater Or Equal To 0?(x=w1471) -> (x >= 0?=w1470:bool)
                              n1033 = Increment(x=w1477) -> (x+1=w1476:i32)
                              n1034 = case shown="참" w1470 {
                                tunnel: w1471 -> [_ w1491]
                                tunnel: w1472 -> [_ w1490]
                                tunnel: [w1478 w1482] -> w1469
                                frame False {
                                n1035 = local read "Control"() -> (w1481:T3)
                                n1036 = Unbundle By Name(w1481) -> ("comment"=w1479:string)
                                n1037 = Format Into String(format string="mix_log_%s.txt", w1479) -> (resulting string=w1478:string)  [unwired: 2 in, 1 out]
                                }
                                frame True {
                                n1038 = local read "MOSL"() -> (w1487:i32)
                                n1039 = local read "MOS"() -> (w1486:T27)
                                n1040 = Index Array(array=w1486, index=w1487) -> (element=w1485:T37)
                                n1041 = Unbundle By Name(w1485) -> ("Lupu's numerical value"=w1484:dbl)
                                n1042 = local read "Control"() -> (w1488:T3)
                                n1043 = local read "Bias_LO_equip"() -> (w1489:T2)
                                n1044 = Bundle By Name(cluster=w1488, "FreqLO"=w1484) -> (w1483:T3)
                                n1045 = call "__file_name.vi"("comment2"=w1490, "Ží—Þ"=w1491, "Control"=w1483, "Bias_LO_equip"=w1489) -> ("file_name"=w1482:string)  [unwired: 7 in]
                                }
                              }
                              n1046 = local write "Buffer"(w1469) -> ()
                            }
                            frame 411 {
                              # "files Time Stamp"
                              n1047 = local read "Control"() -> (w1498:T3)
                              n1048 = local read "Buffer"() -> (w1496:string)
                              n1049 = Unbundle By Name(w1498) -> ("DATA path"=w1497:path)
                              n1050 = Increment(x=w1501) -> (x+1=w1500:i32)
                              n1051 = Build Path(base path=w1497, name or relative path=w1496) -> (appended path=w1495:path)
                              n1052 = File/Directory Info(path=w1495) -> (last mod=w1494:timestamp)  [unwired: 1 in, 6 out]
                              n1053 = Format Date/Time String(time format string (%c)="%Y-%m-%d  %H:%M:%S", seconds (now)=w1494) -> (date/time string=w1492:string)  [unwired: 1 in]
                              n1054 = local write "Buffer"(w1492) -> ()
                            }
                            frame 412 {
                              # "read 2D data"
                              n1055 = local read "Control"() -> (w1510:T3)
                              n1056 = local read "Buffer"() -> (w1508:string)
                              n1057 = Scan From String(format string="%d", input string=w1512) -> (output 1=w1506:i32)  [unwired: 3 in, 3 out]
                              n1058 = Unbundle By Name(w1510) -> ("DATA path"=w1509:path)
                              n1059 = Increment(x=w1515) -> (x+1=w1514:i32)
                              n1060 = Build Path(base path=w1509, name or relative path=w1508) -> (appended path=w1507:path)
                              n1061 = call-poly <vilib>:"Read From Spreadsheet File.vi"("delimiter (\\t)"=",", "file path (dialog if empty)"=w1507) -> ("all rows"=w1503:string[][])  [unwired: 5 in, 4 out]
                              n1062 = Delete From Array(array=w1503, length=w1506, index (row)=0) -> (array with subset deleted=w1505:string[][])  [unwired: 1 in, 1 out]
                              n1063 = local write "2D data"(w1505) -> ()
                            }
                            frame 414 {
                              # "choice 2D data"
                              n1064 = Scan From String(format string="%d,%s", input string=w1524) -> (output 1=w1521:i32, output 2=w1516:string)  [unwired: 4 in, 3 out]
                              n1065 = Increment(x=w1527) -> (x+1=w1526:i32)
                              n1066 = Equal?(x=w1516, y="%POL%") -> (x = y?=w1518:bool)
                              n1067 = case shown="참" w1518 {
                                tunnel: [w1528 w1529] -> w1517
                                tunnel: w1516 -> [w1528 _]
                                frame False {
                                }
                                frame True {
                                n1068 = local read "Bias_LO_equip"() -> (w1532:T2)
                                n1069 = Unbundle By Name(w1532) -> ("POL"=w1530:u32)
                                n1070 = Format Into String(format string="%d", w1530) -> (resulting string=w1529:string)  [unwired: 2 in, 1 out]
                                }
                              }
                              n1071 = local read "2D data"() -> (w1522:string[][])
                              n1072 = call "__para_[CABLE]n.vi"("õl"=w1517, "検索キー列"=w1521, "読み込み配列"=w1522) -> ("oÍzñ"=w1520:string[][])  [unwired: 6 in]
                              n1073 = local write "2D data"(w1520) -> ()
                            }
                            frame 450 {
                              w1541 = "YIG_%.2f_1%1d%1d_%s"
                              # "calc IF output"
                              n1074 = local read "MOSL"() -> (w1562:i32)
                              n1075 = local read "MOS"() -> (w1561:T27)
                              n1076 = Index Array(array=w1561, index=w1562) -> (element=w1560:T37)
                              n1077 = Unbundle By Name(w1560) -> ("Lupu's numerical value"=w1553:dbl)
                              n1078 = local read "Control"() -> (w1563:T3)
                              n1079 = local read "Bias_LO_equip"() -> (w1539:T2)
                              n1080 = Increment(x=w1566) -> (x+1=w1565:i32)
                              n1081 = Bundle By Name(cluster=w1563, "FreqLO"=799) -> (w1554:T3)
                              n1082 = call "__file_name.vi"("comment2"="aNS", "Ží—Þ"=6, "Control"=w1554, "Bias_LO_equip"=w1539) -> ("file_name"=w1542:string)  [unwired: 7 in]
                              n1083 = Unbundle By Name(w1539) -> ("POL"=w1536:u32)
                              n1084 = Bundle By Name(cluster=w1554, "FreqLO"=w1553) -> (w1552:T3)
                              n1085 = Unbundle By Name(w1554) -> ("Th"=w1545:dbl, "Tc"=w1544:dbl, "DATA path"=w1551:path)
                              n1086 = call "__file_name.vi"("comment2"="m", "Ží—Þ"=6, "Control"=w1552, "Bias_LO_equip"=w1539) -> ("file_name"=w1538:string)  [unwired: 7 in]
                              n1087 = Scan From String(format string=w1541, input string=w1538) -> (output 1=w1540:dbl, output 2=w1535:i32, output 4=w1534:string)  [unwired: 7 in, 3 out]
                              n1088 = Build Path(base path=w1551, name or relative path=w1542) -> (appended path=w1549:path)
                              n1089 = local read "Calc_IFout"() -> (w1550:T29)
                              n1090 = Format Into String(format string=w1541, w1540, w1535, w1536, w1534) -> (resulting string=w1537:string)  [unwired: 2 in, 1 out]
                              n1091 = Build Path(base path=w1551, name or relative path=w1537) -> (appended path=w1548:path)
                              n1092 = Bundle By Name(cluster=w1550, "Th"=w1545, "Tc"=w1544, "NS_output_data"=w1549, "Rx_output_data"=w1548, "SAVE"=TRUE) -> (w1547:T29)
                              n1093 = call "_calc_IFoutput.vi"("Calc_IFout"=w1547) -> ("oÍ¶ñ"=w1546:string, "Calc_IFout 2"=w1533:T29)  [unwired: 9 in]
                              n1094 = local write "Buffer"(w1546) -> ()
                              n1095 = local write "Calc_IFout"(w1533) -> ()
                            }
                            frame 451 {
                              # "SP@Sprious"
                              n1096 = local read "MOSL"() -> (w1582:i32)
                              n1097 = local read "MOS"() -> (w1581:T27)
                              n1098 = Index Array(array=w1581, index=w1582) -> (element=w1580:T37)
                              n1099 = Unbundle By Name(w1580) -> ("Lupu's numerical value"=w1577:dbl)
                              n1100 = local read "Control"() -> (w1569:T3)
                              n1101 = local read "Bias_LO_equip"() -> (w1573:T2)
                              n1102 = Increment(x=w1585) -> (x+1=w1584:i32)
                              n1103 = Bundle By Name(cluster=w1569, "FreqLO"=w1577) -> (w1568:T3)
                              n1104 = Unbundle By Name(w1569) -> ("DATA path"=w1576:path)
                              n1105 = call "__file_name.vi"("comment2"="FB", "Ží—Þ"=5, "Control"=w1568, "Bias_LO_equip"=w1573) -> ("file_name"=w1567:string)  [unwired: 7 in]
                              n1106 = Build Path(base path=w1576, name or relative path=w1567) -> (appended path=w1572:path)
                              n1107 = local read "SP_Spurious"() -> (w1575:cluster{"Rx_output_data":path, "SAVE":bool})
                              n1108 = Bundle By Name(cluster=w1575, "Rx_output_data"=w1572, "SAVE"=TRUE) -> (w1571:cluster{"Rx_output_data":path, "SAVE":bool})
                              n1109 = call "_sp_spurious.vi"("SP_Spurious"=w1571) -> ("oÍ¶ñ"=w1570:string)  [unwired: 10 in]
                              n1110 = local write "Buffer"(w1570) -> ()
                            }
                            frame 460 {
                              # "Make 3D graph"
                              n1111 = local read "Control"() -> (w1590:T3)
                              n1112 = local read "Buffer"() -> (w1588:string)
                              n1113 = Unbundle By Name(w1590) -> ("DATA path"=w1589:path)
                              n1114 = Scan From String(format string="%f,%f,%f,%d,%d,%d,%d,%d", input string=w1600) -> (output 1=w1598:dbl, output 2=w1597:dbl, output 3=w1596:dbl, output 4=w1595:i32, output 5=w1594:i32, output 6=w1593:i32, output 7=w1592:i32, output 8=w1591:i32)  [unwired: 10 in, 3 out]
                              n1115 = Increment(x=w1604) -> (x+1=w1603:i32)
                              n1116 = local read "mk3d"() -> (w1599:T30)
                              n1117 = Bundle By Name(cluster=w1599, "Start(GHz)"=w1598, "Stop(GHz)"=w1597, "Step(GHz)"=w1596, "Text line skip"=w1595, "Ring X"=w1594, "Ring Z"=w1593, "Acquisition column X"=w1592, "Acquisition column Z"=w1591, "path"=w1589, "first file name"=w1588) -> (w1587:T30)
                              n1118 = call "_make_3d_data2.vi"("mk3d"=w1587) -> ("出力ファイル名"=w1586:string)  [unwired: 10 in]
                              n1119 = local write "Buffer"(w1586) -> ()
                            }
                          }
                        }
                        frame #2 {
                          # "スクリプトの終了処理\nサブスクリプト実行時は元プログラムに戻す"
                          n1120 = local read "MOSL"() -> (w1607:i32)
                          n1121 = Greater Than 0?(x=w1607) -> (x > 0?=w1609:bool)
                          n1122 = local read "MOS"() -> (w1613:T27)
                          n1123 = Index Array(array=w1613, index=w1607) -> (element=w1612:T37)
                          n1124 = Unbundle By Name(w1612) -> ("number of lines"=w1611:i32)
                          n1125 = Greater Or Equal?(x=w1605, y=w1611) -> (x >= y?=w1614:bool)
                          n1126 = Or(x=w1614, y=w1615) -> (x .or. y?=w1610:bool)
                          n1127 = case shown="거짓" w1610 {
                            tunnel: w1609 -> [_ w1622]
                            tunnel: [FALSE w1621] -> w1608
                            tunnel: w1607 -> [_ w1620]
                            tunnel: [w1616 w1619] -> w1606
                            tunnel: w1605 -> [w1616 w1618]
                            frame False {
                            }
                            frame True {
                              n1128 = case shown="참" w1622 {
                                tunnel: [TRUE w1625] -> w1621
                                tunnel: w1620 -> [_ w1627]
                                tunnel: [w1623 w1626] -> w1619
                                tunnel: w1618 -> [w1623 _]
                                frame False {
                                # "MOSL=０　元のプログラム"
                                }
                                frame True {
                                n1129 = stacked-sequence {
                                tunnel: w1627 -> [w1641 _]
                                tunnel: [_ w1649] -> w1626
                                tunnel: [FALSE _] -> w1625
                                frame #0 {
                                # "親プログラムの読み込み"
                                n1130 = local read "Script path"() -> (w1640:path)
                                n1131 = Decrement(x=w1641) -> (x-1=w1639:i32)
                                n1132 = Format Into String(format string="MOS_SUB%d.tmp", w1639) -> (resulting string=w1638:string)  [unwired: 2 in, 1 out]
                                n1133 = Build Path(base path=w1640, name or relative path=w1638) -> (appended path=w1630:path)
                                n1134 = local write "MOSL"(w1639) -> ()
                                n1135 = call-poly <vilib>:"Read From Spreadsheet File.vi"("delimiter (\\t)"="@@@", "format (%s)"="%s", "file path (dialog if empty)"=w1630) -> ("all rows"=w1636:string[][])  [unwired: 4 in, 4 out]
                                n1136 = Array Size(array=w1636) -> (size(s)=w1633:i32[])
                                n1137 = Index Array(array=w1633, index=0) -> (element=w1635:i32)
                                n1138 = for {
                                N: w1635 -> [_]
                                tunnel: w1636 -> [w1645] mode=indexing
                                tunnel: [w1642] -> w1637 mode=indexing
                                n1139 = Index Array(array=w1645, index=0) -> (element=w1647:string)
                                n1140 = Index Array(array=w1645, index=1) -> (element=w1643:string)
                                n1141 = Decimal String To Number(string=w1647) -> (number=w1644:i32)  [unwired: 2 in, 1 out]
                                n1142 = Bundle(w1644, "String"=w1643) -> (w1642:cluster{i32, "String":string})  [unwired: 1 in]
                                }
                                n1143 = local write "program"(w1637) -> ()
                                }
                                frame #1 {
                                n1144 = local read "MOSL"() -> (w1651:i32)
                                n1145 = local read "MOS"() -> (w1652:T27)
                                n1146 = Index Array(array=w1652, index=w1651) -> (element=w1650:T37)
                                n1147 = Unbundle By Name(w1650) -> ("run number"=w1649:i32)
                                }
                                }
                                }
                              }
                            }
                          }
                        }
                      }
                    }
                  }
                  frame #2 {
                    n1148 = local write "run script"(FALSE) -> ()
                  }
                }
              }
            }
          }
          frame #12 {
            n1149 = case shown="참" "load script" {
              frame False {
              }
              frame True {
                n1150 = local read "Script path"() -> (w1666:path)
                n1151 = call "ファイルダイアログ2"("start path"=w1666) -> ("selected path"=w1667:path)  [unwired: 11 in, 3 out]
                n1152 = call-poly <vilib>:"Read From Spreadsheet File.vi"("delimiter (\\t)"="@@@", "format (%s)"="%s", "file path (dialog if empty)"=w1667) -> ("all rows"=w1659:string[][])  [unwired: 4 in, 4 out]
                n1153 = Array Size(array=w1659) -> (size(s)=w1662:i32[])
                n1154 = Index Array(array=w1662, index=0) -> (element=w1660:i32)
                n1155 = Strip Path(path=w1667) -> (stripped path=w1665:path, name=w1656:string)
                n1156 = local write "Script path"(w1665) -> ()
                n1157 = local write "file name"(w1656) -> ()
                n1158 = for {
                  N: w1660 -> [_]
                  tunnel: w1659 -> [w1671] mode=indexing
                  tunnel: [w1668] -> w1658 mode=indexing
                  n1159 = Index Array(array=w1671, index=0) -> (element=w1673:string)
                  n1160 = Index Array(array=w1671, index=1) -> (element=w1669:string)
                  n1161 = Decimal String To Number(string=w1673) -> (number=w1670:i32)  [unwired: 2 in, 1 out]
                  n1162 = Bundle(w1670, "String"=w1669) -> (w1668:cluster{i32, "String":string})  [unwired: 1 in]
                }
                n1163 = local write "load script"(FALSE) -> ()
                n1164 = local write "program"(w1658) -> ()
              }
            }
            n1165 = case shown="참" "save" {
              frame False {
              }
              frame True {
                n1166 = local read "program"() -> (w1679:cluster{"Cord":u16, "Option":string}[])
                n1167 = Array Size(array=w1679) -> (size(s)=w1682:i32)
                n1168 = for {
                  N: w1682 -> [_]
                  tunnel: w1679 -> [w1688] mode=indexing
                  tunnel: [w1684] -> w1681 mode=indexing
                  n1169 = Unbundle By Name(w1688) -> ("Cord"=w1687:u16, "Option"=w1685:string)
                  n1170 = Number To Decimal String(number=w1687) -> (decimal integer string=w1686:string)  [unwired: 1 in]
                  n1171 = Build Array(w1686, w1685) -> (w1684:string[])
                }
                n1172 = local read "Script path"() -> (w1675:path)
                n1173 = local write "save"(FALSE) -> ()
                n1174 = call "ファイルダイアログ4"("start path"=w1675) -> ("selected path"=w1676:path)  [unwired: 11 in, 3 out]
                n1175 = call-poly <vilib>:"Write To Spreadsheet File.vi"("delimiter (\\t)"="@@@", "2D data"=w1681, "file path (dialog if empty)"=w1676) -> ("new file path (Not A Path if cancelled)"=w1677:path)  [unwired: 5 in]
                n1176 = Strip Path(path=w1677) -> (stripped path=w1678:path)  [unwired: 1 out]
                n1177 = local write "Script path"(w1678) -> ()
              }
            }
          }
          frame #13 {
            n1178 = case shown="참" "SBR" {
              frame False {
              }
              frame True {
                n1179 = stacked-sequence {
                  frame #0 {
                    n1180 = local read "Control"() -> (w1706:T3)
                    n1181 = Unbundle By Name(w1706) -> ("HOT/COLD"=w1705:u16)
                    n1182 = case shown="1" w1705 {
                      frame 0, Default {
                      }
                      frame 1 {
                        n1183 = local read "Bias_LO_equip"() -> (w1711:T2)
                        n1184 = Unbundle By Name(w1711) -> ("POL"=w1709:u32)
                        n1185 = Rotate Right With Carry(2:w1709, 3:TRUE) -> (1:w1708:bool)  [unwired: 1 out]
                        n1186 = local read "SBR_Set"() -> (w1712:T25)
                        n1187 = Bundle By Name(cluster=w1712, "P/V         V/P"=w1708) -> (w1707:T25)
                        n1188 = local write "SBR_Set"(w1707) -> ()
                      }
                    }
                  }
                  frame #1 {
                    n1189 = local read "SBR_Set"() -> (w1713:T25)
                    n1190 = Unbundle By Name(w1713) -> ("PM        SP"=w1715:bool)
                    n1191 = local read "Control"() -> (w1714:T3)
                    n1192 = case shown="거짓" w1715 {
                      tunnel: w1714 -> [w1717 w1719]
                      tunnel: w1713 -> [w1716 w1718]
                      frame False {
                        n1193 = call "_SBR_mes_PM.vi"("SBR_Set"=w1716, "Control"=w1717) -> ()  [unwired: 6 in]
                      }
                      frame True {
                        n1194 = call "_SBR_mes_sp.vi"("SBR_Set"=w1718, "Control"=w1719) -> ()  [unwired: 6 in]
                      }
                    }
                  }
                }
                n1195 = local write "SBR"(FALSE) -> ()
              }
            }
            n1196 = case shown="참" "RF" {
              frame False {
              }
              frame True {
                n1197 = local read "RF"() -> (w1694:T26)
                n1198 = call "_RF.vi"("RF"=w1694) -> ()  [unwired: 11 in]
                n1199 = local write "RF"(FALSE) -> ()
              }
            }
            n1200 = case shown="참" "MPI-I" {
              frame False {
              }
              frame True {
                n1201 = local read "Bias_LO_equip"() -> (w1726:T2)
                n1202 = local read "Control"() -> (w1727:T3)
                n1203 = local read "MPI_I"() -> (w1728:T24)
                n1204 = call "_MPI_I_v2.vi"("MPI_I"=w1728, "Control"=w1727, "Bias_LO_equip"=w1726) -> ()  [unwired: 9 in]
                n1205 = local write "MPI-I"(FALSE) -> ()
              }
            }
            n1206 = case shown="참" "Move MPI toSSB" {
              frame False {
              }
              frame True {
                n1207 = local read "Control"() -> (w1703:T3)
                n1208 = Unbundle By Name(w1703) -> ("FreqLO"=w1702:dbl, "MPI offset(mm)"=w1701:dbl, "MPI COM"=w1697:refnum<visa-resource-name>)
                n1209 = local write "Move MPI toSSB"(FALSE) -> ()
                n1210 = call "_MPI_CALC.vi"("ofset (mm)"=w1701, "IF（GHｚ）"="IF frequency to SSB", "LO（GHｚ）"=w1702) -> ("SSB_pos(mm)"=w1698:dbl)  [unwired: 6 in, 2 out]
                n1211 = call "__MPI_move_pos_RS232c.vi"("pos"=w1698, "VISAリソース名"=w1697) -> ("®ì»ÝÊu"=w1699:string)  [unwired: 5 in]
                n1212 = local write "MPI present location"(w1699) -> ()
              }
            }
            n1213 = case shown="참" "Move MPI" {
              frame False {
              }
              frame True {
                n1214 = local read "MPI pos"() -> (w1724:dbl)
                n1215 = local read "Control"() -> (w1721:T3)
                n1216 = Unbundle By Name(w1721) -> ("MPI COM"=w1720:refnum<visa-resource-name>)
                n1217 = call "__MPI_move_pos_RS232c.vi"("pos"=w1724, "VISAリソース名"=w1720) -> ("®ì»ÝÊu"=w1723:string)  [unwired: 5 in]
                n1218 = local write "MPI present location"(w1723) -> ()
                n1219 = local write "Move MPI"(FALSE) -> ()
              }
            }
          }
          frame #14 {
            n1220 = case shown="참" "YIG measurement" {
              frame False {
              }
              frame True {
                n1221 = local read "Noise_YIG_tune_filter_control"() -> (w1732:T23)
                n1222 = local read "Bias_LO_equip"() -> (w1730:T2)
                n1223 = local read "Control"() -> (w1733:T3)
                n1224 = local write "YIG measurement"(FALSE) -> ()
                n1225 = call "_Noise_YIG3.vi"("Noise_YIG"=w1732, "Bias_LO_equip"=w1730, "Control"=w1733) -> ()  [unwired: 5 in]
              }
            }
          }
          frame #15 {
            n1226 = case shown="참" "Connect" {
              frame False {
              }
              frame True {
                # "@íú»"
                n1227 = stacked-sequence {
                  tunnel: [w1757 _ _ _] -> w1744
                  tunnel: [_ w1783 _ _] -> w1743
                  tunnel: [w1751 _ _ _] -> w1742
                  frame #0 {
                    n1228 = local read "WCA Pol"() -> (w1756:u16)
                    n1229 = local read "Bias_LO_equip"() -> (w1750:T2)
                    n1230 = call "__SISBias_init.vi"("Bias_LO_equip"=w1750) -> ("error out"=w1757:errorcluster, "Detected CAN Nodes."=w1748:string, "Bias_LO_equip 2"=w1749:T38)  [unwired: 4 in]
                    n1231 = Unbundle By Name(w1749) -> ("BiasModule"=w1755:u16)
                    n1232 = case shown="0, 기본" w1755 {
                      tunnel: w1756 -> [_ w1769]
                      tunnel: [w1760 w1768] -> w1754
                      tunnel: [w1759 w1767] -> w1753
                      frame 0, Default {
                        w1766 = 0
                        n1233 = local read "initial value"() -> (w1763:dbl[][])
                        n1234 = Index Array(array=w1763, index (row)=w1766, index (col)=0) -> (element=w1760:dbl)
                        n1235 = Index Array(array=w1763, index (row)=w1766, index (col)=2) -> (element=w1761:dbl)
                        n1236 = Index Array(array=w1763, index (row)=w1766, index (col)=1) -> (element=w1759:dbl)
                        n1237 = local write "Magnet Current Set"(w1761) -> ()
                        n1238 = local write "CLNA Monitor"(FALSE) -> ()
                        n1239 = local write "SISSetVolt"(w1760) -> ()
                        n1240 = local write "Offset"(w1759) -> ()
                      }
                      frame 1 {
                        n1241 = stacked-sequence {
                          tunnel: w1769 -> [w1771 w1777]
                          tunnel: [_ w1774] -> w1768
                          tunnel: [_ w1773] -> w1767
                          frame #0 {
                            n1242 = local read "Bias_LO_equip"() -> (w1772:T2)
                            n1243 = call "__wca_pol_sb.vi"("WCA Pol"=w1771, "Bias_LO_equip"=w1772) -> ("Bias_LO_equip 2"=w1770:T35)
                            n1244 = local write "Bias_LO_equip"(w1770) -> ()
                          }
                          frame #1 {
                            n1245 = local read "initial value"() -> (w1778:dbl[][])
                            n1246 = Index Array(array=w1778, index (row)=w1777, index (col)=0) -> (element=w1774:dbl)
                            n1247 = Index Array(array=w1778, index (row)=w1777, index (col)=2) -> (element=w1775:dbl)
                            n1248 = Index Array(array=w1778, index (row)=w1777, index (col)=1) -> (element=w1773:dbl)
                            n1249 = local write "Magnet Current Set"(w1775) -> ()
                            n1250 = local write "SISSetVolt"(w1774) -> ()
                            n1251 = local write "Offset"(w1773) -> ()
                          }
                        }
                      }
                    }
                    n1252 = local write "Detected CAN Nodes."(w1748) -> ()
                    n1253 = local write "Bias_LO_equip"(w1749) -> ()
                    n1254 = local read "SIScontrol"() -> (w1752:u16)
                    n1255 = call "__SISbias_Set.vi"("SIS@Mode"=w1752, "Offset"=w1753, "Set_V"=w1754, "Bias_LO_equip"=w1749) -> ("error out"=w1751:errorcluster)  [unwired: 7 in]
                  }
                  frame #1 {
                    n1256 = local read "Control"() -> (w1782:T3)
                    n1257 = Unbundle By Name(w1782) -> ("HOT/COLD"=w1781:u16)
                    n1258 = case shown="1" w1781 {
                      tunnel: [w1784 w1792] -> w1783
                      frame 0, Default {
                        n1259 = call <vilib>:"Clear Errors.vi"() -> ("error out"=w1784:errorcluster)  [unwired: 6 in, 1 out]
                      }
                      frame 1 {
                        # "ノミナルコールド"
                        n1260 = local read "Control"() -> (w1791:T3)
                        n1261 = Unbundle By Name(w1791) -> ("motor setting"=w1790:T33)
                        n1262 = Index Array(array=w1790, index=0) -> (element=w1787:T34)
                        n1263 = call "__move_motor2.vi"("Moving distance"=50, "motor setup"=w1787) -> ("error out"=w1792:errorcluster, "counter"=w1793:dbl)  [unwired: 2 in]
                        n1264 = Equal?(x=w1793, y=0.0) -> (x = y?=w1794:bool)
                        n1265 = case shown="거짓" w1794 {
                          tunnel: w1793 -> [w1798 _]
                          tunnel: w1787 -> [w1797 _]
                          frame False {
                            n1266 = Negate(x=w1798) -> (-x=w1796:dbl)
                            n1267 = call "__move_motor2.vi"("Moving distance"=w1796, "motor setup"=w1797) -> ()  [unwired: 2 in, 2 out]
                          }
                          frame True {
                          }
                        }
                        n1268 = local write "HOT/COLD"(TRUE) -> ()
                        n1269 = property on="HOT" class="Bool (엄격한)"("Value"=FALSE) -> ()  [unwired: 2 in, 2 out]
                      }
                    }
                  }
                  frame #2 {
                    n1270 = local read "i-v parameter"() -> (w1802:T17)
                    n1271 = local read "Control"() -> (w1803:T3)
                    n1272 = Unbundle By Name(w1803) -> ("GPIB_PM"=w1799:string)
                    n1273 = Unbundle By Name(w1802) -> ("frq(GHz)"=w1801:dbl, "avg"=w1800:i32)
                    n1274 = call "__SET_PM_1ch_E4419A.VI"("aveg"=w1800, "frq(GHz)"=w1801, "GPIB"=w1799) -> ()  [unwired: 5 in]
                  }
                  frame #3 {
                    n1275 = local read "Bias_LO_equip"() -> (w1807:T2)
                    n1276 = Unbundle By Name(w1807) -> ("LOModule"=w1806:u16)
                    n1277 = local read "LO_misc"() -> (w1805:T11)
                    n1278 = case shown="2, 기본" w1806 {
                      tunnel: w1805 -> [w1811 w1815 w1819]
                      tunnel: [w1808 w1812 w1816] -> w1804
                      frame 0, 5 {
                        n1279 = Bundle By Name(cluster=w1811, "LO REF multi"=3.0, "SG set pow"=20.0) -> (w1808:T11)
                      }
                      frame 2, Default {
                        n1280 = Bundle By Name(cluster=w1815, "LO REF multi"=3.0, "SG set pow"=0.0) -> (w1812:T11)
                      }
                      frame 1, 4, 6, 7 {
                        n1281 = Bundle By Name(cluster=w1819, "LO REF multi"=4.0, "SG set pow"=20.0) -> (w1816:T11)
                      }
                    }
                    n1282 = local write "LO_misc"(w1804) -> ()
                  }
                }
                n1283 = Merge Errors(w1744, w1743, w1742) -> (w1741:errorcluster)
                n1284 = case shown="에러" w1741 {
                  frame No Error {
                    n1285 = local write "Connected"(TRUE) -> ()
                  }
                  frame Error {
                    n1286 = local write "Connected"(FALSE) -> ()
                  }
                }
                n1287 = local write "error out"(w1741) -> ()
                n1288 = local write "Connect"(FALSE) -> ()
              }
            }
            n1289 = case shown="참" "add" {
              frame False {
              }
              frame True {
                n1290 = local read "Bias_LO_equip"() -> (w1740:T2)
                n1291 = Unbundle By Name(w1740) -> ("ObjHandle out"=w1738:u32, "Slave Node in"=w1739:cluster{"Address":i16, "Serial Number":i8[]})
                n1292 = call "Initialize FEMC.vi"("Slave Node in"=w1739, "Cartridge band"="Additional Cartridge band", "ObjHandle in"=w1738) -> ()  [unwired: 7 in, 2 out]
                n1293 = local write "add"(FALSE) -> ()
              }
            }
          }
          frame #16 {
            n1294 = case shown="참" "DISConnect" {
              frame False {
              }
              frame True {
                n1295 = local read "Bias_LO_equip"() -> (w1827:T2)
                n1296 = Unbundle By Name(w1827) -> ("BiasModule"=w1826:u16)
                n1297 = stacked-sequence {
                  tunnel: w1826 -> [w1830 w1837 _ _]
                  frame #0 {
                    n1298 = case shown="1" w1830 {
                      frame 0, Default {
                        n1299 = local read "Bias_LO_equip"() -> (w1833:T2)
                        n1300 = Unbundle By Name(w1833) -> ("GPIB_DMM (SIS I)"=w1832:string)
                        n1301 = GPIB Write(0:w1832, 1:"DISP ON") -> ()  [unwired: 3 in, 2 out]
                      }
                      frame 1 {
                        n1302 = local read "error out"() -> (w1834:errorcluster)
                        n1303 = local read "Bias_LO_equip"() -> (w1836:T2)
                        n1304 = Unbundle By Name(w1836) -> ("ObjHandle out"=w1835:u32)
                        n1305 = call "WCA_CAN_close.vi"("ObjHandle in"=w1835, "error in (no error)"=w1834) -> ()  [unwired: 13 in, 1 out]
                      }
                      frame 99 {
                      }
                    }
                    n1306 = local write "Connected"(FALSE) -> ()
                  }
                  frame #1 {
                    n1307 = local read "WCA Pol"() -> (w1838:u16)
                    n1308 = case shown="0, 기본" w1837 {
                      tunnel: w1838 -> [w1849 _]
                      frame 1 {
                        n1309 = local read "SISSetVolt"() -> (w1846:dbl)
                        n1310 = local read "Magnet Current Set"() -> (w1842:dbl)
                        n1311 = local read "initial value"() -> (w1848:dbl[][])
                        n1312 = local read "Offset"() -> (w1845:dbl)
                        n1313 = Replace Array Subset(array=w1848, new element=w1846, index (row)=w1849, index (col)=0) -> (w1841:dbl[][])
                        n1314 = Replace Array Subset(array=w1841, new element=w1845, index (row)=w1849, index (col)=1) -> (w1840:dbl[][])
                        n1315 = Replace Array Subset(array=w1840, new element=w1842, index (row)=w1849, index (col)=2) -> (w1839:dbl[][])
                        n1316 = local write "initial value"(w1839) -> ()
                      }
                      frame 0, Default {
                        w1850 = 0
                        n1317 = local read "SISSetVolt"() -> (w1858:dbl)
                        n1318 = local read "Magnet Current Set"() -> (w1854:dbl)
                        n1319 = local read "initial value"() -> (w1860:dbl[][])
                        n1320 = local read "Offset"() -> (w1857:dbl)
                        n1321 = Replace Array Subset(array=w1860, new element=w1858, index (row)=w1850, index (col)=0) -> (w1853:dbl[][])
                        n1322 = Replace Array Subset(array=w1853, new element=w1857, index (row)=w1850, index (col)=1) -> (w1852:dbl[][])
                        n1323 = Replace Array Subset(array=w1852, new element=w1854, index (row)=w1850, index (col)=2) -> (w1851:dbl[][])
                        n1324 = local write "initial value"(w1851) -> ()
                      }
                    }
                  }
                  frame #2 {
                    n1325 = local read "End of the equipment\nLOCAL"() -> (w1861:bool)
                    n1326 = case shown="참" w1861 {
                      frame False {
                      }
                      frame True {
                        n1327 = FindLstn(5:32, 6:i32[] [24, 25, 18, 13, 22]) -> (3:w1862:i16[])  [unwired: 2 in, 3 out]
                        n1328 = EnableLocal(3:w1862) -> ()  [unwired: 2 in, 2 out]
                      }
                    }
                  }
                  frame #3 {
                    n1329 = local read "Control"() -> (w1866:T3)
                    n1330 = Unbundle By Name(w1866) -> ("MPI COM"=w1865:refnum<visa-resource-name>)
                    n1331 = VISA Close(VISA resource name=w1865) -> ()  [unwired: 1 in, 1 out]
                  }
                }
                n1332 = local write "DISConnect"(FALSE) -> ()
              }
            }
            n1333 = case shown="참" "CAN reset" {
              frame False {
              }
              frame True {
                n1334 = local read "Bias_LO_equip"() -> (w1824:T2)
                n1335 = local read "error out"() -> (w1822:errorcluster)
                n1336 = local write "CAN reset"(FALSE) -> ()
                n1337 = call "WCA_CAN_reset.vi"("error out"=w1822, "Bias_LO_equip"=w1824) -> ("Bias_LO_equip 2"=w1823:T35)  [unwired: 9 in]
                n1338 = local write "Bias_LO_equip"(w1823) -> ()
              }
            }
          }
        }
      }
    }
  }
  "revision" <- "2018 8/8 Translate Japanese to English\n\n2017 Mix11 English Record support\n\n2013 6/13 LOHarmonics to script\n\n2013 5/25 GC file completed after measurement\n\n2012 8/15 JC ªÈ£Í£á£çªÎ«Õ?«¤«ëÙ£ªË£Ì£Ïñ²÷î?\n2012 8/15 £Ê£ÃªÈ£É£í£á£çªÎ«Õ?«¤«ëÙ£ªË£Ì£Ïñ²÷î?ªòìýªìªÊª¤\n\n\n2012?7/10 £É£Ö??£Õ£Ô£Ï£³ªÎª·ªçªÔªíï³?ªòàâïÒÊ¦?ªË«Ç«Õ«©«ë«ÈªÏ0.2ªËª·ªÆªªª­£Ö£ç£á£ðªÎî¸ª¤ªâªÎªÏ0.15ªËª¹ªë¡£\n£Ì£Ï£Ï£Ð£ÔªÎ?ÑÑÝÂùÜªÀªÈ?ðà?Ê¥ª·ªÊª¤ãÁªËÙýð¹ª¢ªê¡¢£Ã£Ã?07?11ö´ïÒãÁ?ª·ªÐªéª¯ª¹ª¤?ª×ªÇ£Ó£É£Ó£Â£é£á£ó«»«Ã«Èª¹ªë¡£\n£Ç£Ã«×«í«°«é?ªÇö´ïÒüÞ?3üÞì¤ß¾ªÇ?ªáªëÝ»ÝÂªÎ÷÷?ªòªÁªçªÃªÈ?ª¨ªë\n\n\n2012 3/14 IV-auto3ªÇª·ªãªÔªíï³?£°£®£²£í£Öì¤ß¾£½£¾£°£®£±£µ£í£Öì¤ß¾ªË?ÌÚ\n£¨ñ²÷î?ªÎÍÔª¤ªÈª³ªíªÇó¬ª¬ÓÞª­ª¹ª®ªë£©\n\n2012 3/2  WCAPOLªÞªïªêáóïá£¨£Ä£Ó£Â«â?«ÉªÀª±ªËª·ª¿£©\n\n\n2012 2/10 ?«Ò??Ö§?£Ï£îûù\n\n2012 1/26 «¹«¯«ê«×«È?£Ì£Ï£Ð£á£ò£á£íªË£Ð£Ï£ÌªòõÚÊ¥\n???????£Ð£Ï£Ìªò?ÌÚª·ª¿ªÈª­ªË£Ã£ï£î£ô£ò£ï£ìªÎ£Ó£å£ô£Ó£É£Ó£Ö£Ï£Ì£ÔÔõªËÚãç±?\n\n2012 1/18  SBRÍªß©?ÊÛæ¶SBRªòõÚÊ¥\n\n2012 1/9 «¹«¯«ê«×«È?Text Inputáóïá¡¢ôøÑ¢ö·ª¬ù±é©ªË\n???????????Cartridge SNõÚÊ¥\n\n2012 1/8 «¹«¯«ê«×«È?FileTimeStampõÚÊ¥\n\n2012 1/7  «¹«¯«ê«×«È?SP spriousõÚÊ¥\n\n2012?1/7  Calc IF?outªÎ«¯«é«¹?ªÇNS£ßENRªÎ«Ç«£«ì«¯«È«êªò\nInputCable¡¢NS_AMPªÎ«Ç«£«ì«¯«È«êªËª¹ªëªèª¦ªË?ÌÚ£¨ú°à°«Ñ?«³«ó¡¢IFBOXª¬?ªïªÃª¿ãÁªËNS_ENRªÀª±àÔ?ª·ªÊªªª¹£©\n        \n\n2011 11/20 LO Harmonic  õÚÊ¥?CrossTalkªÇSIS«Ð«¤«¢«¹ªò£µ£íVªË\n\n2011 11/14 «¹«¯«ê«×«ÈPolÞÅéÄãÁªËWCAPolªâÌÚãæª¹ªëªèª¦ªËª·ª¿\n\n2011 11/05 CLNA«Ð«¤«¢«¹«¹«¤?«×¡¢ª¤ªÃª¿ªó£°V£°MAªËª¹ªë\n??????«¹«¯«ê«×«ÈExcel?Set?CellªÏ£°£¬£°ª¬A1?£¨ì¤îñíÂà÷ª·ª¿«¹«¯«ê«×«ÈªÏìéËÁªºªÄá´ªÊª¯ª¹ªë£©\n\n2011 11/04 Labview2011 ver «ì??«ÈíÂà÷«Ä?«ëÞÅéÄ\n\n2011 10/29  «¹«¯«ê«×«È?SetcellªËPolõÚÊ¥?Make3DªÎ«Õ?«¤«ëÙ£áóïá\n\n2011 10/25?«¹«¯«ê«×«È?Mix10ParamsªË«¹«¯«ê«×«È«Õ?«¤«ëÙ£õÚÊ¥ \n\n2011 10/14 «¹«¯«ê«×«ÈPolSetªÎªÈª­ôøÑ¢ö·ª«ªéSetMagÔõªò?ÌÚ\n????PM?TEMP?PolªË«¹«Ú?«¹ð¶ËÛ\n????LOParamsªò?PAA?PABªÎ?ªÓª«ªéP0?P1ªÎªÊªéªÓªË¡¢ª½ªÎý­ªÎWCA«Ñ«é«á??ªÏPAA?PABªÎ?ªÓ\n\n2011 10/02 «¹«¯«ê«×«ÈSetcell áóïá?make3Ddataªâáóïá£¨«Ç??«Ç«£«ì«¯«È«êªË?ßÀªòÜÁðí£©\n\n2011 9/28?«¹«¯«ê«×«ÈSP?ÌÚ?VBWªâàâïÒÊ¦?ªË\n \n2011 9/26 SP single dataªÉªê¡¢«¹«¯«ê«×«ÈªËpoint comment2õÚÊ¥\n \n\n2011 9/9 2pol ö´ïÒéÄªË«¹«¯«ê«×«ÈìéÝ»áóïá\n\n2011 9/8 control ªÎDB«Ñ«¹ªòmixer param ªË?ÌÚ\n\n2011 9/7 «¹«¯«ê«×«ÈMake£³DgraphíÂà÷\n\n2011 8/31 SIS setªÎªÈª­ªËPAVÛÕÖªªòÌÚãæ?SISï³??OffsetªâÌÚãæ\n\n2011 8/26 \n¡ÜLO PAMP?ªÈ ?£Ã£Ì£Î??ªÏ£×£Ã?ªÎãÁ£Ð£°£¬£Ð£±ªÈªâªËàâïÒ\n¡ÜBias_LO_equip LOModuleªËÊ¦?£Ì£Ï?£Ô£Ôªâùßªáªëª³ªÈªËª·ª¿ªÎªÇ¡¢\n£Ì£Ï?£Ï£Ð£Ô?Ìõªòáóïá \n¡Ü£Ã?£Î«ê«»«Ã«È?õÚÊ¥ \n\n2011 8/3 «¹«¯«ê«×«ÈªÇ«Õ«é«Ã«¯«¹?Ìõ\n????CAN«Î?«ÉªËMIX10paramsì£?ÌÚ\n\n2011 7/28  «¹«¯«ê«×«ÈªË«·«ã«Ô«í?Ìõ?«Õ?«¤«ëÙ£ªòLogªËßöª¯«³?«ó«ÉõÚÊ¥\n2011 7/27  «·«ã«Ô«í?Ìõáóïá¡¢í»ÔÑûù\n\n2011 7/6 «¨«¯«»«ë?Ìõáóïá\n2011 7/5 ª¤ª¯ªÄª«áóïá\n\n2011 7/1 Calc IF output ?Ö§?õÚÊ¥\n\n2011 6/29 Cross Talk õÚÊ¥\n\n2011 6/21 MPIð¤åÙªòGPIBªÇú¼ªÃªÆª¤ª¿ªé«¨«é?Òý?ªÊªÎªÇRS-232CªÇð¤åÙª¹ªëªèª¦ªËª·ª¿\n\n\n2011 6/18 «¹«¯«ê«×«È?«¨«¯«»«ë?Ìõ\n                                 ìé?jump«³?«ó«ÉõÚÊ¥\n\n2011 6/16  «¹«¯«ê«×«È?fileÙ£ªò«µ«Ö£Ö£éûù\n\n2011 6/12 «¹«¯«ê«×«È?set loop num\n2011 6/12 «¹«¯«ê«×«È?LO Sweep\n\n2011 5/15 «¹«¯«ê«×«ÈLOPOPT?Read LO param??ÌõíÂà÷\n\n2011 5/13 WCA LO??ªÇ«³«ó«È«í?«ëª·ª¿ªÈª³ªíªÎ?×âáóïá\n\n2011 4/28 RoomTemp Helth check \n               SPªâP£°?P1ï·ªêôðª¨ªÇ«Ç??ªòªÈªëªèª¦ªËáóïá\n\n2011?02?15?YIGSave«Õ«©??«Ã«È?ÌÚ\n\n2011/02/6  SetMixerParamõÚÊ¥\n\n\n2011/02/4 GainCompõÚÊ¥ Read MixCLNAParamõÚÊ¥?£¨LOªÏªÞªÀ£©\n \n2011/01/27 «¹«¯«ê«×«È«µ«Ö«×«í«°«é?áóïá\n\n2011/01/20 IFBOXñ²ªêªòáóïá\n\n2011 1/12 Mix10ªË?ÌÚ?«¹«¯«ê«×«È?«µ«Ö«¹«¯«ê«×«È?\n\n12/10 «¹«¯«ê«×«ÈLO«»«Ã«ÈªÎáóïá «â??«ê«»«Ã«È\n\n10/17 «¹«¯«ê«×«ÈªËAllan6£¨?Óø«Ç??ö¢Ôð£©õÚÊ¥?\n\n10/3 SPªËSISVªÇªÎH/CõÚÊ¥\n\n9?7?PLL?GUNNªÄª¤ª«\n\n9/4 YIGõÚÊ¥\n\n8/29 ControlªËHOT/COLDªòõÚÊ¥¡¢SBRö´ïÒãÁªÇªâIVSPDSB?ëåö´ïÒ\n\n8/24 MPIðÚªß?ªß\n\n8/13 WCA LO?Ö§?YTO?ªßö¢ªêáóïá¡¢Lock«ë??«óªÎÌ¸òÁª·£¨IFPªòõÌîêûùª·ªÆª«ªéLock£©\n\n8/12 CANôøÑ¢ûù«¨«é?ãÁªÎ?×âªò?ûù£À««?«È«ê«Ã«¸\n«¤«Ù«ó«È«¹«È«é«¯?«ãªòÓÞøëïÚ×â\n\n\n8/11 LOPOPT ªÎTCTHªòControlª«ªéªË?ÌÚ\n????«¹«¯«ê«×«ÈLOFreqGUNNªÇñ²÷î?ªòControlªË\n\n8/9 «¹«¯«ê«×«ÈªËIVNOLOªòõÚÊ¥¡¢Log«Õ?«¤«ëªËCommentªòªÄª±ªëªèª¦ªË£À?«¯«µö´ïÒÍ§\n\n8/6 «·«ã«Ô«í«¹«Æ«Ã«×«×«í«°«é?¡¢ª¤ªÃª¿ªó0ªË«»«Ã«Èª¹ªëªÈªèª¤Êïª¸£¿£À?«¯«µö´ïÒ\n«·«ã«Ô«í«¹«Æ«Ã«×«×«í«°«é?ÊÛæ¶÷úIF£ðªÎªßö´ïÒªÇ\n\n8/5  8/4áóïáÝÂªÎ«Ð«°áóïá£À?«¯«µö´ïÒ\n?LOSWEEPªÎB10LabãÁªÎ«Õ?«¤«ëÜÁðíáóïá\n\n8/4 IV-TrxªÇö´ïÒý­õÌî¸?ëå?ÓøªËVset\nContorolªËoffseÔõªÎõÚÊ¥IVª«ªéVsetÔõªÎÞûð¶\n\n\n8/2 «Ð«¤«¢«¹«â«¸«å?«ëôøÑ¢ûùªÎ«Ð«°áóïá\n?\n\n\n\n7/31\n?I-V«¹«¤?«×ªÎStartªÇ0.5sÜÁò¥\n?«¹«¯«ê«×«ÈªÇªÎö´ïÒªÇªÏ?ãÆ«Ñ«Í«ëªòÌÚãæª·ªÊª¤£¨«Õ?«¤«ëÙ£?óþ£©\n?«¹«¯«ê«×«È«í«°«Õ?«¤«ë\n?Bias«â«¸«å?«ë?LO«â«¸«å?«ëª¬ªÊª¤íÞùê99ªÇôøÑ¢ûù«â«Ë?ªòú¼ªïªÊª¤\n?SUB«×«í«°«é?ªÇªÏÚ±?óþ¡¢«¹«¯«ê«×«È«Ç«Ð«Ã«°éÄ\n\n\n7/30 \n?«Ò???ð¤åÙªÇ«Õ?«¤«ëÜÁðíõÚÊ¥\n£À««?«È«ê«Ã«¸\n\n7£®27?\n?yig?ãá?ñ²÷î?àâïÒõÚÊ¥¡¹?\n?GetSIS ªÎB10«Ð«¤«¢«¹\n£À?«¯«µö´ïÒÍ§"
